vi "UNITEST MAIN v01.3.vi"() -> ()   [LabVIEW 2025]
uses:
  controls/LAB-IQ UI Data.ctl
  HEAVE vi's/Heave Write enum.ctl
  487e97dd-ad82-4ea8-9260-f35915b83a37.vi
  fdf22e40-24ec-4bd6-b058-052306f15f2c.vi
  02c5850b-52e8-4ed5-91f8-6f0ad62f4994.vi
  1223eb78-e4c4-4b69-bf80-185c82055158.vi
  e5651a45-6a49-4a3f-b503-ff1eaf449b4a.vi
  support/Message Queue/Enqueue Message (Single).vi
  <vilib>/Utility/error.llb/Error Cluster From Error Code.vi
  <vilib>/ErrorRing/Error Ring.xnode
  support/Message Queue/LAB-IQ Message Queue.lvlib
  support/User Event - Stop/LAB-IQ User Event - Stop.lvlib
  d081153b-36ca-4bc4-8478-749476f82ba4.vi
  HEAVE vi's/Heave Right enum.ctl
panel:
  in  "Checkbox":bool
  in  "seconds to wait":dbl=0.0001 format="%#_6p"
  out "error out":errorcluster
  in  "error in (no error)":errorcluster
  out "Heave and Surge Read":string
  in  "min_finetune_floor":dbl=0.15
  in  "min_deadband_floor":dbl=0.05
  in  "fine_tune_pct":dbl=100.0
  out "Start Test Temp":bool
  in  "STOP":bool
  in  "AppLoadSeq scratch":bool
  out "Pulse delta":dbl
  in  "Fine Tune Zone":dbl=10.0
  in  "PID Delay (sec)":dbl=1.0 format="%#_6p"
  in  "Max_pos_limit":dbl=50000000.0
  in  "Min_pos_limit":dbl
  in  "i_limit":dbl=10.0
  in  "Max Step Linit":dbl=10.0
  in  "Init Step":dbl=10.0
  in  "pct_scale":dbl=100.0
  in  "Deadband":dbl=0.1
  in  "Kd":dbl
  in  "Ki":dbl
  in  "Kp":dbl=1.0
  out "Current Position":dbl
  in  "Set Load":dbl
  in  "Current Load":dbl
  in  "Manual Write Heave & Surge":bool
  out "Heave and Surge Write":string
  in  "Heave Loop Delay":dbl
  in  "Heave PID Speed":dbl=15.0
  in  "Surge Jog Speed":dbl=1.0 format="%.4f"
  in  "Heave Jog Speed":dbl=15.0
  in  "SPARE 4":u8
  in  "SPARE 3":u8
  in  "SPARE 2":u8
  in  "SPARE 1":u8
  out "Spare 15":u8
  out "Spare 14":u8
  out "Spare 13":u8
  out "Spare 12":u8
  out "Spare 11":u8
  out "Spare 10":u8
  out "Spare 9":u8
  out "Spare 8":u8
  out "Spare 7":u8
  out "Spare 6":u8
  out "Spare 5":u8
  out "Spare 4":u8
  out "Spare 3":u8
  out "Spare 2":u8
  out "Spare 1":u8
  out "Node Id":u8
  out "Read Heave Temp":bool
  out "fwMinor":u8
  out "fwMajor":u8
  out "faultCode":u16
  out "SURGE POSE":sgl format="%#.6f"
  out "HEAVE POSE":sgl format="%#.6f"
  out "Homed":u8
  out "State":u8
  out "Ack ID":u16
  in  "SPEED":sgl=10000.0
  in  "Distance":sgl=10000.0
  in  "Mode Command":u8=2
  out "Sequence ID":u16
  out "error out Read":errorcluster
  out "error out Write":errorcluster
  out "Heave and Surge Read":string
  out "Load Cell Temp":bool
  in  "Stop Scratch":bool
  in  "Enter Fixed SRR 2":dbl min=0.0 max=0.0 format="%.3f"
  in  "E.Velocity 2":bool=TRUE caption="SRR"
  out "Message":string="Load Entered is out of range!!!"
  in  "Tab Control 3":T1(tab)
  in  "Tab Control 5":enum32{""}(tab)
  in  "Tab Control 14":T2(tab)=enum."Motor Load"
  in  "Ramp MulFac":dbl=2.0
  in  "pulses LoadDiffRamp(2..10)":dbl=9.0
  in  "PulseControlRamp(diff<=3N)":dbl=5.0 min=1.0 max=1000.0 step=1.0 format="%#.1f"
  in  "SetLoadDeadband(%) Load(0-10N)":dbl=0.1 min=0.0001 max=100.0 step=0.0001 format="%#.6f"
  in  "PID gains out delay (microForce)":T3={"proportional gain (Kc)"=300.0, "integral time (Ti, min)"=0.00011, "derivative time (Td, min)"=0.0} {"derivative time (Td, min)" format="%.3f"; "integral time (Ti, min)" min=1e-05 max=100.0 step=1e-06 format="%.6f"; "proportional gain (Kc)" format="%.3f"}
  in  "Ramp":bool
  in  "Gain 2":dbl=0.016
  in  "pulses LoadDiff(2..10)":dbl=10.0
  in  "pulses LoadDiff(11..50)":dbl=40.0
  in  "PulseControl(diff<=3N)":dbl=1.0 min=1.0 max=1000.0 step=1.0 format="%#.1f"
  out "SetLoadDeadband(%)  2":dbl=1.0 min=0.001 max=100.0 step=0.001 format="%#.6f"
  in  "Dummy Run":bool
  out "Vertical load (N)":dbl format="%#.3f"
  in  "AutoTune":bool
  in  "Offset  3":dbl=1.5
  in  "apply load":bool
  in  "Enter ByPass Load":dbl
  in  "reinit 3":bool=TRUE
  in  "output range delay":cluster{"output high":dbl, "output low":dbl}={"output high"=100.0, "output low"=-100.0} {"output low" format="%.2f"; "output high" format="%.2f"}
  in  "PID gains out delay":T3={"proportional gain (Kc)"=30.0, "integral time (Ti, min)"=0.00101, "derivative time (Td, min)"=0.0} {"derivative time (Td, min)" format="%.3f"; "integral time (Ti, min)" min=1e-05 max=100.0 step=0.0001 format="%.4f"; "proportional gain (Kc)" format="%.3f"}
  in  "Bypass Load":bool
  in  "pulsesSent":dbl=200.0
  out "pulses":dbl
  out "actpid":dbl
  out "gFF Rot 7":cluster{dbl, dbl, dbl}(graph)
  in  "pulses LoadDiff(21..1000)":dbl=40.0
  in  "Delay":dbl=1.5 min=0.001 max=5.0 step=0.001 format="%#.6f"
  in  "deadband":dbl=0.2
  in  "Tab Control 26":enum32{"Page 1", "Page 2"}(tab)
  in  "ClearAll":bool
  out "Mz(Nm)":dbl[](array[numeric])
  out "My(Nm)":dbl[](array[numeric])
  out "Mx(Nm)":dbl[](array[numeric])
  in  "Save Dwell":dbl=0.015 caption="Save Dwell (sec)" min=0.0 max=5.0 step=0.001 format="%.3f"
  out "Mx":dbl[](graph)
  out "My":dbl[](graph)
  out "Mz":dbl[](graph)
  out "Fx(N)":dbl[](graph)
  out "Fy(N)":dbl[](graph)
  out "Fz(N)":dbl[](graph)
  in  "ZeroAll":bool
  in  "Acq Delay (ms)":dbl=10.0
  in  "Burst Delay (ms)":dbl=10.0
  out "model":string
  out "SN":i32
  out "FFx(N)":dbl[](array[numeric])
  in  "Sensor IP":string="192.168.1.100"
  in  "Port":i32=8080
  out "FFy(N)":dbl[](array[numeric])
  out "Load(N)":dbl[](array[numeric])
  out "AE":bool
  in  "delete Handle":bool
  in  "Create Handle":bool=TRUE
  out "ft_data":dbl[](array[numeric])=[1.0, 1.0, 1.0, 1.0, 1.0, 1.0]
  out "ft_range":dbl[](array[numeric])=[1.0, 1.0, 1.0, 1.0, 1.0, 1.0]
  in  "stop 6":bool
  out "running_flag":bool
  out "ft_udp_handle":i32
  out "get-data-return":i32
  out "get-range-return":i32
  out "zero-return":i32
  out "filter-return":i32
  out "initial-return":i32
  out "deleteHandle-result":i32
  in  "Tab Control 19":enum32{"Platform COM", "Config ", "DevInfo"}(tab)=enum."Config "
  in  "SAMPLES":dbl=100.0
  in  "Re-initilaize":bool
  in  "Filter ON/OFF":bool=TRUE
  in  "TracHomeSurgeOffsetCounts 10MM":dbl=505100.0
  in  "TracHomeSwayOffsetCounts 10MM":dbl=1432.0
  in  "Acoustic Emission:":dbl=1.0 min=0.0001 max=200.0 step=0.0001 format="%.4f"
  in  "Apply Filter (FF)":bool
  in  "Filter% 2":dbl=50.0 min=50.0 max=100.0 step=0.1 format="%.1f"
  in  "Apply Filter (Load)":bool=TRUE
  in  "Filter%":dbl=80.0 min=50.0 max=100.0 step=0.1 format="%.1f"
  in  "Sway distance (mm)":dbl=245.0
  in  "Surge distance (mm)":dbl=370.0
  in  "DataSavingLoopDelay(ms)":dbl=15.0
  in  "SAVE  2":bool
  in  "Enter Distance":bool caption="Enter Counts"
  in  "Sway Counts:":dbl=100.0 min=0.0 max=100000000.0 step=1.0 format="%.2f"
  in  "Distance (mm): 3":dbl=100.0 caption="Distance (mm):" min=0.0 max=1500.0 step=0.001 format="%.5f"
  in  "Surge Counts:":dbl=100.0 min=0.0 max=100000000.0 step=1.0 format="%.1f"
  in  "Distance (mm): 2":dbl=100.0 caption="Distance (mm):" min=0.0 max=1500.0 step=0.0001 format="%.3f"
  in  "Distance (mm):":dbl=100.0 min=0.0 max=1500.0 step=0.001 format="%.5f"
  in  "Heave Counts:":dbl=100.0 min=0.0 max=100000000.0 step=1.0
  in  "LRMHomeSurgeOffsetCounts":dbl=307197.0
  in  "LRMHomeSwayOffsetCounts":dbl=26880.0
  in  "TracHomeSurgeOffsetCounts 20MM":dbl=505100.0
  in  "TracHomeSwayOffsetCounts 20MM":dbl=1432.0
  in  "RotHomeSwayOffsetCounts":dbl=14656.0
  in  "RotHomeSurgeOffsetCounts":dbl=311465.0
  in  "Heave distance":dbl=340.0
  out "Zmm":dbl=1600.0
  out "Heave Pulses/mm":dbl=1600.0
  out "Surge Pulses/mm":dbl=1600.0
  out "Sway Pulses/mm":dbl=320.0
  in  "Heave Pitch":dbl=4.0
  in  "Surge Pitch":dbl=3.0
  in  "Sway Pitch":dbl=2.0
  in  "Heave PPR":dbl=6400.0
  in  "Surge PPR":dbl=6400.0
  in  "Sway PPR":dbl=6400.0
  in  "GUI":T4(tab)
  in  "Platform Settings":bool caption="Password"
  in  "Configure":bool caption="Password"
  in  "Home":bool caption="Password"
  in  "EXIT":bool
  in  "Analysis":bool caption="Password"
  in  "service 2":bool caption="Password"
  in  "MainPage":T5(tab)=enum."HOME"
  in  "Select Load Head":bool
  in  "Notes :":string
  in  "FILE":string
  in  "Sample ID :":string
  in  "Operator ID :":string
  in  "Operator Name :":string
  in  "Auto":bool caption="Power Status"
  out "mm/s  Surge":dbl=7.0 caption="Jog" min=0.001 max=50.0 step=0.0001 format="%.2f"
  in  "Update Surge Speed":bool
  out "Drive Error":string
  in  "Disable Axis Jog Soft Limits":bool
  out "mm/s  Sway":dbl=7.0 caption="Jog" min=0.001 max=50.0 step=0.0001 format="%.2f"
  out "Sway and Surge COM Status":bool=TRUE caption="Load COM Status"
  out "Heave COM Status":bool=TRUE caption="Load COM Status"
  in  "Enable Platform":bool
  in  "Surge Forward Main":bool
  in  "Surge Backward Main":bool
  in  "Sway Right Main":bool
  in  "Sway Left Main":bool
  in  "Heave Down Main":bool
  in  "Heave Up main":bool
  in  "Update Sway Speed":bool
  in  "Update Heave Speed":bool
  out "mm/s Heave":dbl=7.0 caption="Jog" min=0.001 max=30.0 step=0.0001 format="%.2f"
  in  "mm/sec":dbl=1.0 caption="Jog" min=0.001 max=50.0 step=0.001 format="%.2f"
  in  "mm":dbl=0.001 caption="Jog" min=0.001 max=200.0 step=0.0001 format="%#.3f"
  in  "Surface Analysis":bool
  in  "Imaging":bool
  in  "Image Analysis":bool
  in  "Post Analysis":bool
  in  "SSP 0.75":bool
  in  "SSP 0.5":bool
  in  "SSP 0.3":bool
  in  "Warning":enum32{"Page 2"}(tab)
  in  "gui GIF":enum32{"Check", "Deca", "kilo", "Micro"}(tab)
  out "Communication is established":bool=TRUE caption="Load COM Status"
  in  "Reference Sample":u16(ring) items=["None", "Brass", "Aluminium", "Mild Steel"]
  out "Load Cell Communication Slide":u8(slide)=1 min=1 max=10 step=1 scale=0.0..10.0
  in  "com 3":bool
  out "com":bool
  out "DecaForce COM Status":bool caption="Load COM Status"
  in  "Loading Mode":u16(ring) items=["Constant", "Ramp", "Steps", "Indentation"]
  in  "Enter the CoF Trip":dbl=1.0
  in  "Enter the Friction Force Trip":dbl=520.0 min=500.0 max=500.0 step=1.0 format="%#.1f"
  in  "Enter the Normal load Trip":dbl=520.0 min=500.0 max=500.0 step=0.001 format="%.3f"
  in  "KiloForce":bool
  in  "DecaForce":bool
  in  "MicroForce":bool
  in  "LHBack":bool
  in  "LHNext":bool
  in  "Load Selection":T6(tab)
  in  "Enter the Load  (N)":dbl=2.0 min=2.0 max=50.0 step=0.1 format="%#.4f"
  in  "Enter the Final Load (N)":dbl=1.0 min=0.0 max=500.0 step=1.0 format="%#.0f"
  in  "Update":bool
  in  "Enter the Loading Rate (N/min)":dbl=60.0 min=60.0 max=1200.0 step=0.1 format="%.2f"
  out "Warning 2":bool
  in  "Stribeck Table  For loading":string[][](table)=[["", "", ""], ["", "", ""], ["", "", ""], ["", "", ""]]
  in  "Stribeck table":bool
  in  "seq":bool=TRUE
  in  "Clear 3":bool
  in  "Indentation":string[][](table)=[["Detection", "5", "2"], ["Unload", "0", "5"], ["Load", "10", "2"], ["Unload", "0", "5"], ["Detection", "5", "2"], ["Unload", "0", "5"]]
  in  "Multipoint":bool caption="Singlepoint"
  in  "AppLoad 4":bool
  in  "zNL":bool
  out "NL disp":dbl caption="Normal Load ( N )" min=-2000.0 max=2000.0 step=0.0001 format="%.1f"
  in  "Traction":bool
  in  "Surge Forward MM":bool
  in  "Surge Backward MM":bool
  in  "M3 Image":enum32{"Page 1", "Page 2"}(tab)
  in  "String 39":string="Jog heave to bring the upper sample closer to the lower sample within 1mm."
  in  "Sway Left MM":bool
  in  "Sway Right MM":bool
  in  "Disable Axis Jog Soft Limits":bool
  in  "mm":dbl=0.001 caption="Jog" min=0.001 max=5.0 step=0.0001 format="%#.3f"
  in  "Heave Down MM":bool
  in  "Heave Up MM":bool
  in  "Wear Track Diameter (mm)":dbl=5.0 caption="Wear Track Diameter (mm):" min=1.0 max=30.0 step=1.0 format="%.2f"
  in  "Set WTD":bool
  in  "HomeScratch":bool
  in  "HomeRot":bool
  in  "PlaceModule":bool
  in  "Motion Mode:":u16(ring) items=["Uniform Rotation", "Angular Oscillation", "Stribeck ", "Steps"]
  in  "LR Sway":bool
  in  "Rot Hor":bool
  in  "Rot Ver":bool
  in  "Scratch":bool
  in  "LR Cam":bool
  in  "MMBack":bool
  in  "MMNext":bool
  in  "Rotary Module Selection":T7(tab)
  in  "SPEED SELECTION :":enum32{"Speed in RPM", "Speed in m/sec"}(radio)=enum."Speed in m/sec"
  in  "TEST SELECTION":enum32{"Time", "Cycle"}(radio)
  in  "Enter the Speed(mm/sec)":dbl=1.0 min=0.1 max=10.0 step=0.1 format="%.1f"
  in  "Enter the Speed(RPM)":dbl=45.0 min=5.0 max=300.0 step=1.0
  in  "Enter the Frequency (Hz)":dbl=1.0 min=0.1 max=10.0 step=0.1 format="%.1f"
  in  "Enter the Angle (Deg)":dbl=45.0 min=5.0 max=300.0 step=1.0
  in  "Angular Oscillation Set":bool
  in  "Rotary Tab":enum32{"Page 1", "Page 2"}(tab)
  out "e.v/ssr 2":enum32{"E.V", "SSR"}(tab)
  in  "Enter the Final E.Velocity (m/s) 2":dbl=1.0 min=0.001 max=4.0 step=0.001 format="%.3f"
  in  "Enter initial E.Velocity (m/s) 2":dbl=2.0 min=0.001 max=4.0 step=0.001 format="%.3f"
  in  "Enter Fixed E.Velocity 2":dbl=1.0 min=0.001 max=2.0 step=0.001 format="%.3f"
  in  "Enter Final SRR 2":dbl=1.0 min=0.001 max=1.0 step=0.001 format="%.2f"
  in  "Enter initial SRR 2":dbl=1.0 min=0.001 max=1.0 step=0.001 format="%.2f"
  out "Final Speed (RPM) 3":dbl=1.0 min=0.1 max=3000.0 step=0.1 format="%.1f"
  out "Initial Speed (RPM) 2":dbl=100.0 min=0.1 max=3000.0 step=0.1 format="%.1f"
  in  "Enter the Final Velocity (m/s) 3":dbl=1.0 min=0.001 max=2.0 step=0.001 format="%.3f"
  in  "Enter initial Velocity (m/s)  3":dbl=2.0 min=0.001 max=2.0 step=0.001 format="%.3f"
  out "Ramp Up 2":bool caption="Ramp Down"
  in  "File Path :  2":path
  in  "Import 2":bool
  in  "Save 2":bool
  in  "SPEED SELECTION : rotary":enum32{"Speed in Rpm", "Speed in m/sec"}(radio)=enum."Speed in m/sec"
  in  "calculate rotary":bool
  in  "String 45":string="File Path Location : C:-->LAB-IQ 150 --> User Defined\n                                       Protocol-->File.txt"
  in  "Step Speed":enum32{"Step Speed", "Step (load-Speed)"}(tab)
  in  "StepTable For Speed":string[][](table)=[["", "", ""], ["", "", ""], ["", "", ""], ["", "", ""]]
  in  "StepTable For Load-Speed":string[][](table)=[["", "", ""], ["", "", ""], ["", "", ""], ["", "", ""]]
  in  "StepTable For Speed 3":string[][](table)=[["", "", ""], ["", "", ""], ["", "", ""], ["", "", ""]]
  in  "Motion Direction:  3":u16(ring) items=["Clockwise", "Counter Clockwise"]
  out "Humidity  Status  3":bool caption="Communication Status"
  out "Low Temp  Status  2":bool caption="Communication Status"
  out "TK4 status 2":bool caption="Communication Status"
  in  "String 40":string="Before selecting Acoustic make sure the sensor output pin is connected to A4."
  in  "Stage Temperature":dbl[](array[numeric])=[150.0, 230.0, 300.0, 350.0, 400.0, 450.0, 500.0]
  in  "Sample Temperature":dbl[](array[numeric])=[100.0, 150.0, 200.0, 250.0, 300.0, 350.0, 400.0]
  in  "Humidity (Amb)":bool
  in  "Clear List":bool
  out "Sensors Picked":string
  in  "Add to list":bool
  in  "Wear":bool
  in  "Vibration":bool
  in  "Humidity (Chamber)":bool
  in  "Temperature (Chamber)":bool
  in  "ECR":bool
  in  "Temperature (Amb)":bool
  in  "Microphone":bool
  in  "Acoustic Emission 3":bool
  in  "SNext":bool
  in  "APBack":bool
  in  "Enter the Temperature (°C):":dbl
  in  "Enter the Stage \nTemperature (°C):":dbl=20.0 min=20.0 max=150.0 step=1.0 format="%#.0f"
  in  "Enter the Humidity (%Rh):":dbl=30.0 min=30.0 max=85.0 step=1.0
  in  "Low Temp":bool
  in  "High Temp":bool
  in  "Humidity":bool
  in  "Main Screen Tab":T8(tab)
  in  "ClrLog":bool
  out "Trip Log":string
  in  "Start Test":bool
  out "Test status":bool caption="Test Status"
  out "AR Led":bool caption="AR"
  out "Data":bool=TRUE
  out "Health":bool=TRUE
  out "Sway COM Status":bool=TRUE caption="Load COM Status"
  out "Heave COM Status":bool=TRUE caption="Load COM Status"
  in  "Grp Tab":enum32{"Rot/LRM", "FBT"}(tab)
  in  "Sub Graph":T9(tab)
  in  "Speed Reset Graph":bool
  in  "Speed Tab":enum32{" Rotary Disc", "MTM Ball", "MTM Disc"}(tab)
  out "speed mm/sec":dbl(graph)=0.13298760003255525
  out "MTM BALL SPEED":dbl(graph)=0.13298760003255525
  out "MTM DISC  SPEED":dbl(graph)=0.13298760003255525
  in  "Temperature Reset":bool
  out "Temperature (deg c)":dbl(graph)=0.13298760003255525
  in  "ECR RESET":bool
  out "ECR":dbl(graph)=0.13298760003255525
  out "Acoustic Emission (mV)":dbl min=0.0 max=5000.0 step=0.1
  in  "Aqucostic Reset Graph":bool
  out "gACQUOS":dbl(graph)=0.13298760003255525
  in  "Humidity Reset Graph":bool
  out "HumrGp":dbl(graph)=0.13298760003255525
  out "SD (mm)":dbl caption="Sliding Distance ( mm )" min=-200.0 max=200.0 step=0.1 format="%.4f"
  in  "Siliding distance Reset Graph":bool
  out "SDGp":dbl(graph)=0.13298760003255525
  out "Hymidity":bool
  in  "Humidity Disable trip":bool=TRUE
  in  "CoF Trip  2":dbl=540.0 min=100.0 max=540.0 step=1.0
  out "Depth Trip":dbl=600.0
  in  "Depth Trip":bool=TRUE
  out "Weart Deapth":bool
  in  "Depth Reset Graph":bool
  out "Weart":bool
  in  "Depthz":bool
  out "Depth (µm)":dbl min=-200.0 max=200.0 step=0.1 format="%.1f"
  out "WearGp":dbl(graph)=0.13298760003255525
  out "NL Trip 2":dbl=600.0
  out "Load pid":bool
  in  "Load Disable Trip":bool=TRUE
  in  "Load Reset Graph":bool
  out "NL Display 4":dbl caption="Normal Load ( N )" min=-2000.0 max=2000.0 step=0.0001 format="%.1f"
  out "Main Chart 3":cluster{dbl, "NL disp":dbl, dbl}(graph)
  in  "FF Tab":T10(tab)
  in  "COF Reset Graph":bool
  in  "COF Disable Trip":bool=TRUE
  out "COF TRIP":dbl=600.0
  out "COF MAIN CHART":cluster{dbl, "NL disp":dbl, dbl}(graph)
  out "Friction Force (N)":dbl min=-2000.0 max=2000.0 step=0.0001 format="%.1f"
  in  "FF Reset Graph":bool
  in  "FF Disable Trip":bool=TRUE
  out "FF TRIP":dbl=600.0
  out "FF MAIN CHART":cluster{dbl, "NL disp":dbl, dbl}(graph)
  in  "BACK":bool
  out "Ambient \nTemperature":dbl min=0.0 max=5000.0 step=0.1 format="%.1f"
  out "Ambient\n Humidity":dbl min=0.0 max=5000.0 step=0.1 format="%.2f"
  out "NL disp 2":dbl caption="Normal Load ( N )" min=-2000.0 max=2000.0 step=0.0001 format="%.1f"
  out "Set Humidity":dbl caption="Set Humidity  (% Rh)" min=-2000.0 max=2000.0 step=1.0 format="%.1f"
  out "humidity disp":dbl caption="Humidity (% Rh)" min=-2000.0 max=2000.0 step=1.0 format="%.1f"
  in  "Humidity On":bool
  in  "zNL 2":bool
  out "NLt":bool
  in  "Load En":bool
  out "Freq (Hz)":dbl min=0.0 max=5000.0 step=0.1 format="%.4f"
  out "HumCOMStatus":bool caption="Communication Status"
  out "Load Communication":bool
  in  "Temp Tabs":enum32{"Low Temp", "High Temp"}(tab)=enum."High Temp"
  out "Controller  Status":bool
  out "ChamberTemp":dbl format="%#.1f"
  in  "SetTmp":dbl=-190.0 caption="Set Temperature (Deg C)" min=-190.0 max=100.0 step=1.0 format="%.1f"
  in  "Cooling":bool
  in  "Heater":bool
  out "TK4 status":bool caption="Controller  Status"
  out "ChamberTemp":dbl format="%#.1f"
  in  "SetTmp":dbl caption="Set Temperature (Deg C)" min=0.0 max=1000.0 step=1.0 format="%.1f"
  in  "Set Load (N)":dbl=100.0 min=0.01 max=1500.0 step=0.01 format="%.1f"
  in  "Time Tab":enum32{"cycles", "duration"}(tab)=enum."duration"
  out "Test Duration 4":dbl=600.0 caption="Test Duration\n(HH:MM:SS)" min=0.0083 max=180000.0 step=0.0001 format="%<%H:%M:%S>t"
  out "TEST CYCLE":dbl min=0.0 max=5000.0 step=0.01 format="%.2f"
  in  "TOTAL CYCLES":dbl min=0.0 max=5000.0 step=0.1 format="%.4f"
  out "Time ( HH:MM:SS ) 2":dbl min=0.0 max=144000.0 step=1.0 format="%<%H:%M:%S>t"
  in  "Test Duration":dbl=600.0 caption="Test Duration\n(HH:MM:SS)" min=0.0083 max=180000.0 step=0.0001 format="%<%H:%M:%S>t"
  in  "Main Speed Tab":enum32{"ROTARY", "TRACTION"}(tab)
  in  "SPEED TAB":enum32{"RPM", "m/sec"}(tab)
  out "Speed (RPM)":dbl min=0.0 max=5000.0 step=0.1 format="%.1f"
  out "Set Speed":dbl caption="Set Speed (RPM)" min=0.0 max=1500.0 step=0.1 format="%.1f"
  out "Speed (m/sec)":dbl min=0.0 max=5000.0 step=0.001 format="%.4f"
  out "Set Speed (m/sec)":dbl min=0.0 max=1500.0 step=0.001 format="%.4f"
  in  "MTM MOTOR DISPLAY":enum32{"MTM RPM", "MTM m/sec"}(tab)
  out "Disc Speed (RPM)":dbl min=0.0 max=1500.0 step=0.1 format="%.1f"
  out "Ball Speed (RPM)":dbl min=0.0 max=1500.0 step=0.1 format="%.1f"
  out "Disc Speed (m/sec)":dbl min=0.0 max=1500.0 step=0.1 format="%.1f"
  out "Ball Speed (m/sec)":dbl min=0.0 max=1500.0 step=0.1 format="%.1f"
  in  "Angle and Frequency":enum32{"angular", "lrm"}(tab)
  out "Angle (Deg)":dbl min=0.0 max=5000.0 step=0.01 format="%.2f"
  out "Stroke (mm)":dbl min=0.0 max=5000.0 step=0.01 format="%.2f"
  in  "Analysis Home":bool
  in  "Password":string
  in  "Home Service":bool
  in  "Advanced Setting":bool
  in  "About Tab":enum32{"Primary"}(tab)
  in  "ECR Port:":refnum<visa-resource-name>="COM10"
  in  "Ramp Port:":refnum<visa-resource-name>="COM10"
  in  "Installation/Replacement completed":bool
  in  "Loahead":bool
  in  "Heave and Surge COM Port:":refnum<visa-resource-name>="COM9"
  in  "Sway COM Port:":refnum<visa-resource-name>="COM10"
  in  "Temp Modbus:":refnum<visa-resource-name>="COM14"
  in  "Humidity Port:":refnum<visa-resource-name>="COM10"
  in  "Edit Gain Constants":bool
  in  "Save Gain Constants":bool
  in  "Service About":bool
  # "load Aquisition off"
  # "load Aquisition On"
  # "Configuration"
  # "Limits for Heave Surge and Sway"
  # "Modules Offset Parameters"
  # "Counts-Distance Calculator"
  # "File Name :"
  # "Ensure the traction module is aligned\n horizontally with the stage before ENABLE."
  # "SET JOG SPEED"
  # "JOG MODE"
  # "Module Selection"
  # "Positioning Control"
  # "Connect the controller\ncable to M3"
  # "Environment"
  # "Sensors"
  # "Data Points"
  # "Data Points"
  # "Data Points"
  # "Data Points"
  # "ohms"
  # "Data Points"
  # "Data Points"
  # "Data Points"
  # "LAB-IQ 150 / UNITEST / WO2456 / UT150  v05 / AUGUST 2025"
  # "NOTE: This operation needs to be done only when the machine is ON."
types:
  T1 = enum32{"Advanced", "Motor", "Depth_graph", "UIO Communicator", "Add to list parametrs", "Instrument Functions", "BURST FILE SAVE"}
  T2 = enum32{"LRM heating", "FBT_Heating", "Motor Load", "Loadcell Response", "Voice Load", "Step loading and speed ", "Depth"}
  T3 = cluster{"proportional gain (Kc)":dbl, "integral time (Ti, min)":dbl, "derivative time (Td, min)":dbl}
  T4 = enum32{"Setup", "Load Head", "Motion Module", "Environment", "Begin"}
  T5 = enum32{"Details", "PlatformSetting", "Analysis", "HOME"}
  T6 = enum32{"Constant", "Ramp", "Step", "Indentation"}
  T7 = enum32{"Uniform Rotation", "Angular Oscillation", "Speed Ramp", "Speed Step"}
  T8 = enum32{"  Acquire  ", "Compare Files Rot", "About", "Service"}
  T9 = enum32{"Speed", "Temperature", "ECR", "Acoustic Emission", "Humidity", "Sliding Distance"}
  T10 = enum32{"Coefficient of Friction ", "Friction Force (N)"}
  T11 = typedef "Heave Write enum.ctl" = enum16{"INIT", "WRITE", "CLOSE", "REINIT"}
  T12 = typedef "LAB-IQ UI Data.ctl" = cluster{"Main Home Screen":cluster{"GUI":refnum<vi>, "Platform Settings":refnum<vi>, "Configure":refnum<vi>, "Home":refnum<vi>, "EXIT":refnum<vi>, "service 2":refnum<vi>, "MainPage":refnum<vi>, "Analysis":refnum<vi>}, "Platform Settings":cluster{"mm/s  Surge":refnum<vi>, "Update Surge Speed":refnum<vi>, "Drive Error":refnum<vi>, "Disable Axis Jog Soft Limits":refnum<vi>, "mm/s  Sway":refnum<vi>, "Sway and Surge COM Status":refnum<vi>, "Heave COM Status":refnum<vi>, "Enable Platform":refnum<vi>, "Surge Forward Main":refnum<vi>, "Sway Right Main":refnum<vi>, "Sway Left Main":refnum<vi>, "Heave Down Main":refnum<vi>, "Heave Up main":refnum<vi>, "Update Sway Speed":refnum<vi>, "Update Heave Speed":refnum<vi>, "mm/s Heave":refnum<vi>, "mm/sec":refnum<vi>, "mm":refnum<vi>, "Surge Backward Main":refnum<vi>}, "Analysis Screen":cluster{"Analysis Home":refnum<vi>, "Surface Analysis":refnum<vi>, "Imaging":refnum<vi>, "Image Analysis":refnum<vi>, "Post Analysis":refnum<vi>}, "Config Screen":cluster{"Select Load Head":refnum<vi>, "Notes :":refnum<vi>, "FILE":refnum<vi>, "Sample ID :":refnum<vi>, "Operator ID :":refnum<vi>, "Operator Name :":refnum<vi>, "Auto":refnum<vi>}, "Motion Module":cluster{"zNL":refnum<vi>, "NL disp":refnum<vi>, "Rotary Tab":refnum<vi>, "Motion Direction:  3":refnum<vi>, "E.Velocity 2":refnum<vi>, "e.v/ssr 2":refnum<vi>, "Enter Fixed E.Velocity 2":refnum<vi>, "Enter Final SRR 2":refnum<vi>, "Enter initial SRR 2":refnum<vi>, "Enter Fixed SRR 2":refnum<vi>, "Enter the Final E.Velocity (m/s) 2":refnum<vi>, "Enter initial E.Velocity (m/s) 2":refnum<vi>, "Final Speed (RPM) 3":refnum<vi>, "Initial Speed (RPM) 2":refnum<vi>, "Enter the Final Velocity (m/s) 3":refnum<vi>, "Enter initial Velocity (m/s)  3":refnum<vi>, "Ramp Up 2":refnum<vi>, "TEST SELECTION":refnum<vi>, "SPEED SELECTION : ":refnum<vi>, "Angular Oscillation Set":refnum<vi>, "Traction":refnum<vi>, "Step Speed":refnum<vi>, "StepTable For Load-Speed":refnum<vi>, "StepTable For Speed":refnum<vi>, "Surge Forward MM":refnum<vi>, "Surge Backward MM":refnum<vi>, "M3 Image":refnum<vi>, "String 39":refnum<vi>, "Sway Left MM":refnum<vi>, "Sway Right MM":refnum<vi>, "Disable Axis Jog Soft Limits":refnum<vi>, "mm":refnum<vi>, "Heave Down MM":refnum<vi>, "Heave Up MM":refnum<vi>, "Wear Track Diameter (mm)":refnum<vi>, "Set WTD":refnum<vi>, "HomeScratch":refnum<vi>, "HomeRot":refnum<vi>, "PlaceModule":refnum<vi>, "Enter the Angle (Deg)":refnum<vi>, "Enter the Frequency (Hz)":refnum<vi>, "Motion Mode:":refnum<vi>, "LR Sway":refnum<vi>, "Rot Hor":refnum<vi>, "Scratch":refnum<vi>, "LR Cam":refnum<vi>, "MMBack":refnum<vi>, "MMNext":refnum<vi>, "Rot Ver":refnum<vi>, "Rotary Module Selection":refnum<vi>, "calculate rotary":refnum<vi>, "SPEED SELECTION : rotary":refnum<vi>, "Import 2":refnum<vi>, "Save 2":refnum<vi>, "File Path :  2":refnum<vi>, "String 45":refnum<vi>, "StepTable For Speed 3":refnum<vi>, "Enter the Speed(mm/sec)":refnum<vi>, "Enter the Speed(RPM)":refnum<vi>}, "Environmental control":cluster{"Humidity  Status  3":refnum<vi>, "Low Temp  Status  2":refnum<vi>, "TK4 status 2":refnum<vi>, "Stage Temperature":refnum<vi>, "Sample Temperature":refnum<vi>, "Humidity (Amb)":refnum<vi>, "Clear List":refnum<vi>, "Add to list":refnum<vi>, "Wear":refnum<vi>, "Vibration":refnum<vi>, "Humidity (Chamber)":refnum<vi>, "Temperature (Chamber)":refnum<vi>, "ECR ":refnum<vi>, "Temperature (Amb)":refnum<vi>, "Microphone":refnum<vi>, "Acoustic Emission 3":refnum<vi>, "SNext":refnum<vi>, "APBack":refnum<vi>, "Enter the Temperature (°C):":refnum<vi>, "Enter the Stage \nTemperature (°C):":refnum<vi>, "Enter the Humidity (%Rh):":refnum<vi>, "Low Temp":refnum<vi>, "High Temp":refnum<vi>, "Humidity":refnum<vi>, "Sensors Picked":refnum<vi>}, "About Screen":cluster{"Password":refnum<vi>, "Home Service":refnum<vi>, "Advanced Setting":refnum<vi>, "About Tab":refnum<vi>, "ECR Port:":refnum<vi>, "Ramp Port:":refnum<vi>, "Installation/Replacement completed":refnum<vi>, "Loahead":refnum<vi>, "Heave and Surge COM Port:":refnum<vi>, "Sway COM Port:":refnum<vi>, "Temp Modbus:":refnum<vi>, "Humidity Port:":refnum<vi>, "Edit Gain Constants":refnum<vi>, "Save Gain Constants":refnum<vi>}, "Main Screen":cluster{"Main Screen Tab":refnum<vi>, "Angle and Frequency":refnum<vi>, "Stroke (mm)":refnum<vi>, "Angle (Deg)":refnum<vi>, "Main Speed Tab":refnum<vi>, "MTM MOTOR DISPLAY":refnum<vi>, "Disc Speed (m/sec)":refnum<vi>, "Ball Speed (m/sec)":refnum<vi>, "Disc Speed (RPM)":refnum<vi>, "Ball Speed (RPM)":refnum<vi>, "SPEED TAB":refnum<vi>, "Speed (m/sec)":refnum<vi>, "Set Speed (m/sec)":refnum<vi>, "Speed (RPM)":refnum<vi>, "Set Speed":refnum<vi>, "Time Tab":refnum<vi>, "Time ( HH:MM:SS ) 2":refnum<vi>, "Test Duration":refnum<vi>, "Test Duration 4":refnum<vi>, "TEST CYCLE":refnum<vi>, "TOTAL CYCLES":refnum<vi>, "Set Load (N)":refnum<vi>, "Temp Tabs":refnum<vi>, "Heater":refnum<vi>, "TK4 status":refnum<vi>, "ChamberTemp":refnum<vi>, "SetTmp":refnum<vi>, "Controller  Status":refnum<vi>, "ChamberTemp 2":refnum<vi>, "SetTmp 2":refnum<vi>, "Controller  Status 2":refnum<vi>, "ChamberTemp 3":refnum<vi>, "SetTmp 3":refnum<vi>, "Cooling":refnum<vi>, "Load Communication":refnum<vi>, "Ambient \nTemperature":refnum<vi>, "HumCOMStatus":refnum<vi>, "Ambient\n Humidity":refnum<vi>, "Freq (Hz)":refnum<vi>, "Load En":refnum<vi>, "NLt":refnum<vi>, "zNL 2":refnum<vi>, "Humidity On":refnum<vi>, "humidity disp":refnum<vi>, "Set Humidity":refnum<vi>, "NL disp 2":refnum<vi>, "Humidity On 2":refnum<vi>, "humidity disp 2":refnum<vi>, "Set Humidity 2":refnum<vi>, "NL disp 3":refnum<vi>, "AppLoadSeq scratch":refnum<vi>, "Stop Scratch":refnum<vi>, "ClrLog":refnum<vi>, "Trip Log":refnum<vi>, "STOP":refnum<vi>, "Start Test":refnum<vi>, "Test status":refnum<vi>, "AR Led":refnum<vi>, "Data":refnum<vi>, "Health":refnum<vi>, "Sway COM Status":refnum<vi>, "Heave COM Status":refnum<vi>, "Grp Tab":refnum<vi>, "Sub Graph":refnum<vi>, "SD (mm)":refnum<vi>, "Siliding distance Reset Graph":refnum<vi>, "SDGp":refnum<vi>, "Humidity Reset Graph":refnum<vi>, "HumrGp":refnum<vi>, "Acoustic Emission (mV)":refnum<vi>, "Aqucostic Reset Graph":refnum<vi>, "gACQUOS":refnum<vi>, "ECR RESET":refnum<vi>, "ECR":refnum<vi>, "Temperature Reset":refnum<vi>, "Acoustic Emission (mV) 2":refnum<vi>, "Aqucostic Reset Graph 2":refnum<vi>, "gACQUOS 2":refnum<vi>, "ECR RESET 2":refnum<vi>, "ECR 2":refnum<vi>, "Temperature Reset 2":refnum<vi>, "Temperature (deg c)":refnum<vi>, "Speed Reset Graph":refnum<vi>, "Speed Tab":refnum<vi>, "MTM DISC  SPEED":refnum<vi>, "MTM BALL SPEED":refnum<vi>, "speed mm/sec":refnum<vi>, "Hymidity":refnum<vi>, "Humidity Disable trip":refnum<vi>, "CoF Trip  2":refnum<vi>, "Depth Trip":refnum<vi>, "Weart Deapth":refnum<vi>, "Depth Reset Graph":refnum<vi>, "Weart":refnum<vi>, "Depthz":refnum<vi>, "Depth (µm)":refnum<vi>, "WearGp":refnum<vi>, "NL Trip 2":refnum<vi>, "Load pid":refnum<vi>, "Load Disable Trip":refnum<vi>, "Load Reset Graph":refnum<vi>, "NL Display 4":refnum<vi>, "Main Chart 3":refnum<vi>, "BACK":refnum<vi>, "Depth Trip 2":refnum<vi>, "COF TRIP ":refnum<vi>, "Friction Force (N)":refnum<vi>, "FF Reset Graph":refnum<vi>, "FF Disable Trip":refnum<vi>, "FF TRIP":refnum<vi>, "FF MAIN CHART":refnum<vi>, "COF Disable Trip":refnum<vi>, "COF Reset Graph":refnum<vi>, "COF MAIN CHART":refnum<vi>, "FF Tab":refnum<vi>, "Start Test Temp":refnum<vi>}, "Loading":cluster{"Indentation":refnum<vi>, "Reference Sample":refnum<vi>, "Load Cell Communication Slide":refnum<vi>, "com 3":refnum<vi>, "com":refnum<vi>, "DecaForce COM Status":refnum<vi>, "Update":refnum<vi>, "Clear 3":refnum<vi>, "seq":refnum<vi>, "Stribeck table":refnum<vi>, "Stribeck Table  For loading":refnum<vi>, "Loading Mode":refnum<vi>, "Enter the Final Load (N)":refnum<vi>, "Enter the CoF Trip":refnum<vi>, "Enter the Friction Force Trip":refnum<vi>, "Enter the Normal load Trip":refnum<vi>, "Enter the Load  (N)":refnum<vi>, "KiloForce":refnum<vi>, "DecaForce ":refnum<vi>, "MicroForce":refnum<vi>, "LHBack":refnum<vi>, "LHNext":refnum<vi>, "Enter the Loading Rate (N/min)":refnum<vi>, "Message":refnum<vi>, "Warning 2":refnum<vi>, "SSP 0.75":refnum<vi>, "SSP 0.5":refnum<vi>, "SSP 0.3":refnum<vi>, "Warning":refnum<vi>, "gui GIF":refnum<vi>, "Communication is established":refnum<vi>, "AppLoad 4":refnum<vi>, "Multipoint":refnum<vi>, "Load Selection":refnum<vi>}, "PID":cluster{"Ramp MulFac":refnum<vi>, "pulses LoadDiffRamp(2..10)":refnum<vi>, "PulseControlRamp(diff<=3N)":refnum<vi>, "SetLoadDeadband(%) Load(0-10N)":refnum<vi>, "PID gains out delay (microForce)":refnum<vi>, "Ramp":refnum<vi>, "Gain 2":refnum<vi>, "pulses LoadDiff(2..10)":refnum<vi>, "pulses LoadDiff(11..50)":refnum<vi>, "PulseControl(diff<=3N)":refnum<vi>, "SetLoadDeadband(%)  2":refnum<vi>, "Dummy Run":refnum<vi>, "Vertical load (N)":refnum<vi>, "AutoTune":refnum<vi>, "Offset 3 ":refnum<vi>, "apply load":refnum<vi>, "Offset  3":refnum<vi>, "apply load 2":refnum<vi>, "Enter ByPass Load":refnum<vi>, "reinit 3":refnum<vi>, "output range delay":refnum<vi>, "PID gains out delay":refnum<vi>, "Bypass Load":refnum<vi>, "pulsesSent":refnum<vi>, "pulses ":refnum<vi>, "actpid":refnum<vi>, "gFF Rot":refnum<vi>, "pulses LoadDiff(21..1000)":refnum<vi>, "Delay":refnum<vi>, "deadband":refnum<vi>}, "Config Parameters":cluster{"Tab Control 3":refnum<vi>, "Tab Control 19":refnum<vi>, "SAMPLES":refnum<vi>, "Re-initilaize":refnum<vi>, "Filter ON/OFF":refnum<vi>, "TracHomeSurgeOffsetCounts 10MM":refnum<vi>, "TracHomeSwayOffsetCounts 10MM":refnum<vi>, "Acoustic Emission:":refnum<vi>, "Apply Filter (FF)":refnum<vi>, "Filter% 2":refnum<vi>, "Apply Filter (Load)":refnum<vi>, "Filter% ":refnum<vi>, "Sway distance (mm)":refnum<vi>, "Surge distance (mm)":refnum<vi>, "DataSavingLoopDelay(ms)":refnum<vi>, "SAVE 2":refnum<vi>, "Enter Distance":refnum<vi>, "Sway Counts:":refnum<vi>, "Distance (mm): 3":refnum<vi>, "Surge Counts:":refnum<vi>, "Distance (mm): 2":refnum<vi>, "Distance (mm):":refnum<vi>, "Heave Counts:":refnum<vi>, "LRMHomeSurgeOffsetCounts":refnum<vi>, "LRMHomeSwayOffsetCounts":refnum<vi>, "TracHomeSurgeOffsetCounts 20MM":refnum<vi>, "TracHomeSwayOffsetCounts 20MM":refnum<vi>, "RotHomeSwayOffsetCounts":refnum<vi>, "RotHomeSurgeOffsetCounts":refnum<vi>, "Heave distance":refnum<vi>, "Zmm":refnum<vi>, "Heave Pulses/mm":refnum<vi>, "Surge Pulses/mm":refnum<vi>, "Sway Pulses/mm":refnum<vi>, "Heave Pitch":refnum<vi>, "Surge Pitch":refnum<vi>, "Sway Pitch":refnum<vi>, "Heave PPR":refnum<vi>, "Surge PPR":refnum<vi>, "Sway PPR":refnum<vi>, "Tab Control 5":refnum<vi>, "Tab Control 14":refnum<vi>, "Tab Control 26":refnum<vi>, "AE":refnum<vi>, "Heave Loop Delay":refnum<vi>, "Heave PID Speed":refnum<vi>, "Surge Jog Speed":refnum<vi>, "Heave Jog Speed":refnum<vi>}, "Loading Com Port":cluster{"ClearAll":refnum<vi>, "Mz(Nm)":refnum<vi>, "My(Nm)":refnum<vi>, "Mx(Nm)":refnum<vi>, "Save Dwell":refnum<vi>, "Mx ":refnum<vi>, "My ":refnum<vi>, "Mz":refnum<vi>, "Fx(N)":refnum<vi>, "Fy(N)":refnum<vi>, "Fz(N)":refnum<vi>, "ZeroAll":refnum<vi>, "Acq Delay (ms)":refnum<vi>, "Burst Delay (ms)":refnum<vi>, "model":refnum<vi>, "SN":refnum<vi>, "FFx(N)":refnum<vi>, "Sensor IP":refnum<vi>, "Port":refnum<vi>, "FFy(N)":refnum<vi>, "Load(N)":refnum<vi>, "delete Handle":refnum<vi>, "Create Handle":refnum<vi>, "ft_data":refnum<vi>, "ft_range":refnum<vi>, "ft_data 2":refnum<vi>, "stop 6":refnum<vi>, "running_flag":refnum<vi>, "ft_udp_handle":refnum<vi>, "get-data-return":refnum<vi>, "get-range-return":refnum<vi>, "zero-return":refnum<vi>, "filter-return":refnum<vi>, "initial-return":refnum<vi>, "deleteHandle-result":refnum<vi>, "Load Cell Temp":refnum<vi>}, "Heave AND Surge":cluster{"SURGE POSE":refnum<vi>, "error out Read":refnum<vi>, "HEAVE POSE":refnum<vi>, "State":refnum<vi>, "Homed":refnum<vi>, "Sequence ID":refnum<vi>, "error out Write":refnum<vi>, "faultCode":refnum<vi>, "Ack ID":refnum<vi>, "SPEED":refnum<vi>, "Distance":refnum<vi>, "Mode Command":refnum<vi>, "Heave and Surge Read":refnum<vi>, "Read Heave Temp":refnum<vi>, "Spare 15":refnum<vi>, "Spare 14":refnum<vi>, "Spare 13":refnum<vi>, "Spare 12":refnum<vi>, "Spare 11":refnum<vi>, "Spare 10":refnum<vi>, "Spare 9":refnum<vi>, "Spare 8":refnum<vi>, "Spare 7":refnum<vi>, "Spare 6":refnum<vi>, "Spare 5":refnum<vi>, "Spare 4":refnum<vi>, "Spare 2":refnum<vi>, "Spare 1":refnum<vi>, "Node Id":refnum<vi>, "Spare 3":refnum<vi>, "SPARE 4":refnum<vi>, "SPARE 3":refnum<vi>, "SPARE 2":refnum<vi>, "SPARE 1":refnum<vi>, "fwMajor":refnum<vi>, "fwMinor":refnum<vi>, "Manual Write":refnum<vi>, "Heave and Surge Write":refnum<vi>}, "New PID LOGIC":cluster{"Fine Tune Zone":refnum<vi>, "PID SDelay":refnum<vi>, "Max_pos_limit":refnum<vi>, "Min_pos_limit":refnum<vi>, "i_limit":refnum<vi>, "pct_scale":refnum<vi>, "Deadband":refnum<vi>, "Kd":refnum<vi>, "Ki":refnum<vi>, "Kp":refnum<vi>, "Current Position":refnum<vi>, "Set Load":refnum<vi>, "Current Load":refnum<vi>, "Pulse delta":refnum<vi>, "Init Step":refnum<vi>, "Max Step Linit":refnum<vi>}}
  T13 = typedef "init queue out loop.ctl" = cluster{"UI Loop":refnum<queue>, "LOAD COM LOOP ":refnum<queue>, "SWAY MOTOR COM LOOP":refnum<queue>, "HEAVE MOTOR COM LOOP":refnum<queue>, "TEMPERATURE COM LOOP":refnum<queue>, "RAMP MOTOR COM LOOP":refnum<queue>, "ECR PORT":refnum<queue>, "HUMIDITY COM PORT":refnum<queue>, "PROGRAM LOOP":refnum<queue>, "MONITOR LOOP":refnum<queue>, "REPORT":refnum<queue>, "LOAD PID":refnum<queue>}
  T14 = typedef "Heave Right enum.ctl" = enum16{"INIT", "READ", "CLOSE", "REINIT", ""}
  T15 = enum8{"Enabled", "Disabled", "Disabled and Grayed Out"}
  T16 = enum16{"INIT", "SETLOWPASSFILTER", "SETZERO", "GETSENSORINFO", "GETRANGE", "ZEROALL", "READDATA", "UNINITIAL", "DELETEHANDLE"}
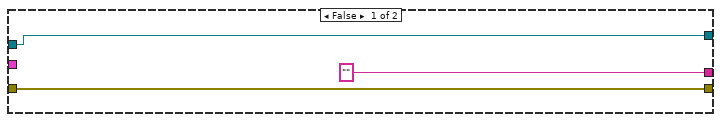
[diagram p2: hidden frame]
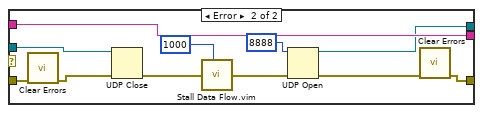
[diagram p3: hidden frame]
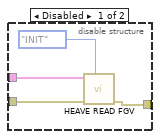
[diagram p4: hidden frame]
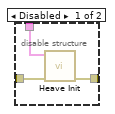
[diagram p5: hidden frame]
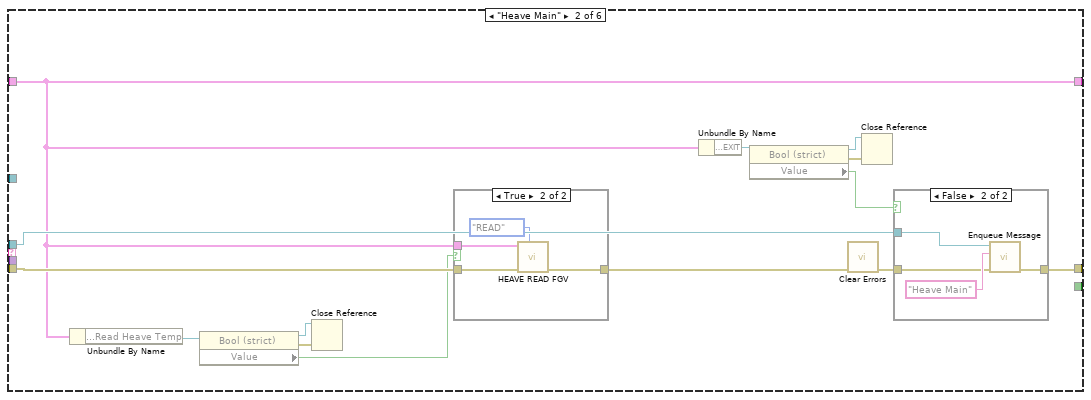
[diagram p6: hidden frame]
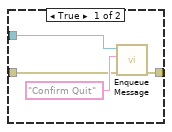
[diagram p8: hidden frame]
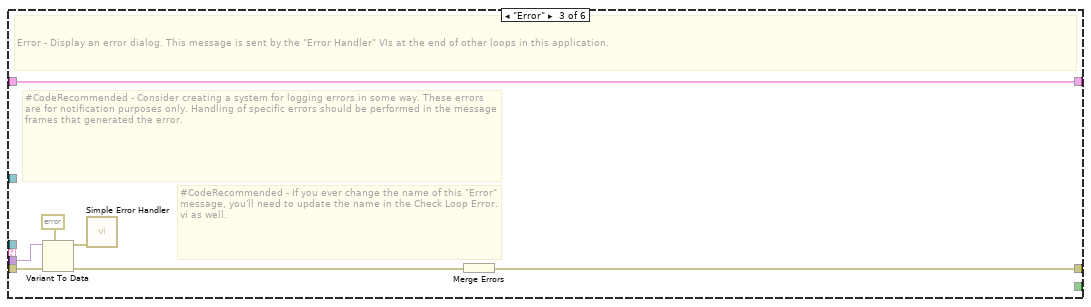
[diagram p9: hidden frame]
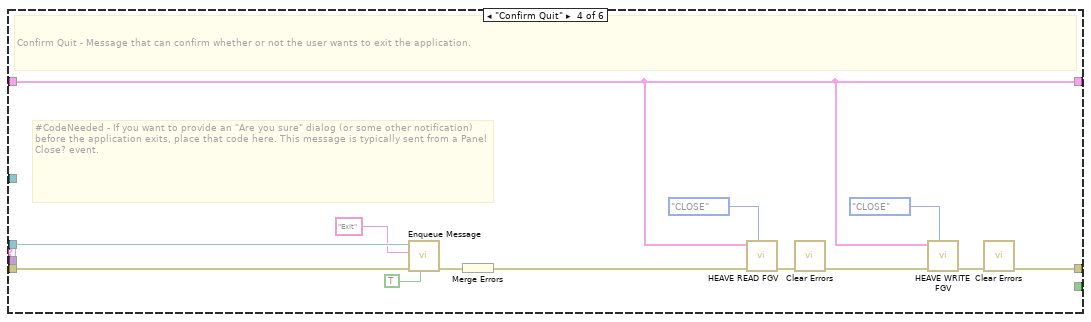
[diagram p10: hidden frame]
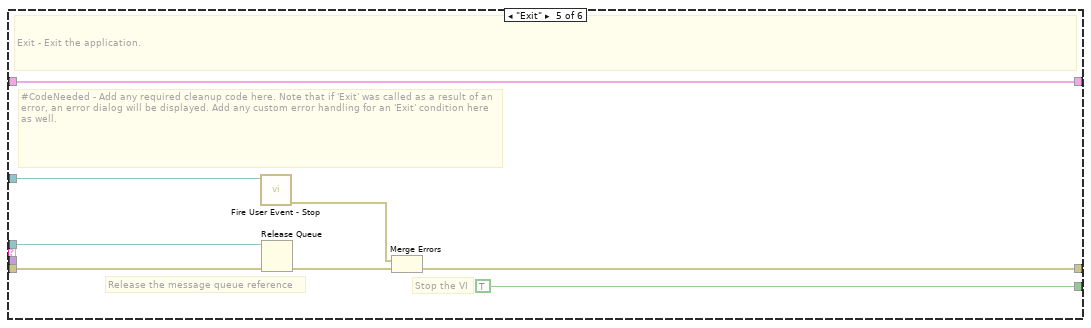
[diagram p11: hidden frame]
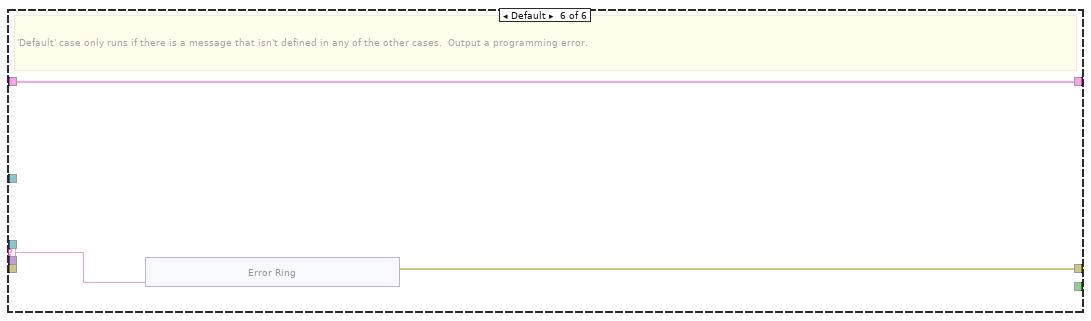
[diagram p12: hidden frame]
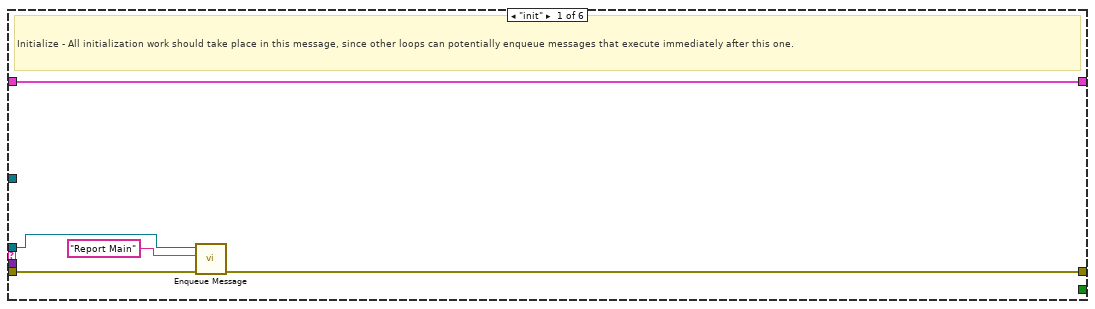
[diagram p14: hidden frame]
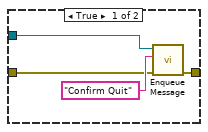
[diagram p15: hidden frame]
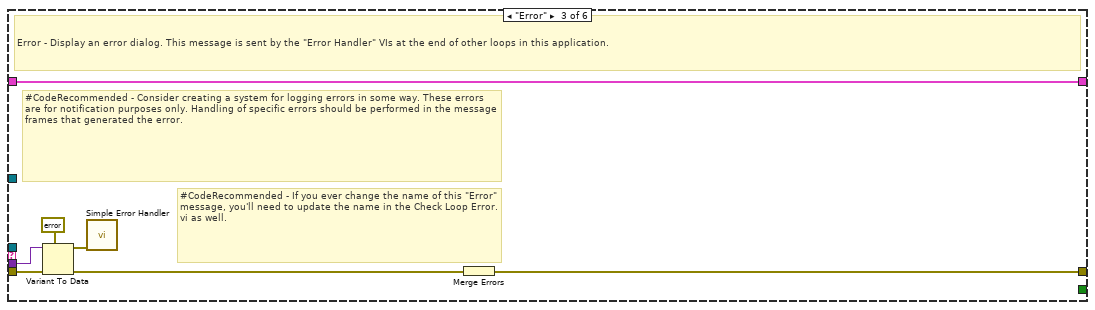
[diagram p16: hidden frame]
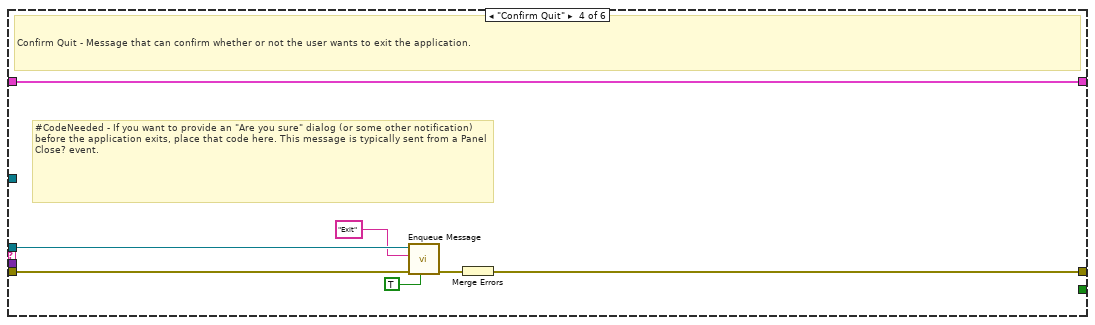
[diagram p17: hidden frame]
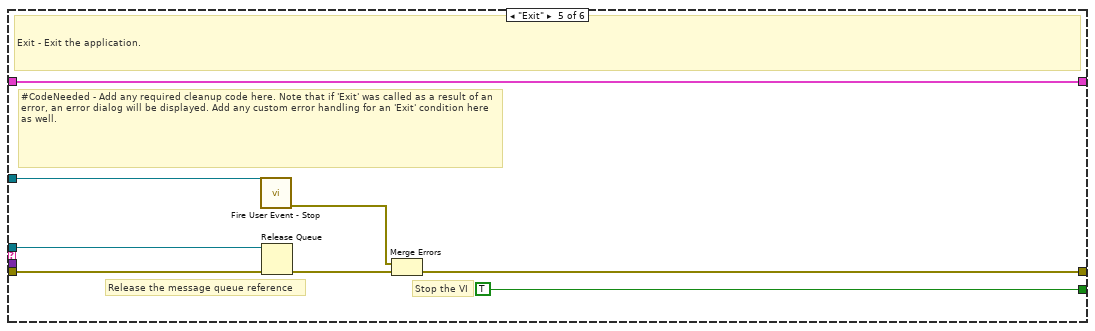
[diagram p18: hidden frame]
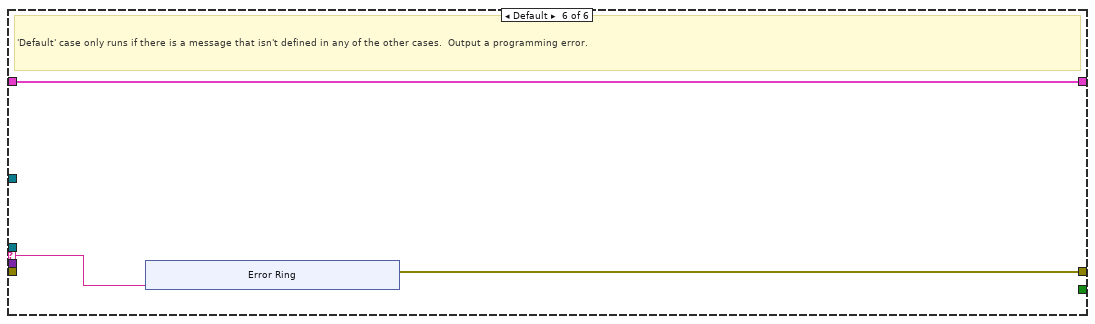
[diagram p19: hidden frame]
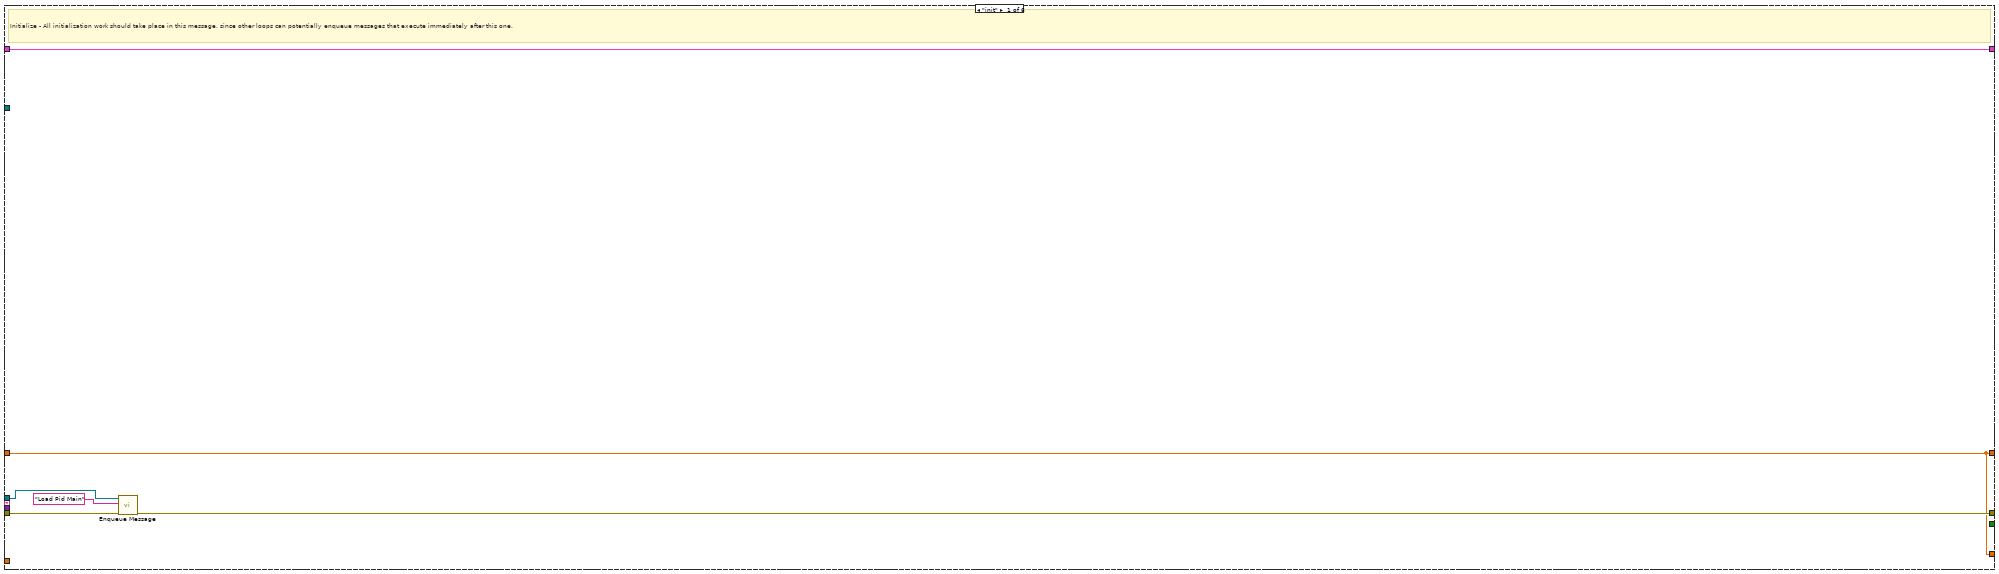
[diagram p20: hidden frame]
diagram:
  w1 = 0.0
  w8 = "" ("HEAVE OUT")
  w15 = -1  # max queue size
  (unwired) string[] ["PID DELAY (sec)", "Kp", "Ki", "Kd", "Deaadband", "pct_scale", "Init_step", "i_limit", "Max Step Limit", "i_limit", "Min_pos_limit", "Max_pos_limit", "Fine_tune_zone"]
  # "Start Test"
  n1 = flat-sequence {
    tunnel: [w68] -> w55
    tunnel: T12 {"Main Home Screen"={"GUI"=refnum, "Platform Settings"=refnum, "Configure"=refnum, "Home"=refnum, "EXIT"=refnum, "service 2"=refnum, "MainPage"=refnum, "Analysis"=refnum}, "Platform Settings"={"mm/s  Surge"=refnum, "Update Surge Speed"=refnum, "Drive Error"=refnum, "Disable Axis Jog Soft Limits"=refnum, "mm/s  Sway"=refnum, "Sway and Surge COM Status"=refnum, "Heave COM Status"=refnum, "Enable Platform"=refnum, "Surge Forward Main"=refnum, "Sway Right Main"=refnum, "Sway Left Main"=refnum, "Heave Down Main"=refnum, "Heave Up main"=refnum, "Update Sway Speed"=refnum, "Update Heave Speed"=refnum, "mm/s Heave"=refnum, "mm/sec"=refnum, "mm"=refnum, "Surge Backward Main"=refnum}, "Analysis Screen"={"Analysis Home"=refnum, "Surface Analysis"=refnum, "Imaging"=refnum, "Image Analysis"=refnum, "Post Analysis"=refnum}, "Config Screen"={"Select Load Head"=refnum, "Notes :"=refnum, "FILE"=refnum, "Sample ID :"=refnum, "Operator ID :"=refnum, "Operator Name :"=refnum, "Auto"=refnum}, "Motion Module"={"zNL"=refnum, "NL disp"=refnum, "Rotary Tab"=refnum, "Motion Direction:  3"=refnum, "E.Velocity 2"=refnum, "e.v/ssr 2"=refnum, "Enter Fixed E.Velocity 2"=refnum, "Enter Final SRR 2"=refnum, "Enter initial SRR 2"=refnum, "Enter Fixed SRR 2"=refnum, "Enter the Final E.Velocity (m/s) 2"=refnum, "Enter initial E.Velocity (m/s) 2"=refnum, "Final Speed (RPM) 3"=refnum, "Initial Speed (RPM) 2"=refnum, "Enter the Final Velocity (m/s) 3"=refnum, "Enter initial Velocity (m/s)  3"=refnum, "Ramp Up 2"=refnum, "TEST SELECTION"=refnum, "SPEED SELECTION : "=refnum, "Angular Oscillation Set"=refnum, "Traction"=refnum, "Step Speed"=refnum, "StepTable For Load-Speed"=refnum, "StepTable For Speed"=refnum, "Surge Forward MM"=refnum, "Surge Backward MM"=refnum, "M3 Image"=refnum, "String 39"=refnum, "Sway Left MM"=refnum, "Sway Right MM"=refnum, "Disable Axis Jog Soft Limits"=refnum, "mm"=refnum, "Heave Down MM"=refnum, "Heave Up MM"=refnum, "Wear Track Diameter (mm)"=refnum, "Set WTD"=refnum, "HomeScratch"=refnum, "HomeRot"=refnum, "PlaceModule"=refnum, "Enter the Angle (Deg)"=refnum, "Enter the Frequency (Hz)"=refnum, "Motion Mode:"=refnum, "LR Sway"=refnum, "Rot Hor"=refnum, "Scratch"=refnum, "LR Cam"=refnum, "MMBack"=refnum, "MMNext"=refnum, "Rot Ver"=refnum, "Rotary Module Selection"=refnum, "calculate rotary"=refnum, "SPEED SELECTION : rotary"=refnum, "Import 2"=refnum, "Save 2"=refnum, "File Path :  2"=refnum, "String 45"=refnum, "StepTable For Speed 3"=refnum, "Enter the Speed(mm/sec)"=refnum, "Enter the Speed(RPM)"=refnum}, "Environmental control"={"Humidity  Status  3"=refnum, "Low Temp  Status  2"=refnum, "TK4 status 2"=refnum, "Stage Temperature"=refnum, "Sample Temperature"=refnum, "Humidity (Amb)"=refnum, "Clear List"=refnum, "Add to list"=refnum, "Wear"=refnum, "Vibration"=refnum, "Humidity (Chamber)"=refnum, "Temperature (Chamber)"=refnum, "ECR "=refnum, "Temperature (Amb)"=refnum, "Microphone"=refnum, "Acoustic Emission 3"=refnum, "SNext"=refnum, "APBack"=refnum, "Enter the Temperature (°C):"=refnum, "Enter the Stage \nTemperature (°C):"=refnum, "Enter the Humidity (%Rh):"=refnum, "Low Temp"=refnum, "High Temp"=refnum, "Humidity"=refnum, "Sensors Picked"=refnum}, "About Screen"={"Password"=refnum, "Home Service"=refnum, "Advanced Setting"=refnum, "About Tab"=refnum, "ECR Port:"=refnum, "Ramp Port:"=refnum, "Installation/Replacement completed"=refnum, "Loahead"=refnum, "Heave and Surge COM Port:"=refnum, "Sway COM Port:"=refnum, "Temp Modbus:"=refnum, "Humidity Port:"=refnum, "Edit Gain Constants"=refnum, "Save Gain Constants"=refnum}, "Main Screen"={"Main Screen Tab"=refnum, "Angle and Frequency"=refnum, "Stroke (mm)"=refnum, "Angle (Deg)"=refnum, "Main Speed Tab"=refnum, "MTM MOTOR DISPLAY"=refnum, "Disc Speed (m/sec)"=refnum, "Ball Speed (m/sec)"=refnum, "Disc Speed (RPM)"=refnum, "Ball Speed (RPM)"=refnum, "SPEED TAB"=refnum, "Speed (m/sec)"=refnum, "Set Speed (m/sec)"=refnum, "Speed (RPM)"=refnum, "Set Speed"=refnum, "Time Tab"=refnum, "Time ( HH:MM:SS ) 2"=refnum, "Test Duration"=refnum, "Test Duration 4"=refnum, "TEST CYCLE"=refnum, "TOTAL CYCLES"=refnum, "Set Load (N)"=refnum, "Temp Tabs"=refnum, "Heater"=refnum, "TK4 status"=refnum, "ChamberTemp"=refnum, "SetTmp"=refnum, "Controller  Status"=refnum, "ChamberTemp 2"=refnum, "SetTmp 2"=refnum, "Controller  Status 2"=refnum, "ChamberTemp 3"=refnum, "SetTmp 3"=refnum, "Cooling"=refnum, "Load Communication"=refnum, "Ambient \nTemperature"=refnum, "HumCOMStatus"=refnum, "Ambient\n Humidity"=refnum, "Freq (Hz)"=refnum, "Load En"=refnum, "NLt"=refnum, "zNL 2"=refnum, "Humidity On"=refnum, "humidity disp"=refnum, "Set Humidity"=refnum, "NL disp 2"=refnum, "Humidity On 2"=refnum, "humidity disp 2"=refnum, "Set Humidity 2"=refnum, "NL disp 3"=refnum, "AppLoadSeq scratch"=refnum, "Stop Scratch"=refnum, "ClrLog"=refnum, "Trip Log"=refnum, "STOP"=refnum, "Start Test"=refnum, "Test status"=refnum, "AR Led"=refnum, "Data"=refnum, "Health"=refnum, "Sway COM Status"=refnum, "Heave COM Status"=refnum, "Grp Tab"=refnum, "Sub Graph"=refnum, "SD (mm)"=refnum, "Siliding distance Reset Graph"=refnum, "SDGp"=refnum, "Humidity Reset Graph"=refnum, "HumrGp"=refnum, "Acoustic Emission (mV)"=refnum, "Aqucostic Reset Graph"=refnum, "gACQUOS"=refnum, "ECR RESET"=refnum, "ECR"=refnum, "Temperature Reset"=refnum, "Acoustic Emission (mV) 2"=refnum, "Aqucostic Reset Graph 2"=refnum, "gACQUOS 2"=refnum, "ECR RESET 2"=refnum, "ECR 2"=refnum, "Temperature Reset 2"=refnum, "Temperature (deg c)"=refnum, "Speed Reset Graph"=refnum, "Speed Tab"=refnum, "MTM DISC  SPEED"=refnum, "MTM BALL SPEED"=refnum, "speed mm/sec"=refnum, "Hymidity"=refnum, "Humidity Disable trip"=refnum, "CoF Trip  2"=refnum, "Depth Trip"=refnum, "Weart Deapth"=refnum, "Depth Reset Graph"=refnum, "Weart"=refnum, "Depthz"=refnum, "Depth (µm)"=refnum, "WearGp"=refnum, "NL Trip 2"=refnum, "Load pid"=refnum, "Load Disable Trip"=refnum, "Load Reset Graph"=refnum, "NL Display 4"=refnum, "Main Chart 3"=refnum, "BACK"=refnum, "Depth Trip 2"=refnum, "COF TRIP "=refnum, "Friction Force (N)"=refnum, "FF Reset Graph"=refnum, "FF Disable Trip"=refnum, "FF TRIP"=refnum, "FF MAIN CHART"=refnum, "COF Disable Trip"=refnum, "COF Reset Graph"=refnum, "COF MAIN CHART"=refnum, "FF Tab"=refnum, "Start Test Temp"=refnum}, "Loading"={"Indentation"=refnum, "Reference Sample"=refnum, "Load Cell Communication Slide"=refnum, "com 3"=refnum, "com"=refnum, "DecaForce COM Status"=refnum, "Update"=refnum, "Clear 3"=refnum, "seq"=refnum, "Stribeck table"=refnum, "Stribeck Table  For loading"=refnum, "Loading Mode"=refnum, "Enter the Final Load (N)"=refnum, "Enter the CoF Trip"=refnum, "Enter the Friction Force Trip"=refnum, "Enter the Normal load Trip"=refnum, "Enter the Load  (N)"=refnum, "KiloForce"=refnum, "DecaForce "=refnum, "MicroForce"=refnum, "LHBack"=refnum, "LHNext"=refnum, "Enter the Loading Rate (N/min)"=refnum, "Message"=refnum, "Warning 2"=refnum, "SSP 0.75"=refnum, "SSP 0.5"=refnum, "SSP 0.3"=refnum, "Warning"=refnum, "gui GIF"=refnum, "Communication is established"=refnum, "AppLoad 4"=refnum, "Multipoint"=refnum, "Load Selection"=refnum}, "PID"={"Ramp MulFac"=refnum, "pulses LoadDiffRamp(2..10)"=refnum, "PulseControlRamp(diff<=3N)"=refnum, "SetLoadDeadband(%) Load(0-10N)"=refnum, "PID gains out delay (microForce)"=refnum, "Ramp"=refnum, "Gain 2"=refnum, "pulses LoadDiff(2..10)"=refnum, "pulses LoadDiff(11..50)"=refnum, "PulseControl(diff<=3N)"=refnum, "SetLoadDeadband(%)  2"=refnum, "Dummy Run"=refnum, "Vertical load (N)"=refnum, "AutoTune"=refnum, "Offset 3 "=refnum, "apply load"=refnum, "Offset  3"=refnum, "apply load 2"=refnum, "Enter ByPass Load"=refnum, "reinit 3"=refnum, "output range delay"=refnum, "PID gains out delay"=refnum, "Bypass Load"=refnum, "pulsesSent"=refnum, "pulses "=refnum, "actpid"=refnum, "gFF Rot"=refnum, "pulses LoadDiff(21..1000)"=refnum, "Delay"=refnum, "deadband"=refnum}, "Config Parameters"={"Tab Control 3"=refnum, "Tab Control 19"=refnum, "SAMPLES"=refnum, "Re-initilaize"=refnum, "Filter ON/OFF"=refnum, "TracHomeSurgeOffsetCounts 10MM"=refnum, "TracHomeSwayOffsetCounts 10MM"=refnum, "Acoustic Emission:"=refnum, "Apply Filter (FF)"=refnum, "Filter% 2"=refnum, "Apply Filter (Load)"=refnum, "Filter% "=refnum, "Sway distance (mm)"=refnum, "Surge distance (mm)"=refnum, "DataSavingLoopDelay(ms)"=refnum, "SAVE 2"=refnum, "Enter Distance"=refnum, "Sway Counts:"=refnum, "Distance (mm): 3"=refnum, "Surge Counts:"=refnum, "Distance (mm): 2"=refnum, "Distance (mm):"=refnum, "Heave Counts:"=refnum, "LRMHomeSurgeOffsetCounts"=refnum, "LRMHomeSwayOffsetCounts"=refnum, "TracHomeSurgeOffsetCounts 20MM"=refnum, "TracHomeSwayOffsetCounts 20MM"=refnum, "RotHomeSwayOffsetCounts"=refnum, "RotHomeSurgeOffsetCounts"=refnum, "Heave distance"=refnum, "Zmm"=refnum, "Heave Pulses/mm"=refnum, "Surge Pulses/mm"=refnum, "Sway Pulses/mm"=refnum, "Heave Pitch"=refnum, "Surge Pitch"=refnum, "Sway Pitch"=refnum, "Heave PPR"=refnum, "Surge PPR"=refnum, "Sway PPR"=refnum, "Tab Control 5"=refnum, "Tab Control 14"=refnum, "Tab Control 26"=refnum, "AE"=refnum, "Heave Loop Delay"=refnum, "Heave PID Speed"=refnum, "Surge Jog Speed"=refnum, "Heave Jog Speed"=refnum}, "Loading Com Port"={"ClearAll"=refnum, "Mz(Nm)"=refnum, "My(Nm)"=refnum, "Mx(Nm)"=refnum, "Save Dwell"=refnum, "Mx "=refnum, "My "=refnum, "Mz"=refnum, "Fx(N)"=refnum, "Fy(N)"=refnum, "Fz(N)"=refnum, "ZeroAll"=refnum, "Acq Delay (ms)"=refnum, "Burst Delay (ms)"=refnum, "model"=refnum, "SN"=refnum, "FFx(N)"=refnum, "Sensor IP"=refnum, "Port"=refnum, "FFy(N)"=refnum, "Load(N)"=refnum, "delete Handle"=refnum, "Create Handle"=refnum, "ft_data"=refnum, "ft_range"=refnum, "ft_data 2"=refnum, "stop 6"=refnum, "running_flag"=refnum, "ft_udp_handle"=refnum, "get-data-return"=refnum, "get-range-return"=refnum, "zero-return"=refnum, "filter-return"=refnum, "initial-return"=refnum, "deleteHandle-result"=refnum, "Load Cell Temp"=refnum}, "Heave AND Surge"={"SURGE POSE"=refnum, "error out Read"=refnum, "HEAVE POSE"=refnum, "State"=refnum, "Homed"=refnum, "Sequence ID"=refnum, "error out Write"=refnum, "faultCode"=refnum, "Ack ID"=refnum, "SPEED"=refnum, "Distance"=refnum, "Mode Command"=refnum, "Heave and Surge Read"=refnum, "Read Heave Temp"=refnum, "Spare 15"=refnum, "Spare 14"=refnum, "Spare 13"=refnum, "Spare 12"=refnum, "Spare 11"=refnum, "Spare 10"=refnum, "Spare 9"=refnum, "Spare 8"=refnum, "Spare 7"=refnum, "Spare 6"=refnum, "Spare 5"=refnum, "Spare 4"=refnum, "Spare 2"=refnum, "Spare 1"=refnum, "Node Id"=refnum, "Spare 3"=refnum, "SPARE 4"=refnum, "SPARE 3"=refnum, "SPARE 2"=refnum, "SPARE 1"=refnum, "fwMajor"=refnum, "fwMinor"=refnum, "Manual Write"=refnum, "Heave and Surge Write"=refnum}, "New PID LOGIC"={"Fine Tune Zone"=refnum, "PID SDelay"=refnum, "Max_pos_limit"=refnum, "Min_pos_limit"=refnum, "i_limit"=refnum, "pct_scale"=refnum, "Deadband"=refnum, "Kd"=refnum, "Ki"=refnum, "Kp"=refnum, "Current Position"=refnum, "Set Load"=refnum, "Current Load"=refnum, "Pulse delta"=refnum, "Init Step"=refnum, "Max Step Linit"=refnum}} ("Data Cluster") -> [w67]
    tunnel: w55 -> [w97]
    tunnel: [w77] -> w54
    tunnel: w54 -> [w104]
    tunnel: [w98] -> w53
    tunnel: w53 -> [w113]
    tunnel: [w112] -> w52
    tunnel: w52 -> [w149]
    tunnel: [w148] -> w50
    tunnel: w50 -> [w210]
    tunnel: [w209] -> w49
    tunnel: w49 -> [w237]
    tunnel: [w236] -> w48
    tunnel: w48 -> [w253]
    tunnel: [w252] -> w47
    tunnel: w47 -> [w358]
    tunnel: [w357] -> w22
    tunnel: w22 -> [w388]
    tunnel: [w387] -> w21
    tunnel: w21 -> [w438]
    tunnel: [w437] -> w20
    tunnel: w20 -> [w475]
    tunnel: [w474] -> w19
    tunnel: w19 -> [w515]
    tunnel: [w514] -> w17
    tunnel: [w532] -> w7
    tunnel: w17 -> [w533]
    frame #0 {
      n2 = control-ref of="GUI"() -> (w76:refnum<vi>)
      n3 = control-ref of="MainPage"() -> (w70:refnum<vi>)
      n4 = control-ref of="Platform Settings"() -> (w75:refnum<vi>)
      n5 = control-ref of="Configure"() -> (w74:refnum<vi>)
      n6 = control-ref of="Home"() -> (w73:refnum<vi>)
      n7 = control-ref of="EXIT"() -> (w72:refnum<vi>)
      n8 = control-ref of="service 2"() -> (w71:refnum<vi>)
      n9 = control-ref of="Analysis"() -> (w69:refnum<vi>)
      n10 = Bundle By Name(cluster=w67, "Main Home Screen.GUI"=w76, "Main Home Screen.Platform Settings"=w75, "Main Home Screen.Configure"=w74, "Main Home Screen.Home"=w73, "Main Home Screen.EXIT"=w72, "Main Home Screen.service 2"=w71, "Main Home Screen.MainPage"=w70, "Main Home Screen.Analysis"=w69) -> (w68:T12)
    }
    frame #1 {
      n11 = control-ref of="Sway Right Main"() -> (w87:refnum<vi>)
      n12 = control-ref of="Sway Left Main"() -> (w86:refnum<vi>)
      n13 = control-ref of="Heave Down Main"() -> (w85:refnum<vi>)
      n14 = control-ref of="Heave Up main"() -> (w84:refnum<vi>)
      n15 = control-ref of="Update Sway Speed"() -> (w83:refnum<vi>)
      n16 = control-ref of="Update Heave Speed"() -> (w82:refnum<vi>)
      n17 = control-ref of="Surge Backward Main"() -> (w78:refnum<vi>)
      n18 = control-ref of="Update Surge Speed"() -> (w95:refnum<vi>)
      n19 = control-ref of="Disable Axis Jog Soft Limits"() -> (w93:refnum<vi>)
      n20 = control-ref of="Sway and Surge COM Status"() -> (w91:refnum<vi>)
      n21 = control-ref of="Heave COM Status"() -> (w90:refnum<vi>)
      n22 = control-ref of="Enable Platform"() -> (w89:refnum<vi>)
      n23 = control-ref of="Surge Forward Main"() -> (w88:refnum<vi>)
      n24 = control-ref of="mm/s Heave"() -> (w81:refnum<vi>)
      n25 = control-ref of="mm/sec"() -> (w80:refnum<vi>)
      n26 = control-ref of="mm"() -> (w79:refnum<vi>)
      n27 = control-ref of="mm/s  Surge"() -> (w96:refnum<vi>)
      n28 = control-ref of="mm/s  Sway"() -> (w92:refnum<vi>)
      n29 = control-ref of="Drive Error"() -> (w94:refnum<vi>)
      n30 = Bundle By Name(cluster=w97, "Platform Settings.mm/s  Surge"=w96, "Platform Settings.Update Surge Speed"=w95, "Platform Settings.Drive Error"=w94, "Platform Settings.Disable Axis Jog Soft Limits"=w93, "Platform Settings.mm/s  Sway"=w92, "Platform Settings.Sway and Surge COM Status"=w91, "Platform Settings.Heave COM Status"=w90, "Platform Settings.Enable Platform"=w89, "Platform Settings.Surge Forward Main"=w88, "Platform Settings.Sway Right Main"=w87, "Platform Settings.Sway Left Main"=w86, "Platform Settings.Heave Down Main"=w85, "Platform Settings.Heave Up main"=w84, "Platform Settings.Update Sway Speed"=w83, "Platform Settings.Update Heave Speed"=w82, "Platform Settings.mm/s Heave"=w81, "Platform Settings.mm/sec"=w80, "Platform Settings.mm"=w79, "Platform Settings.Surge Backward Main"=w78) -> (w77:T12)
    }
    frame #2 {
      n31 = control-ref of="Analysis Home"() -> (w103:refnum<vi>)
      n32 = control-ref of="Surface Analysis"() -> (w102:refnum<vi>)
      n33 = control-ref of="Imaging"() -> (w101:refnum<vi>)
      n34 = control-ref of="Image Analysis"() -> (w100:refnum<vi>)
      n35 = control-ref of="Post Analysis"() -> (w99:refnum<vi>)
      n36 = Bundle By Name(cluster=w104, "Analysis Screen.Analysis Home"=w103, "Analysis Screen.Surface Analysis"=w102, "Analysis Screen.Imaging"=w101, "Analysis Screen.Image Analysis"=w100, "Analysis Screen.Post Analysis"=w99) -> (w98:T12)
    }
    frame #3 {
      n37 = control-ref of="Select Load Head"() -> (w111:refnum<vi>)
      n38 = control-ref of="Auto"() -> (w105:refnum<vi>)
      n39 = control-ref of="Notes :"() -> (w110:refnum<vi>)
      n40 = control-ref of="FILE"() -> (w109:refnum<vi>)
      n41 = control-ref of="Sample ID :"() -> (w108:refnum<vi>)
      n42 = control-ref of="Operator ID :"() -> (w107:refnum<vi>)
      n43 = control-ref of="Operator Name :"() -> (w106:refnum<vi>)
      n44 = Bundle By Name(cluster=w113, "Config Screen.Select Load Head"=w111, "Config Screen.Notes :"=w110, "Config Screen.FILE"=w109, "Config Screen.Sample ID :"=w108, "Config Screen.Operator ID :"=w107, "Config Screen.Operator Name :"=w106, "Config Screen.Auto"=w105) -> (w112:T12)
    }
    frame #4 {
      n45 = control-ref of="Warning"() -> (w141:refnum<vi>)
      n46 = control-ref of="gui GIF"() -> (w140:refnum<vi>)
      n47 = control-ref of="Load Selection"() -> (w114:refnum<vi>)
      n48 = control-ref of="Warning 2"() -> (w145:refnum<vi>)
      n49 = control-ref of="SSP 0.75"() -> (w144:refnum<vi>)
      n50 = control-ref of="SSP 0.5"() -> (w143:refnum<vi>)
      n51 = control-ref of="SSP 0.3"() -> (w142:refnum<vi>)
      n52 = control-ref of="Communication is established"() -> (w139:refnum<vi>)
      n53 = control-ref of="AppLoad 4"() -> (w138:refnum<vi>)
      n54 = control-ref of="Multipoint"() -> (w137:refnum<vi>)
      n55 = control-ref of="com 3"() -> (w133:refnum<vi>)
      n56 = control-ref of="com"() -> (w132:refnum<vi>)
      n57 = control-ref of="DecaForce COM Status"() -> (w131:refnum<vi>)
      n58 = control-ref of="Update"() -> (w130:refnum<vi>)
      n59 = control-ref of="Clear 3"() -> (w129:refnum<vi>)
      n60 = control-ref of="seq"() -> (w128:refnum<vi>)
      n61 = control-ref of="Stribeck table"() -> (w127:refnum<vi>)
      n62 = control-ref of="KiloForce"() -> (w119:refnum<vi>)
      n63 = control-ref of="DecaForce"() -> (w118:refnum<vi>)
      n64 = control-ref of="MicroForce"() -> (w117:refnum<vi>)
      n65 = control-ref of="LHBack"() -> (w116:refnum<vi>)
      n66 = control-ref of="LHNext"() -> (w115:refnum<vi>)
      n67 = control-ref of="Enter the Loading Rate (N/min)"() -> (w147:refnum<vi>)
      n68 = control-ref of="Enter the Final Load (N)"() -> (w124:refnum<vi>)
      n69 = control-ref of="Enter the CoF Trip"() -> (w123:refnum<vi>)
      n70 = control-ref of="Enter the Friction Force Trip"() -> (w122:refnum<vi>)
      n71 = control-ref of="Enter the Normal load Trip"() -> (w121:refnum<vi>)
      n72 = control-ref of="Enter the Load  (N)"() -> (w120:refnum<vi>)
      n73 = control-ref of="Message"() -> (w146:refnum<vi>)
      n74 = control-ref of="Indentation"() -> (w136:refnum<vi>)
      n75 = control-ref of="Stribeck Table  For loading"() -> (w126:refnum<vi>)
      n76 = control-ref of="Reference Sample"() -> (w135:refnum<vi>)
      n77 = control-ref of="Load Cell Communication Slide"() -> (w134:refnum<vi>)
      n78 = control-ref of="Loading Mode"() -> (w125:refnum<vi>)
      n79 = Bundle By Name(cluster=w149, "Loading.Enter the Loading Rate (N/min)"=w147, "Loading.Message"=w146, "Loading.Warning 2"=w145, "Loading.SSP 0.75"=w144, "Loading.SSP 0.5"=w143, "Loading.SSP 0.3"=w142, "Loading.Warning"=w141, "Loading.gui GIF"=w140, "Loading.Communication is established"=w139, "Loading.AppLoad 4"=w138, "Loading.Multipoint"=w137, "Loading.Indentation"=w136, "Loading.Reference Sample"=w135, "Loading.Load Cell Communication Slide"=w134, "Loading.com 3"=w133, "Loading.com"=w132, "Loading.DecaForce COM Status"=w131, "Loading.Update"=w130, "Loading.Clear 3"=w129, "Loading.seq"=w128, "Loading.Stribeck table"=w127, "Loading.Stribeck Table  For loading"=w126, "Loading.Loading Mode"=w125, "Loading.Enter the Final Load (N)"=w124, "Loading.Enter the CoF Trip"=w123, "Loading.Enter the Friction Force Trip"=w122, "Loading.Enter the Normal load Trip"=w121, "Loading.Enter the Load  (N)"=w120, "Loading.KiloForce"=w119, "Loading.DecaForce"=w118, "Loading.MicroForce"=w117, "Loading.LHBack"=w116, "Loading.LHNext"=w115, "Loading.Load Selection"=w114) -> (w148:T12)
    }
    frame #5 {
      n80 = control-ref of="TEST SELECTION"() -> (w191:refnum<vi>)
      n81 = control-ref of="SPEED SELECTION :"() -> (w190:refnum<vi>)
      n82 = control-ref of="SPEED SELECTION : rotary"() -> (w157:refnum<vi>)
      n83 = control-ref of="Rotary Tab"() -> (w206:refnum<vi>)
      n84 = control-ref of="e.v/ssr 2"() -> (w203:refnum<vi>)
      n85 = control-ref of="Step Speed"() -> (w187:refnum<vi>)
      n86 = control-ref of="M3 Image"() -> (w182:refnum<vi>)
      n87 = control-ref of="Rotary Module Selection"() -> (w159:refnum<vi>)
      n88 = control-ref of="zNL"() -> (w208:refnum<vi>)
      n89 = control-ref of="E.Velocity 2"() -> (w204:refnum<vi>)
      n90 = control-ref of="Ramp Up 2"() -> (w192:refnum<vi>)
      n91 = control-ref of="Angular Oscillation Set"() -> (w189:refnum<vi>)
      n92 = control-ref of="Traction"() -> (w188:refnum<vi>)
      n93 = control-ref of="Surge Forward MM"() -> (w184:refnum<vi>)
      n94 = control-ref of="Surge Backward MM"() -> (w183:refnum<vi>)
      n95 = control-ref of="Sway Left MM"() -> (w180:refnum<vi>)
      n96 = control-ref of="Sway Right MM"() -> (w179:refnum<vi>)
      n97 = control-ref of="Disable Axis Jog Soft Limits"() -> (w178:refnum<vi>)
      n98 = control-ref of="Heave Down MM"() -> (w176:refnum<vi>)
      n99 = control-ref of="Heave Up MM"() -> (w175:refnum<vi>)
      n100 = control-ref of="Set WTD"() -> (w173:refnum<vi>)
      n101 = control-ref of="HomeScratch"() -> (w172:refnum<vi>)
      n102 = control-ref of="HomeRot"() -> (w171:refnum<vi>)
      n103 = control-ref of="PlaceModule"() -> (w170:refnum<vi>)
      n104 = control-ref of="LR Sway"() -> (w166:refnum<vi>)
      n105 = control-ref of="Rot Hor"() -> (w165:refnum<vi>)
      n106 = control-ref of="Scratch"() -> (w164:refnum<vi>)
      n107 = control-ref of="LR Cam"() -> (w163:refnum<vi>)
      n108 = control-ref of="MMBack"() -> (w162:refnum<vi>)
      n109 = control-ref of="MMNext"() -> (w161:refnum<vi>)
      n110 = control-ref of="Rot Ver"() -> (w160:refnum<vi>)
      n111 = control-ref of="calculate rotary"() -> (w158:refnum<vi>)
      n112 = control-ref of="Import 2"() -> (w156:refnum<vi>)
      n113 = control-ref of="Save 2"() -> (w155:refnum<vi>)
      n114 = control-ref of="NL disp"() -> (w207:refnum<vi>)
      n115 = control-ref of="Enter Fixed E.Velocity 2"() -> (w202:refnum<vi>)
      n116 = control-ref of="Enter Final SRR 2"() -> (w201:refnum<vi>)
      n117 = control-ref of="Enter initial SRR 2"() -> (w200:refnum<vi>)
      n118 = control-ref of="Enter Fixed SRR 2"() -> (w199:refnum<vi>)
      n119 = control-ref of="Enter the Final E.Velocity (m/s) 2"() -> (w198:refnum<vi>)
      n120 = control-ref of="Enter initial E.Velocity (m/s) 2"() -> (w197:refnum<vi>)
      n121 = control-ref of="Final Speed (RPM) 3"() -> (w196:refnum<vi>)
      n122 = control-ref of="Initial Speed (RPM) 2"() -> (w195:refnum<vi>)
      n123 = control-ref of="Enter the Final Velocity (m/s) 3"() -> (w194:refnum<vi>)
      n124 = control-ref of="Enter initial Velocity (m/s)  3"() -> (w193:refnum<vi>)
      n125 = control-ref of="mm"() -> (w177:refnum<vi>)
      n126 = control-ref of="Wear Track Diameter (mm)"() -> (w174:refnum<vi>)
      n127 = control-ref of="Enter the Angle (Deg)"() -> (w169:refnum<vi>)
      n128 = control-ref of="Enter the Frequency (Hz)"() -> (w168:refnum<vi>)
      n129 = control-ref of="Enter the Speed(mm/sec)"() -> (w151:refnum<vi>)
      n130 = control-ref of="Enter the Speed(RPM)"() -> (w150:refnum<vi>)
      n131 = control-ref of="String 39"() -> (w181:refnum<vi>)
      n132 = control-ref of="String 45"() -> (w153:refnum<vi>)
      n133 = control-ref of="StepTable For Load-Speed"() -> (w186:refnum<vi>)
      n134 = control-ref of="StepTable For Speed"() -> (w185:refnum<vi>)
      n135 = control-ref of="Motion Direction:  3"() -> (w205:refnum<vi>)
      n136 = control-ref of="Motion Mode:"() -> (w167:refnum<vi>)
      n137 = control-ref of="StepTable For Speed 3"() -> (w152:refnum<vi>)
      n138 = control-ref of="File Path :  2"() -> (w154:refnum<vi>)
      n139 = Bundle By Name(cluster=w210, "Motion Module.zNL"=w208, "Motion Module.NL disp"=w207, "Motion Module.Rotary Tab"=w206, "Motion Module.Motion Direction:  3"=w205, "Motion Module.E.Velocity 2"=w204, "Motion Module.e.v/ssr 2"=w203, "Motion Module.Enter Fixed E.Velocity 2"=w202, "Motion Module.Enter Final SRR 2"=w201, "Motion Module.Enter initial SRR 2"=w200, "Motion Module.Enter Fixed SRR 2"=w199, "Motion Module.Enter the Final E.Velocity (m/s) 2"=w198, "Motion Module.Enter initial E.Velocity (m/s) 2"=w197, "Motion Module.Final Speed (RPM) 3"=w196, "Motion Module.Initial Speed (RPM) 2"=w195, "Motion Module.Enter the Final Velocity (m/s) 3"=w194, "Motion Module.Enter initial Velocity (m/s)  3"=w193, "Motion Module.Ramp Up 2"=w192, "Motion Module.TEST SELECTION"=w191, "Motion Module.SPEED SELECTION :"=w190, "Motion Module.Angular Oscillation Set"=w189, "Motion Module.Traction"=w188, "Motion Module.Step Speed"=w187, "Motion Module.StepTable For Load-Speed"=w186, "Motion Module.StepTable For Speed"=w185, "Motion Module.Surge Forward MM"=w184, "Motion Module.Surge Backward MM"=w183, "Motion Module.M3 Image"=w182, "Motion Module.String 39"=w181, "Motion Module.Sway Left MM"=w180, "Motion Module.Sway Right MM"=w179, "Motion Module.Disable Axis Jog Soft Limits"=w178, "Motion Module.mm"=w177, "Motion Module.Heave Down MM"=w176, "Motion Module.Heave Up MM"=w175, "Motion Module.Wear Track Diameter (mm)"=w174, "Motion Module.Set WTD"=w173, "Motion Module.HomeScratch"=w172, "Motion Module.HomeRot"=w171, "Motion Module.PlaceModule"=w170, "Motion Module.Enter the Angle (Deg)"=w169, "Motion Module.Enter the Frequency (Hz)"=w168, "Motion Module.Motion Mode:"=w167, "Motion Module.LR Sway"=w166, "Motion Module.Rot Hor"=w165, "Motion Module.Scratch"=w164, "Motion Module.LR Cam"=w163, "Motion Module.MMBack"=w162, "Motion Module.MMNext"=w161, "Motion Module.Rot Ver"=w160, "Motion Module.Rotary Module Selection"=w159, "Motion Module.calculate rotary"=w158, "Motion Module.SPEED SELECTION : rotary"=w157, "Motion Module.Import 2"=w156, "Motion Module.Save 2"=w155, "Motion Module.File Path :  2"=w154, "Motion Module.String 45"=w153, "Motion Module.StepTable For Speed 3"=w152, "Motion Module.Enter the Speed(mm/sec)"=w151, "Motion Module.Enter the Speed(RPM)"=w150) -> (w209:T12)
    }
    frame #6 {
      n140 = control-ref of="Add to list"() -> (w228:refnum<vi>)
      n141 = control-ref of="Wear"() -> (w227:refnum<vi>)
      n142 = control-ref of="Vibration"() -> (w226:refnum<vi>)
      n143 = control-ref of="Humidity (Chamber)"() -> (w225:refnum<vi>)
      n144 = control-ref of="Temperature (Chamber)"() -> (w224:refnum<vi>)
      n145 = control-ref of="ECR"() -> (w223:refnum<vi>)
      n146 = control-ref of="Temperature (Amb)"() -> (w222:refnum<vi>)
      n147 = control-ref of="Microphone"() -> (w221:refnum<vi>)
      n148 = control-ref of="Acoustic Emission 3"() -> (w220:refnum<vi>)
      n149 = control-ref of="SNext"() -> (w219:refnum<vi>)
      n150 = control-ref of="APBack"() -> (w218:refnum<vi>)
      n151 = control-ref of="Low Temp"() -> (w214:refnum<vi>)
      n152 = control-ref of="High Temp"() -> (w213:refnum<vi>)
      n153 = control-ref of="Humidity"() -> (w212:refnum<vi>)
      n154 = control-ref of="Humidity  Status  3"() -> (w235:refnum<vi>)
      n155 = control-ref of="Low Temp  Status  2"() -> (w234:refnum<vi>)
      n156 = control-ref of="TK4 status 2"() -> (w233:refnum<vi>)
      n157 = control-ref of="Humidity (Amb)"() -> (w230:refnum<vi>)
      n158 = control-ref of="Clear List"() -> (w229:refnum<vi>)
      n159 = control-ref of="Enter the Temperature (°C):"() -> (w217:refnum<vi>)
      n160 = control-ref of="Enter the Stage \nTemperature (°C):"() -> (w216:refnum<vi>)
      n161 = control-ref of="Enter the Humidity (%Rh):"() -> (w215:refnum<vi>)
      n162 = control-ref of="Sensors Picked"() -> (w211:refnum<vi>)
      n163 = control-ref of="Stage Temperature"() -> (w232:refnum<vi>)
      n164 = control-ref of="Sample Temperature"() -> (w231:refnum<vi>)
      n165 = Bundle By Name(cluster=w237, "Environmental control.Humidity  Status  3"=w235, "Environmental control.Low Temp  Status  2"=w234, "Environmental control.TK4 status 2"=w233, "Environmental control.Stage Temperature"=w232, "Environmental control.Sample Temperature"=w231, "Environmental control.Humidity (Amb)"=w230, "Environmental control.Clear List"=w229, "Environmental control.Add to list"=w228, "Environmental control.Wear"=w227, "Environmental control.Vibration"=w226, "Environmental control.Humidity (Chamber)"=w225, "Environmental control.Temperature (Chamber)"=w224, "Environmental control.ECR"=w223, "Environmental control.Temperature (Amb)"=w222, "Environmental control.Microphone"=w221, "Environmental control.Acoustic Emission 3"=w220, "Environmental control.SNext"=w219, "Environmental control.APBack"=w218, "Environmental control.Enter the Temperature (°C):"=w217, "Environmental control.Enter the Stage \nTemperature (°C):"=w216, "Environmental control.Enter the Humidity (%Rh):"=w215, "Environmental control.Low Temp"=w214, "Environmental control.High Temp"=w213, "Environmental control.Humidity"=w212, "Environmental control.Sensors Picked"=w211) -> (w236:T12)
    }
    frame #7 {
      n166 = control-ref of="ECR Port:"() -> (w247:refnum<vi>)
      n167 = control-ref of="Ramp Port:"() -> (w246:refnum<vi>)
      n168 = control-ref of="Heave and Surge COM Port:"() -> (w243:refnum<vi>)
      n169 = control-ref of="Sway COM Port:"() -> (w242:refnum<vi>)
      n170 = control-ref of="Temp Modbus:"() -> (w241:refnum<vi>)
      n171 = control-ref of="Humidity Port:"() -> (w240:refnum<vi>)
      n172 = control-ref of="About Tab"() -> (w248:refnum<vi>)
      n173 = control-ref of="Home Service"() -> (w250:refnum<vi>)
      n174 = control-ref of="Advanced Setting"() -> (w249:refnum<vi>)
      n175 = control-ref of="Installation/Replacement completed"() -> (w245:refnum<vi>)
      n176 = control-ref of="Loahead"() -> (w244:refnum<vi>)
      n177 = control-ref of="Edit Gain Constants"() -> (w239:refnum<vi>)
      n178 = control-ref of="Save Gain Constants"() -> (w238:refnum<vi>)
      n179 = control-ref of="Password"() -> (w251:refnum<vi>)
      n180 = Bundle By Name(cluster=w253, "About Screen.Password"=w251, "About Screen.Home Service"=w250, "About Screen.Advanced Setting"=w249, "About Screen.About Tab"=w248, "About Screen.ECR Port:"=w247, "About Screen.Ramp Port:"=w246, "About Screen.Installation/Replacement completed"=w245, "About Screen.Loahead"=w244, "About Screen.Heave and Surge COM Port:"=w243, "About Screen.Sway COM Port:"=w242, "About Screen.Temp Modbus:"=w241, "About Screen.Humidity Port:"=w240, "About Screen.Edit Gain Constants"=w239, "About Screen.Save Gain Constants"=w238) -> (w252:T12)
    }
    frame #8 {
      n181 = control-ref of="SDGp"() -> (w297:refnum<vi>)
      n182 = control-ref of="HumrGp"() -> (w295:refnum<vi>)
      n183 = control-ref of="gACQUOS"() -> (w292:refnum<vi>)
      n184 = control-ref of="ECR"() -> (w290:refnum<vi>)
      n185 = control-ref of="Temperature (deg c)"() -> (w288:refnum<vi>)
      n186 = control-ref of="MTM DISC  SPEED"() -> (w285:refnum<vi>)
      n187 = control-ref of="MTM BALL SPEED"() -> (w284:refnum<vi>)
      n188 = control-ref of="speed mm/sec"() -> (w283:refnum<vi>)
      n189 = control-ref of="WearGp"() -> (w273:refnum<vi>)
      n190 = control-ref of="Main Chart 3"() -> (w267:refnum<vi>)
      n191 = control-ref of="FF MAIN CHART"() -> (w259:refnum<vi>)
      n192 = control-ref of="COF MAIN CHART"() -> (w256:refnum<vi>)
      n193 = control-ref of="Main Screen Tab"() -> (w356:refnum<vi>)
      n194 = control-ref of="Angle and Frequency"() -> (w355:refnum<vi>)
      n195 = control-ref of="Main Speed Tab"() -> (w352:refnum<vi>)
      n196 = control-ref of="MTM MOTOR DISPLAY"() -> (w351:refnum<vi>)
      n197 = control-ref of="SPEED TAB"() -> (w346:refnum<vi>)
      n198 = control-ref of="Time Tab"() -> (w341:refnum<vi>)
      n199 = control-ref of="Temp Tabs"() -> (w334:refnum<vi>)
      n200 = control-ref of="Grp Tab"() -> (w301:refnum<vi>)
      n201 = control-ref of="Sub Graph"() -> (w300:refnum<vi>)
      n202 = control-ref of="Speed Tab"() -> (w286:refnum<vi>)
      n203 = control-ref of="FF Tab"() -> (w255:refnum<vi>)
      n204 = control-ref of="Heater"() -> (w333:refnum<vi>)
      n205 = control-ref of="TK4 status"() -> (w332:refnum<vi>)
      n206 = control-ref of="Controller  Status"() -> (w329:refnum<vi>)
      n207 = control-ref of="Cooling"() -> (w326:refnum<vi>)
      n208 = control-ref of="Load Communication"() -> (w325:refnum<vi>)
      n209 = control-ref of="HumCOMStatus"() -> (w323:refnum<vi>)
      n210 = control-ref of="Load En"() -> (w320:refnum<vi>)
      n211 = control-ref of="NLt"() -> (w319:refnum<vi>)
      n212 = control-ref of="zNL 2"() -> (w318:refnum<vi>)
      n213 = control-ref of="Humidity On"() -> (w317:refnum<vi>)
      n214 = control-ref of="AppLoadSeq scratch"() -> (w313:refnum<vi>)
      n215 = control-ref of="Stop Scratch"() -> (w312:refnum<vi>)
      n216 = control-ref of="ClrLog"() -> (w311:refnum<vi>)
      n217 = control-ref of="STOP"() -> (w309:refnum<vi>)
      n218 = control-ref of="Start Test"() -> (w308:refnum<vi>)
      n219 = control-ref of="Test status"() -> (w307:refnum<vi>)
      n220 = control-ref of="AR Led"() -> (w306:refnum<vi>)
      n221 = control-ref of="Data"() -> (w305:refnum<vi>)
      n222 = control-ref of="Health"() -> (w304:refnum<vi>)
      n223 = control-ref of="Sway COM Status"() -> (w303:refnum<vi>)
      n224 = control-ref of="Heave COM Status"() -> (w302:refnum<vi>)
      n225 = control-ref of="Siliding distance Reset Graph"() -> (w298:refnum<vi>)
      n226 = control-ref of="Humidity Reset Graph"() -> (w296:refnum<vi>)
      n227 = control-ref of="Aqucostic Reset Graph"() -> (w293:refnum<vi>)
      n228 = control-ref of="ECR RESET"() -> (w291:refnum<vi>)
      n229 = control-ref of="Temperature Reset"() -> (w289:refnum<vi>)
      n230 = control-ref of="Speed Reset Graph"() -> (w287:refnum<vi>)
      n231 = control-ref of="Hymidity"() -> (w282:refnum<vi>)
      n232 = control-ref of="Humidity Disable trip"() -> (w281:refnum<vi>)
      n233 = control-ref of="Weart Deapth"() -> (w278:refnum<vi>)
      n234 = control-ref of="Depth Reset Graph"() -> (w277:refnum<vi>)
      n235 = control-ref of="Weart"() -> (w276:refnum<vi>)
      n236 = control-ref of="Depthz"() -> (w275:refnum<vi>)
      n237 = control-ref of="Load pid"() -> (w271:refnum<vi>)
      n238 = control-ref of="Load Disable Trip"() -> (w270:refnum<vi>)
      n239 = control-ref of="Load Reset Graph"() -> (w269:refnum<vi>)
      n240 = control-ref of="BACK"() -> (w266:refnum<vi>)
      n241 = control-ref of="FF Reset Graph"() -> (w262:refnum<vi>)
      n242 = control-ref of="FF Disable Trip"() -> (w261:refnum<vi>)
      n243 = control-ref of="COF Disable Trip"() -> (w258:refnum<vi>)
      n244 = control-ref of="COF Reset Graph"() -> (w257:refnum<vi>)
      n245 = control-ref of="Start Test Temp"() -> (w254:refnum<vi>)
      n246 = control-ref of="Depth Trip"() -> (w265:refnum<vi>)
      n247 = control-ref of="Stroke (mm)"() -> (w354:refnum<vi>)
      n248 = control-ref of="Angle (Deg)"() -> (w353:refnum<vi>)
      n249 = control-ref of="Disc Speed (m/sec)"() -> (w350:refnum<vi>)
      n250 = control-ref of="Ball Speed (m/sec)"() -> (w349:refnum<vi>)
      n251 = control-ref of="Disc Speed (RPM)"() -> (w348:refnum<vi>)
      n252 = control-ref of="Ball Speed (RPM)"() -> (w347:refnum<vi>)
      n253 = control-ref of="Speed (m/sec)"() -> (w345:refnum<vi>)
      n254 = control-ref of="Set Speed (m/sec)"() -> (w344:refnum<vi>)
      n255 = control-ref of="Speed (RPM)"() -> (w343:refnum<vi>)
      n256 = control-ref of="Set Speed"() -> (w342:refnum<vi>)
      n257 = control-ref of="Time ( HH:MM:SS ) 2"() -> (w340:refnum<vi>)
      n258 = control-ref of="Test Duration"() -> (w339:refnum<vi>)
      n259 = control-ref of="Test Duration 4"() -> (w338:refnum<vi>)
      n260 = control-ref of="TEST CYCLE"() -> (w337:refnum<vi>)
      n261 = control-ref of="TOTAL CYCLES"() -> (w336:refnum<vi>)
      n262 = control-ref of="Set Load (N)"() -> (w335:refnum<vi>)
      n263 = control-ref of="ChamberTemp"() -> (w331:refnum<vi>)
      n264 = control-ref of="SetTmp"() -> (w330:refnum<vi>)
      n265 = control-ref of="ChamberTemp"() -> (w328:refnum<vi>)
      n266 = control-ref of="SetTmp"() -> (w327:refnum<vi>)
      n267 = control-ref of="Ambient \nTemperature"() -> (w324:refnum<vi>)
      n268 = control-ref of="Ambient\n Humidity"() -> (w322:refnum<vi>)
      n269 = control-ref of="Freq (Hz)"() -> (w321:refnum<vi>)
      n270 = control-ref of="humidity disp"() -> (w316:refnum<vi>)
      n271 = control-ref of="Set Humidity"() -> (w315:refnum<vi>)
      n272 = control-ref of="NL disp 2"() -> (w314:refnum<vi>)
      n273 = control-ref of="SD (mm)"() -> (w299:refnum<vi>)
      n274 = control-ref of="Acoustic Emission (mV)"() -> (w294:refnum<vi>)
      n275 = control-ref of="CoF Trip  2"() -> (w280:refnum<vi>)
      n276 = control-ref of="Depth Trip"() -> (w279:refnum<vi>)
      n277 = control-ref of="Depth (µm)"() -> (w274:refnum<vi>)
      n278 = control-ref of="NL Trip 2"() -> (w272:refnum<vi>)
      n279 = control-ref of="NL Display 4"() -> (w268:refnum<vi>)
      n280 = control-ref of="COF TRIP"() -> (w264:refnum<vi>)
      n281 = control-ref of="Friction Force (N)"() -> (w263:refnum<vi>)
      n282 = control-ref of="FF TRIP"() -> (w260:refnum<vi>)
      n283 = control-ref of="Trip Log"() -> (w310:refnum<vi>)
      n284 = Bundle By Name(cluster=w358, "Main Screen.Main Screen Tab"=w356, "Main Screen.Angle and Frequency"=w355, "Main Screen.Stroke (mm)"=w354, "Main Screen.Angle (Deg)"=w353, "Main Screen.Main Speed Tab"=w352, "Main Screen.MTM MOTOR DISPLAY"=w351, "Main Screen.Disc Speed (m/sec)"=w350, "Main Screen.Ball Speed (m/sec)"=w349, "Main Screen.Disc Speed (RPM)"=w348, "Main Screen.Ball Speed (RPM)"=w347, "Main Screen.SPEED TAB"=w346, "Main Screen.Speed (m/sec)"=w345, "Main Screen.Set Speed (m/sec)"=w344, "Main Screen.Speed (RPM)"=w343, "Main Screen.Set Speed"=w342, "Main Screen.Time Tab"=w341, "Main Screen.Time ( HH:MM:SS ) 2"=w340, "Main Screen.Test Duration"=w339, "Main Screen.Test Duration 4"=w338, "Main Screen.TEST CYCLE"=w337, "Main Screen.TOTAL CYCLES"=w336, "Main Screen.Set Load (N)"=w335, "Main Screen.Temp Tabs"=w334, "Main Screen.Heater"=w333, "Main Screen.TK4 status"=w332, "Main Screen.ChamberTemp"=w331, "Main Screen.SetTmp"=w330, "Main Screen.Controller  Status"=w329, "Main Screen.ChamberTemp 2"=w328, "Main Screen.SetTmp 2"=w327, "Main Screen.Cooling"=w326, "Main Screen.Load Communication"=w325, "Main Screen.Ambient \nTemperature"=w324, "Main Screen.HumCOMStatus"=w323, "Main Screen.Ambient\n Humidity"=w322, "Main Screen.Freq (Hz)"=w321, "Main Screen.Load En"=w320, "Main Screen.NLt"=w319, "Main Screen.zNL 2"=w318, "Main Screen.Humidity On"=w317, "Main Screen.humidity disp"=w316, "Main Screen.Set Humidity"=w315, "Main Screen.NL disp 2"=w314, "Main Screen.AppLoadSeq scratch"=w313, "Main Screen.Stop Scratch"=w312, "Main Screen.ClrLog"=w311, "Main Screen.Trip Log"=w310, "Main Screen.STOP"=w309, "Main Screen.Start Test"=w308, "Main Screen.Test status"=w307, "Main Screen.AR Led"=w306, "Main Screen.Data"=w305, "Main Screen.Health"=w304, "Main Screen.Sway COM Status"=w303, "Main Screen.Heave COM Status"=w302, "Main Screen.Grp Tab"=w301, "Main Screen.Sub Graph"=w300, "Main Screen.SD (mm)"=w299, "Main Screen.Siliding distance Reset Graph"=w298, "Main Screen.SDGp"=w297, "Main Screen.Humidity Reset Graph"=w296, "Main Screen.HumrGp"=w295, "Main Screen.Acoustic Emission (mV)"=w294, "Main Screen.Aqucostic Reset Graph"=w293, "Main Screen.gACQUOS"=w292, "Main Screen.ECR RESET"=w291, "Main Screen.ECR"=w290, "Main Screen.Temperature Reset"=w289, "Main Screen.Temperature (deg c)"=w288, "Main Screen.Speed Reset Graph"=w287, "Main Screen.Speed Tab"=w286, "Main Screen.MTM DISC  SPEED"=w285, "Main Screen.MTM BALL SPEED"=w284, "Main Screen.speed mm/sec"=w283, "Main Screen.Hymidity"=w282, "Main Screen.Humidity Disable trip"=w281, "Main Screen.CoF Trip  2"=w280, "Main Screen.Depth Trip"=w279, "Main Screen.Weart Deapth"=w278, "Main Screen.Depth Reset Graph"=w277, "Main Screen.Weart"=w276, "Main Screen.Depthz"=w275, "Main Screen.Depth (µm)"=w274, "Main Screen.WearGp"=w273, "Main Screen.NL Trip 2"=w272, "Main Screen.Load pid"=w271, "Main Screen.Load Disable Trip"=w270, "Main Screen.Load Reset Graph"=w269, "Main Screen.NL Display 4"=w268, "Main Screen.Main Chart 3"=w267, "Main Screen.BACK"=w266, "Main Screen.Depth Trip 2"=w265, "Main Screen.COF TRIP"=w264, "Main Screen.Friction Force (N)"=w263, "Main Screen.FF Reset Graph"=w262, "Main Screen.FF Disable Trip"=w261, "Main Screen.FF TRIP"=w260, "Main Screen.FF MAIN CHART"=w259, "Main Screen.COF Disable Trip"=w258, "Main Screen.COF Reset Graph"=w257, "Main Screen.COF MAIN CHART"=w256, "Main Screen.FF Tab"=w255, "Main Screen.Start Test Temp"=w254) -> (w357:T12)
    }
    frame #9 {
      n285 = control-ref of="gFF Rot 7"() -> (w362:refnum<vi>)
      n286 = control-ref of="Ramp"() -> (w381:refnum<vi>)
      n287 = control-ref of="Dummy Run"() -> (w375:refnum<vi>)
      n288 = control-ref of="AutoTune"() -> (w373:refnum<vi>)
      n289 = control-ref of="apply load"() -> (w371:refnum<vi>)
      n290 = control-ref of="reinit 3"() -> (w369:refnum<vi>)
      n291 = control-ref of="Bypass Load"() -> (w366:refnum<vi>)
      n292 = control-ref of="PID gains out delay (microForce)"() -> (w382:refnum<vi>)
      n293 = control-ref of="output range delay"() -> (w368:refnum<vi>)
      n294 = control-ref of="PID gains out delay"() -> (w367:refnum<vi>)
      n295 = control-ref of="Ramp MulFac"() -> (w386:refnum<vi>)
      n296 = control-ref of="pulses LoadDiffRamp(2..10)"() -> (w385:refnum<vi>)
      n297 = control-ref of="PulseControlRamp(diff<=3N)"() -> (w384:refnum<vi>)
      n298 = control-ref of="SetLoadDeadband(%) Load(0-10N)"() -> (w383:refnum<vi>)
      n299 = control-ref of="Gain 2"() -> (w380:refnum<vi>)
      n300 = control-ref of="pulses LoadDiff(2..10)"() -> (w379:refnum<vi>)
      n301 = control-ref of="pulses LoadDiff(11..50)"() -> (w378:refnum<vi>)
      n302 = control-ref of="PulseControl(diff<=3N)"() -> (w377:refnum<vi>)
      n303 = control-ref of="SetLoadDeadband(%)  2"() -> (w376:refnum<vi>)
      n304 = control-ref of="Vertical load (N)"() -> (w374:refnum<vi>)
      n305 = control-ref of="Offset  3"() -> (w372:refnum<vi>)
      n306 = control-ref of="Enter ByPass Load"() -> (w370:refnum<vi>)
      n307 = control-ref of="pulsesSent"() -> (w365:refnum<vi>)
      n308 = control-ref of="pulses"() -> (w364:refnum<vi>)
      n309 = control-ref of="actpid"() -> (w363:refnum<vi>)
      n310 = control-ref of="pulses LoadDiff(21..1000)"() -> (w361:refnum<vi>)
      n311 = control-ref of="Delay"() -> (w360:refnum<vi>)
      n312 = control-ref of="deadband"() -> (w359:refnum<vi>)
      n313 = Bundle By Name(cluster=w388, "PID.Ramp MulFac"=w386, "PID.pulses LoadDiffRamp(2..10)"=w385, "PID.PulseControlRamp(diff<=3N)"=w384, "PID.SetLoadDeadband(%) Load(0-10N)"=w383, "PID.PID gains out delay (microForce)"=w382, "PID.Ramp"=w381, "PID.Gain 2"=w380, "PID.pulses LoadDiff(2..10)"=w379, "PID.pulses LoadDiff(11..50)"=w378, "PID.PulseControl(diff<=3N)"=w377, "PID.SetLoadDeadband(%)  2"=w376, "PID.Dummy Run"=w375, "PID.Vertical load (N)"=w374, "PID.AutoTune"=w373, "PID.Offset 3"=w372, "PID.apply load"=w371, "PID.Enter ByPass Load"=w370, "PID.reinit 3"=w369, "PID.output range delay"=w368, "PID.PID gains out delay"=w367, "PID.Bypass Load"=w366, "PID.pulsesSent"=w365, "PID.pulses"=w364, "PID.actpid"=w363, "PID.gFF Rot"=w362, "PID.pulses LoadDiff(21..1000)"=w361, "PID.Delay"=w360, "PID.deadband"=w359) -> (w387:T12)
    }
    frame #10 {
      n314 = control-ref of="Tab Control 3"() -> (w436:refnum<vi>)
      n315 = control-ref of="Tab Control 19"() -> (w435:refnum<vi>)
      n316 = control-ref of="Tab Control 5"() -> (w396:refnum<vi>)
      n317 = control-ref of="Tab Control 14"() -> (w395:refnum<vi>)
      n318 = control-ref of="Tab Control 26"() -> (w394:refnum<vi>)
      n319 = control-ref of="Re-initilaize"() -> (w433:refnum<vi>)
      n320 = control-ref of="Filter ON/OFF"() -> (w432:refnum<vi>)
      n321 = control-ref of="Apply Filter (FF)"() -> (w428:refnum<vi>)
      n322 = control-ref of="Apply Filter (Load)"() -> (w426:refnum<vi>)
      n323 = control-ref of="SAVE  2"() -> (w421:refnum<vi>)
      n324 = control-ref of="Enter Distance"() -> (w420:refnum<vi>)
      n325 = control-ref of="AE"() -> (w393:refnum<vi>)
      n326 = control-ref of="Heave Loop Delay"() -> (w392:refnum<vi>)
      n327 = control-ref of="Heave PID Speed"() -> (w391:refnum<vi>)
      n328 = control-ref of="Surge Jog Speed"() -> (w390:refnum<vi>)
      n329 = control-ref of="Heave Jog Speed"() -> (w389:refnum<vi>)
      n330 = control-ref of="SAMPLES"() -> (w434:refnum<vi>)
      n331 = control-ref of="TracHomeSurgeOffsetCounts 10MM"() -> (w431:refnum<vi>)
      n332 = control-ref of="TracHomeSwayOffsetCounts 10MM"() -> (w430:refnum<vi>)
      n333 = control-ref of="Acoustic Emission:"() -> (w429:refnum<vi>)
      n334 = control-ref of="Filter% 2"() -> (w427:refnum<vi>)
      n335 = control-ref of="Filter%"() -> (w425:refnum<vi>)
      n336 = control-ref of="Sway distance (mm)"() -> (w424:refnum<vi>)
      n337 = control-ref of="Surge distance (mm)"() -> (w423:refnum<vi>)
      n338 = control-ref of="DataSavingLoopDelay(ms)"() -> (w422:refnum<vi>)
      n339 = control-ref of="Sway Counts:"() -> (w419:refnum<vi>)
      n340 = control-ref of="Distance (mm): 3"() -> (w418:refnum<vi>)
      n341 = control-ref of="Surge Counts:"() -> (w417:refnum<vi>)
      n342 = control-ref of="Distance (mm): 2"() -> (w416:refnum<vi>)
      n343 = control-ref of="Distance (mm):"() -> (w415:refnum<vi>)
      n344 = control-ref of="Heave Counts:"() -> (w414:refnum<vi>)
      n345 = control-ref of="LRMHomeSurgeOffsetCounts"() -> (w413:refnum<vi>)
      n346 = control-ref of="LRMHomeSwayOffsetCounts"() -> (w412:refnum<vi>)
      n347 = control-ref of="TracHomeSurgeOffsetCounts 20MM"() -> (w411:refnum<vi>)
      n348 = control-ref of="TracHomeSwayOffsetCounts 20MM"() -> (w410:refnum<vi>)
      n349 = control-ref of="RotHomeSwayOffsetCounts"() -> (w409:refnum<vi>)
      n350 = control-ref of="RotHomeSurgeOffsetCounts"() -> (w408:refnum<vi>)
      n351 = control-ref of="Heave distance"() -> (w407:refnum<vi>)
      n352 = control-ref of="Zmm"() -> (w406:refnum<vi>)
      n353 = control-ref of="Heave Pulses/mm"() -> (w405:refnum<vi>)
      n354 = control-ref of="Surge Pulses/mm"() -> (w404:refnum<vi>)
      n355 = control-ref of="Sway Pulses/mm"() -> (w403:refnum<vi>)
      n356 = control-ref of="Heave Pitch"() -> (w402:refnum<vi>)
      n357 = control-ref of="Surge Pitch"() -> (w401:refnum<vi>)
      n358 = control-ref of="Sway Pitch"() -> (w400:refnum<vi>)
      n359 = control-ref of="Heave PPR"() -> (w399:refnum<vi>)
      n360 = control-ref of="Surge PPR"() -> (w398:refnum<vi>)
      n361 = control-ref of="Sway PPR"() -> (w397:refnum<vi>)
      n362 = Bundle By Name(cluster=w438, "Config Parameters.Tab Control 3"=w436, "Config Parameters.Tab Control 19"=w435, "Config Parameters.SAMPLES"=w434, "Config Parameters.Re-initilaize"=w433, "Config Parameters.Filter ON/OFF"=w432, "Config Parameters.TracHomeSurgeOffsetCounts 10MM"=w431, "Config Parameters.TracHomeSwayOffsetCounts 10MM"=w430, "Config Parameters.Acoustic Emission:"=w429, "Config Parameters.Apply Filter (FF)"=w428, "Config Parameters.Filter% 2"=w427, "Config Parameters.Apply Filter (Load)"=w426, "Config Parameters.Filter%"=w425, "Config Parameters.Sway distance (mm)"=w424, "Config Parameters.Surge distance (mm)"=w423, "Config Parameters.DataSavingLoopDelay(ms)"=w422, "Config Parameters.SAVE 2"=w421, "Config Parameters.Enter Distance"=w420, "Config Parameters.Sway Counts:"=w419, "Config Parameters.Distance (mm): 3"=w418, "Config Parameters.Surge Counts:"=w417, "Config Parameters.Distance (mm): 2"=w416, "Config Parameters.Distance (mm):"=w415, "Config Parameters.Heave Counts:"=w414, "Config Parameters.LRMHomeSurgeOffsetCounts"=w413, "Config Parameters.LRMHomeSwayOffsetCounts"=w412, "Config Parameters.TracHomeSurgeOffsetCounts 20MM"=w411, "Config Parameters.TracHomeSwayOffsetCounts 20MM"=w410, "Config Parameters.RotHomeSwayOffsetCounts"=w409, "Config Parameters.RotHomeSurgeOffsetCounts"=w408, "Config Parameters.Heave distance"=w407, "Config Parameters.Zmm"=w406, "Config Parameters.Heave Pulses/mm"=w405, "Config Parameters.Surge Pulses/mm"=w404, "Config Parameters.Sway Pulses/mm"=w403, "Config Parameters.Heave Pitch"=w402, "Config Parameters.Surge Pitch"=w401, "Config Parameters.Sway Pitch"=w400, "Config Parameters.Heave PPR"=w399, "Config Parameters.Surge PPR"=w398, "Config Parameters.Sway PPR"=w397, "Config Parameters.Tab Control 5"=w396, "Config Parameters.Tab Control 14"=w395, "Config Parameters.Tab Control 26"=w394, "Config Parameters.AE"=w393, "Config Parameters.Heave Loop Delay"=w392, "Config Parameters.Heave PID Speed"=w391, "Config Parameters.Surge Jog Speed"=w390, "Config Parameters.Heave Jog Speed"=w389) -> (w437:T12)
    }
    frame #11 {
      n363 = control-ref of="Mx"() -> (w468:refnum<vi>)
      n364 = control-ref of="My"() -> (w467:refnum<vi>)
      n365 = control-ref of="Mz"() -> (w466:refnum<vi>)
      n366 = control-ref of="Fx(N)"() -> (w465:refnum<vi>)
      n367 = control-ref of="Fy(N)"() -> (w464:refnum<vi>)
      n368 = control-ref of="Fz(N)"() -> (w463:refnum<vi>)
      n369 = control-ref of="Load Cell Temp"() -> (w439:refnum<vi>)
      n370 = control-ref of="ClearAll"() -> (w473:refnum<vi>)
      n371 = control-ref of="ZeroAll"() -> (w462:refnum<vi>)
      n372 = control-ref of="delete Handle"() -> (w452:refnum<vi>)
      n373 = control-ref of="Create Handle"() -> (w451:refnum<vi>)
      n374 = control-ref of="stop 6"() -> (w448:refnum<vi>)
      n375 = control-ref of="running_flag"() -> (w447:refnum<vi>)
      n376 = control-ref of="Save Dwell"() -> (w469:refnum<vi>)
      n377 = control-ref of="Acq Delay (ms)"() -> (w461:refnum<vi>)
      n378 = control-ref of="Burst Delay (ms)"() -> (w460:refnum<vi>)
      n379 = control-ref of="SN"() -> (w458:refnum<vi>)
      n380 = control-ref of="Port"() -> (w455:refnum<vi>)
      n381 = control-ref of="ft_udp_handle"() -> (w446:refnum<vi>)
      n382 = control-ref of="get-data-return"() -> (w445:refnum<vi>)
      n383 = control-ref of="get-range-return"() -> (w444:refnum<vi>)
      n384 = control-ref of="zero-return"() -> (w443:refnum<vi>)
      n385 = control-ref of="filter-return"() -> (w442:refnum<vi>)
      n386 = control-ref of="initial-return"() -> (w441:refnum<vi>)
      n387 = control-ref of="deleteHandle-result"() -> (w440:refnum<vi>)
      n388 = control-ref of="model"() -> (w459:refnum<vi>)
      n389 = control-ref of="Sensor IP"() -> (w456:refnum<vi>)
      n390 = control-ref of="Mz(Nm)"() -> (w472:refnum<vi>)
      n391 = control-ref of="My(Nm)"() -> (w471:refnum<vi>)
      n392 = control-ref of="Mx(Nm)"() -> (w470:refnum<vi>)
      n393 = control-ref of="FFx(N)"() -> (w457:refnum<vi>)
      n394 = control-ref of="FFy(N)"() -> (w454:refnum<vi>)
      n395 = control-ref of="Load(N)"() -> (w453:refnum<vi>)
      n396 = control-ref of="ft_data"() -> (w450:refnum<vi>)
      n397 = control-ref of="ft_range"() -> (w449:refnum<vi>)
      n398 = Bundle By Name(cluster=w475, "Loading Com Port.ClearAll"=w473, "Loading Com Port.Mz(Nm)"=w472, "Loading Com Port.My(Nm)"=w471, "Loading Com Port.Mx(Nm)"=w470, "Loading Com Port.Save Dwell"=w469, "Loading Com Port.Mx"=w468, "Loading Com Port.My"=w467, "Loading Com Port.Mz"=w466, "Loading Com Port.Fx(N)"=w465, "Loading Com Port.Fy(N)"=w464, "Loading Com Port.Fz(N)"=w463, "Loading Com Port.ZeroAll"=w462, "Loading Com Port.Acq Delay (ms)"=w461, "Loading Com Port.Burst Delay (ms)"=w460, "Loading Com Port.model"=w459, "Loading Com Port.SN"=w458, "Loading Com Port.FFx(N)"=w457, "Loading Com Port.Sensor IP"=w456, "Loading Com Port.Port"=w455, "Loading Com Port.FFy(N)"=w454, "Loading Com Port.Load(N)"=w453, "Loading Com Port.delete Handle"=w452, "Loading Com Port.Create Handle"=w451, "Loading Com Port.ft_data"=w450, "Loading Com Port.ft_range"=w449, "Loading Com Port.stop 6"=w448, "Loading Com Port.running_flag"=w447, "Loading Com Port.ft_udp_handle"=w446, "Loading Com Port.get-data-return"=w445, "Loading Com Port.get-range-return"=w444, "Loading Com Port.zero-return"=w443, "Loading Com Port.filter-return"=w442, "Loading Com Port.initial-return"=w441, "Loading Com Port.deleteHandle-result"=w440, "Loading Com Port.Load Cell Temp"=w439) -> (w474:T12)
    }
    frame #12 {
      n399 = control-ref of="Manual Write Heave & Surge"() -> (w477:refnum<vi>)
      n400 = control-ref of="Read Heave Temp"() -> (w500:refnum<vi>)
      n401 = control-ref of="error out Read"() -> (w512:refnum<vi>)
      n402 = control-ref of="error out Write"() -> (w507:refnum<vi>)
      n403 = control-ref of="SURGE POSE"() -> (w513:refnum<vi>)
      n404 = control-ref of="HEAVE POSE"() -> (w511:refnum<vi>)
      n405 = control-ref of="State"() -> (w510:refnum<vi>)
      n406 = control-ref of="Homed"() -> (w509:refnum<vi>)
      n407 = control-ref of="Sequence ID"() -> (w508:refnum<vi>)
      n408 = control-ref of="faultCode"() -> (w506:refnum<vi>)
      n409 = control-ref of="Ack ID"() -> (w505:refnum<vi>)
      n410 = control-ref of="SPEED"() -> (w504:refnum<vi>)
      n411 = control-ref of="Distance"() -> (w503:refnum<vi>)
      n412 = control-ref of="Mode Command"() -> (w502:refnum<vi>)
      n413 = control-ref of="SPARE 2"() -> (w499:refnum<vi>)
      n414 = control-ref of="SPARE 1"() -> (w498:refnum<vi>)
      n415 = control-ref of="Spare 15"() -> (w497:refnum<vi>)
      n416 = control-ref of="Spare 14"() -> (w496:refnum<vi>)
      n417 = control-ref of="Spare 13"() -> (w495:refnum<vi>)
      n418 = control-ref of="Spare 12"() -> (w494:refnum<vi>)
      n419 = control-ref of="Spare 11"() -> (w493:refnum<vi>)
      n420 = control-ref of="Spare 10"() -> (w492:refnum<vi>)
      n421 = control-ref of="Spare 9"() -> (w491:refnum<vi>)
      n422 = control-ref of="Spare 8"() -> (w490:refnum<vi>)
      n423 = control-ref of="Spare 7"() -> (w489:refnum<vi>)
      n424 = control-ref of="Spare 6"() -> (w488:refnum<vi>)
      n425 = control-ref of="Spare 5"() -> (w487:refnum<vi>)
      n426 = control-ref of="Spare 4"() -> (w486:refnum<vi>)
      n427 = control-ref of="Spare 3"() -> (w485:refnum<vi>)
      n428 = control-ref of="Spare 2"() -> (w484:refnum<vi>)
      n429 = control-ref of="Spare 1"() -> (w483:refnum<vi>)
      n430 = control-ref of="Node Id"() -> (w482:refnum<vi>)
      n431 = control-ref of="SPARE 3"() -> (w481:refnum<vi>)
      n432 = control-ref of="SPARE 4"() -> (w480:refnum<vi>)
      n433 = control-ref of="fwMajor"() -> (w479:refnum<vi>)
      n434 = control-ref of="fwMinor"() -> (w478:refnum<vi>)
      n435 = control-ref of="Heave and Surge Write"() -> (w476:refnum<vi>)
      n436 = control-ref of="Heave and Surge Read"() -> (w501:refnum<vi>)
      n437 = Bundle By Name(cluster=w515, "Heave AND Surge.SURGE POSE"=w513, "Heave AND Surge.error out Read"=w512, "Heave AND Surge.HEAVE POSE"=w511, "Heave AND Surge.State"=w510, "Heave AND Surge.Homed"=w509, "Heave AND Surge.Sequence ID"=w508, "Heave AND Surge.error out Write"=w507, "Heave AND Surge.faultCode"=w506, "Heave AND Surge.Ack ID"=w505, "Heave AND Surge.SPEED"=w504, "Heave AND Surge.Distance"=w503, "Heave AND Surge.Mode Command"=w502, "Heave AND Surge.Heave and Surge Read"=w501, "Heave AND Surge.Read Heave Temp"=w500, "Heave AND Surge.SPARE 2"=w499, "Heave AND Surge.SPARE 1"=w498, "Heave AND Surge.Spare 15"=w497, "Heave AND Surge.Spare 14"=w496, "Heave AND Surge.Spare 13"=w495, "Heave AND Surge.Spare 12"=w494, "Heave AND Surge.Spare 11"=w493, "Heave AND Surge.Spare 10"=w492, "Heave AND Surge.Spare 9"=w491, "Heave AND Surge.Spare 8"=w490, "Heave AND Surge.Spare 7"=w489, "Heave AND Surge.Spare 6"=w488, "Heave AND Surge.Spare 5"=w487, "Heave AND Surge.Spare 4"=w486, "Heave AND Surge.Spare 3"=w485, "Heave AND Surge.Spare 2"=w484, "Heave AND Surge.Spare 1"=w483, "Heave AND Surge.Node Id"=w482, "Heave AND Surge.SPARE 3"=w481, "Heave AND Surge.SPARE 4"=w480, "Heave AND Surge.fwMajor"=w479, "Heave AND Surge.fwMinor"=w478, "Heave AND Surge.Manual Write"=w477, "Heave AND Surge.Heave and Surge Write"=w476) -> (w514:T12)
    }
    frame #13 {
      n438 = control-ref of="Fine Tune Zone"() -> (w531:refnum<vi>)
      n439 = control-ref of="PID Delay (sec)"() -> (w530:refnum<vi>)
      n440 = control-ref of="Max_pos_limit"() -> (w529:refnum<vi>)
      n441 = control-ref of="Min_pos_limit"() -> (w528:refnum<vi>)
      n442 = control-ref of="i_limit"() -> (w527:refnum<vi>)
      n443 = control-ref of="pct_scale"() -> (w518:refnum<vi>)
      n444 = control-ref of="Deadband"() -> (w526:refnum<vi>)
      n445 = control-ref of="Kd"() -> (w525:refnum<vi>)
      n446 = control-ref of="Ki"() -> (w524:refnum<vi>)
      n447 = control-ref of="Kp"() -> (w523:refnum<vi>)
      n448 = control-ref of="Current Position"() -> (w522:refnum<vi>)
      n449 = control-ref of="Set Load"() -> (w521:refnum<vi>)
      n450 = control-ref of="Current Load"() -> (w520:refnum<vi>)
      n451 = control-ref of="Pulse delta"() -> (w519:refnum<vi>)
      n452 = control-ref of="Init Step"() -> (w517:refnum<vi>)
      n453 = control-ref of="Max Step Linit"() -> (w516:refnum<vi>)
      n454 = Bundle By Name(cluster=w533, "New PID LOGIC.Fine Tune Zone"=w531, "New PID LOGIC.PID SDelay"=w530, "New PID LOGIC.Max_pos_limit"=w529, "New PID LOGIC.Min_pos_limit"=w528, "New PID LOGIC.i_limit"=w527, "New PID LOGIC.pct_scale"=w518, "New PID LOGIC.Deadband"=w526, "New PID LOGIC.Kd"=w525, "New PID LOGIC.Ki"=w524, "New PID LOGIC.Kp"=w523, "New PID LOGIC.Current Position"=w522, "New PID LOGIC.Set Load"=w521, "New PID LOGIC.Current Load"=w520, "New PID LOGIC.Pulse delta"=w519, "New PID LOGIC.Init Step"=w517, "New PID LOGIC.Max Step Linit"=w516) -> (w532:T12)
    }
  }
  n455 = call <userlib>:"Fit VI window to Largest Dec.vi"() -> ("error out"=w43:errorcluster, "dup VI Ref"=w40:refnum<vi>)  [unwired: 6 in]
  n456 = invoke on="Invoke Node" class="VI" method="FP.Run-Time Position.Maximized"(reference=w40, error in=w43) -> (error out=w42:errorcluster)  [unwired: 2 in, 3 out]
  n457 = call <vilib>:"Clear Errors.vi"("error in (no error)"=w42) -> ("error out"=w41:errorcluster)  [unwired: 5 in, 1 out]
  n458 = control-ref of="This VI"() -> (w46:refnum<vi>)
  n459 = invoke on="Invoke Node" class="VI" method="Default Vals.Reinit All"(reference=w46, error in=w41) -> (reference out=w44:refnum<vi>, error out=w45:errorcluster)  [unwired: 1 in, 1 out]
  n460 = Close Reference(reference=w44, error in (no error)=w45) -> (error out=w39:errorcluster)
  n461 = call "Create User Event - Stop.vi"("error in (no error)"=w39) -> ("error out"=w14:errorcluster, "User Event - Stop"=w26:refnum<user-event>)  [unwired: 9 in]
  n462 = call "main screen queue out Unitest.vi"("error in (no error)"=w14) -> ("error out"=w66:errorcluster, "output Queue"=w38:T13)  [unwired: 9 in]
  n463 = Unbundle By Name(w38) -> ("UI Loop"=w64:refnum<queue>)
  n464 = Unbundle By Name(w38) -> ("LOAD COM LOOP"=w36:refnum<queue>)
  n465 = Unbundle By Name(w38) -> ("SWAY MOTOR COM LOOP"=w35:refnum<queue>)
  n466 = Unbundle By Name(w38) -> ("HEAVE MOTOR COM LOOP"=w18:refnum<queue>)
  n467 = Unbundle By Name(w38) -> ("TEMPERATURE COM LOOP"=w33:refnum<queue>)
  n468 = Unbundle By Name(w38) -> ("RAMP MOTOR COM LOOP"=w30:refnum<queue>)
  n469 = Unbundle By Name(w38) -> ("ECR PORT"=w29:refnum<queue>)
  n470 = Unbundle By Name(w38) -> ("HUMIDITY COM PORT"=w28:refnum<queue>)
  n471 = Unbundle By Name(w38) -> ("PROGRAM LOOP"=w27:refnum<queue>)
  n472 = Unbundle By Name(w38) -> ("MONITOR LOOP"=w25:refnum<queue>)
  n473 = Unbundle By Name(w38) -> ("LOAD PID"=w24:refnum<queue>)
  n474 = Unbundle By Name(w38) -> ("REPORT"=w23:refnum<queue>)
  n475 = register-events(w26) -> (reference out=w58:refnum<event-registration>, error out=w56:errorcluster)  [unwired: 2 in]
  n476 = Merge Errors(w56, w66) -> (w57:errorcluster)
  n477 = while {
    tunnel: w64 -> [w541]
    shift-right: [w539] -> w61
    shift-left: w58 -> [w540]
    tunnel: [w535] -> w59
    stop <- w537 stop-if-true
    # "Event Handling Loop"
    n478 = event shown="[35] \"STOP\": Value Change" {
      selector: w540 -> [_ _ _ _ _ _ _ _ _ _ _ _ _ _ _ _ _ _ _ _ _ _ _ _ _ _ _ _ _ _ _ _ _ _ _ _ _ _ _]
      dyn-events: [_ _ _ _ _ _ _ _ _ _ _ _ _ _ _ _ _ _ _ _ _ _ _ _ _ _ _ _ _ _ _ _ _ _ _ _ _ _ _] -> w539
      timeout: 100 -> [_ _ _ _ _ _ _ _ _ _ _ _ _ _ _ _ _ _ _ _ _ _ _ _ _ _ _ _ _ _ _ _ _ _ _ _ _ _ _]
      tunnel: [_ _ _ _ _ _ _ _ _ _ _ _ _ _ _ _ _ _ _ _ _ _ _ _ _ _ _ _ _ _ _ _ _ _ _ _ _ _ TRUE ("Discard?")] -> w537
      tunnel: w541 -> [w546 w550 w555 w560 w565 w570 w575 w580 w585 w590 w595 w600 w605 w610 w615 w620 w625 w630 w635 w640 w645 w650 w655 w660 w665 w670 w675 w680 w685 w690 w695 w700 w705 w710 w715 w720 w723 w728 w730]
      tunnel: [w545 w548 w553 w558 w563 w568 w573 w578 w583 w588 w593 w598 w603 w608 w613 w618 w623 w628 w633 w638 w643 w648 w653 w658 w663 w668 w673 w678 w683 w688 w693 w698 w703 w708 w713 w718 _ w727 _] -> w538
      tunnel: [w544 w549 w554 w559 w564 w569 w574 w579 w584 w589 w594 w599 w604 w609 w614 w619 w624 w629 w634 w639 w644 w649 w654 w659 w664 w669 w674 w679 w684 w689 w694 w699 w704 w709 w714 w719 w723 w726 w730] -> w536
      event Panel Close? {
        n479 = event-data() -> ()  [unwired: 1 in, 1 out]
        n480 = call-poly "Enqueue Message.vi"("Priority Message? (F)"=TRUE, "Message"="Confirm Quit", "Message Queue"=w546) -> ("error out"=w545:errorcluster, "dup Message Queue"=w544:refnum<queue>)  [unwired: 7 in]
        n481 = event-data("Discard?"=TRUE) -> ()  [unwired: 1 in, 1 out]
      }
      event Timeout {
        n482 = event-data() -> ()  [unwired: 1 in, 1 out]
        n483 = call-poly "Enqueue Message.vi"("Priority Message? (F)"=TRUE, "Message"="Time Out", "Message Queue"=w550) -> ("error out"=w548:errorcluster, "dup Message Queue"=w549:refnum<queue>)  [unwired: 7 in]
      }
      event "SAVE  2": Value Change {
        n484 = event-data() -> ()  [unwired: 1 in, 1 out]
        n485 = call-poly "Enqueue Message.vi"("Priority Message? (F)"=TRUE, "Message"="Service Save", "Message Queue"=w555) -> ("error out"=w553:errorcluster, "dup Message Queue"=w554:refnum<queue>)  [unwired: 7 in]
      }
      event "Home": Value Change {
        n486 = event-data() -> ()  [unwired: 1 in, 1 out]
        n487 = call-poly "Enqueue Message.vi"("Priority Message? (F)"=TRUE, "Message"="HOME", "Message Queue"=w560) -> ("error out"=w558:errorcluster, "dup Message Queue"=w559:refnum<queue>)  [unwired: 7 in]
      }
      event "Platform Settings": Value Change {
        n488 = event-data() -> ()  [unwired: 1 in, 1 out]
        n489 = call-poly "Enqueue Message.vi"("Priority Message? (F)"=TRUE, "Message"="Platform Setting", "Message Queue"=w565) -> ("error out"=w563:errorcluster, "dup Message Queue"=w564:refnum<queue>)  [unwired: 7 in]
      }
      event "Configure": Value Change {
        n490 = event-data() -> ()  [unwired: 1 in, 1 out]
        n491 = call-poly "Enqueue Message.vi"("Priority Message? (F)"=TRUE, "Message"="Configure", "Message Queue"=w570) -> ("error out"=w568:errorcluster, "dup Message Queue"=w569:refnum<queue>)  [unwired: 7 in]
      }
      event "Analysis": Value Change {
        n492 = event-data() -> ()  [unwired: 1 in, 1 out]
        n493 = call-poly "Enqueue Message.vi"("Priority Message? (F)"=TRUE, "Message"="Analysis", "Message Queue"=w575) -> ("error out"=w573:errorcluster, "dup Message Queue"=w574:refnum<queue>)  [unwired: 7 in]
      }
      event "service 2": Value Change {
        n494 = event-data() -> ()  [unwired: 1 in, 1 out]
        n495 = call-poly "Enqueue Message.vi"("Priority Message? (F)"=TRUE, "Message"="service 2", "Message Queue"=w580) -> ("error out"=w578:errorcluster, "dup Message Queue"=w579:refnum<queue>)  [unwired: 7 in]
      }
      event "Auto": Value Change {
        n496 = event-data() -> ()  [unwired: 1 in, 1 out]
        n497 = call-poly "Enqueue Message.vi"("Priority Message? (F)"=TRUE, "Message"="Auto", "Message Queue"=w585) -> ("error out"=w583:errorcluster, "dup Message Queue"=w584:refnum<queue>)  [unwired: 7 in]
      }
      event "Select Load Head": Value Change {
        n498 = event-data() -> ()  [unwired: 1 in, 1 out]
        n499 = call-poly "Enqueue Message.vi"("Priority Message? (F)"=TRUE, "Message"="Select Load Head", "Message Queue"=w590) -> ("error out"=w588:errorcluster, "dup Message Queue"=w589:refnum<queue>)  [unwired: 7 in]
      }
      event "com 3": Value Change {
        n500 = event-data() -> ()  [unwired: 1 in, 1 out]
        n501 = call-poly "Enqueue Message.vi"("Priority Message? (F)"=TRUE, "Message"="com 3", "Message Queue"=w595) -> ("error out"=w593:errorcluster, "dup Message Queue"=w594:refnum<queue>)  [unwired: 7 in]
      }
      event "Loading Mode": Value Change {
        n502 = event-data() -> ()  [unwired: 1 in, 1 out]
        n503 = call-poly "Enqueue Message.vi"("Priority Message? (F)"=TRUE, "Message"="Loading Mode", "Message Queue"=w600) -> ("error out"=w598:errorcluster, "dup Message Queue"=w599:refnum<queue>)  [unwired: 7 in]
      }
      event "SSP 0.3": Value Change {
        n504 = event-data() -> ()  [unwired: 1 in, 1 out]
        n505 = call-poly "Enqueue Message.vi"("Priority Message? (F)"=TRUE, "Message"="SSP 0.3", "Message Queue"=w605) -> ("error out"=w603:errorcluster, "dup Message Queue"=w604:refnum<queue>)  [unwired: 7 in]
      }
      event "SSP 0.5": Value Change {
        n506 = event-data() -> ()  [unwired: 1 in, 1 out]
        n507 = call-poly "Enqueue Message.vi"("Priority Message? (F)"=TRUE, "Message"="SSP 0.5", "Message Queue"=w610) -> ("error out"=w608:errorcluster, "dup Message Queue"=w609:refnum<queue>)  [unwired: 7 in]
      }
      event "SSP 0.75": Value Change {
        n508 = event-data() -> ()  [unwired: 1 in, 1 out]
        n509 = call-poly "Enqueue Message.vi"("Priority Message? (F)"=TRUE, "Message"="SSP 0.75", "Message Queue"=w615) -> ("error out"=w613:errorcluster, "dup Message Queue"=w614:refnum<queue>)  [unwired: 7 in]
      }
      event "LHBack": Value Change {
        n510 = event-data() -> ()  [unwired: 1 in, 1 out]
        n511 = call-poly "Enqueue Message.vi"("Priority Message? (F)"=TRUE, "Message"="LHBack", "Message Queue"=w620) -> ("error out"=w618:errorcluster, "dup Message Queue"=w619:refnum<queue>)  [unwired: 7 in]
      }
      event "LHNext": Value Change {
        n512 = event-data() -> ()  [unwired: 1 in, 1 out]
        n513 = call-poly "Enqueue Message.vi"("Priority Message? (F)"=TRUE, "Message"="LHNext", "Message Queue"=w625) -> ("error out"=w623:errorcluster, "dup Message Queue"=w624:refnum<queue>)  [unwired: 7 in]
      }
      event "Rot Ver": Value Change {
        n514 = event-data() -> ()  [unwired: 1 in, 1 out]
        n515 = call-poly "Enqueue Message.vi"("Priority Message? (F)"=TRUE, "Message"="Rot Ver", "Message Queue"=w630) -> ("error out"=w628:errorcluster, "dup Message Queue"=w629:refnum<queue>)  [unwired: 7 in]
      }
      event "Scratch": Value Change {
        n516 = event-data() -> ()  [unwired: 1 in, 1 out]
        n517 = call-poly "Enqueue Message.vi"("Priority Message? (F)"=TRUE, "Message"="Scratch", "Message Queue"=w635) -> ("error out"=w633:errorcluster, "dup Message Queue"=w634:refnum<queue>)  [unwired: 7 in]
      }
      event "Motion Mode:": Value Change {
        n518 = event-data() -> ()  [unwired: 1 in, 1 out]
        n519 = call-poly "Enqueue Message.vi"("Priority Message? (F)"=TRUE, "Message"="Motion Mode:", "Message Queue"=w640) -> ("error out"=w638:errorcluster, "dup Message Queue"=w639:refnum<queue>)  [unwired: 7 in]
      }
      event "MMBack": Value Change {
        n520 = event-data() -> ()  [unwired: 1 in, 1 out]
        n521 = call-poly "Enqueue Message.vi"("Priority Message? (F)"=TRUE, "Message"="MMBack", "Message Queue"=w645) -> ("error out"=w643:errorcluster, "dup Message Queue"=w644:refnum<queue>)  [unwired: 7 in]
      }
      event "MMNext": Value Change {
        n522 = event-data() -> ()  [unwired: 1 in, 1 out]
        n523 = call-poly "Enqueue Message.vi"("Priority Message? (F)"=TRUE, "Message"="MMNext", "Message Queue"=w650) -> ("error out"=w648:errorcluster, "dup Message Queue"=w649:refnum<queue>)  [unwired: 7 in]
      }
      event "APBack": Value Change {
        n524 = event-data() -> ()  [unwired: 1 in, 1 out]
        n525 = call-poly "Enqueue Message.vi"("Priority Message? (F)"=TRUE, "Message"="APBack", "Message Queue"=w655) -> ("error out"=w653:errorcluster, "dup Message Queue"=w654:refnum<queue>)  [unwired: 7 in]
      }
      event "SNext": Value Change {
        n526 = event-data() -> ()  [unwired: 1 in, 1 out]
        n527 = call-poly "Enqueue Message.vi"("Priority Message? (F)"=TRUE, "Message"="SNext", "Message Queue"=w660) -> ("error out"=w658:errorcluster, "dup Message Queue"=w659:refnum<queue>)  [unwired: 7 in]
      }
      event "ZeroAll": Value Change {
        n528 = event-data() -> ()  [unwired: 1 in, 1 out]
        n529 = call-poly "Enqueue Message.vi"("Priority Message? (F)"=TRUE, "Message"="ZeroAll", "Message Queue"=w665) -> ("error out"=w663:errorcluster, "dup Message Queue"=w664:refnum<queue>)  [unwired: 7 in]
      }
      event "Enable Platform": Value Change {
        n530 = event-data() -> ()  [unwired: 1 in, 1 out]
        n531 = call-poly "Enqueue Message.vi"("Priority Message? (F)"=TRUE, "Message"="Enable Platform", "Message Queue"=w670) -> ("error out"=w668:errorcluster, "dup Message Queue"=w669:refnum<queue>)  [unwired: 7 in]
      }
      event "Heave Up main": Value Change {
        n532 = event-data() -> ()  [unwired: 1 in, 1 out]
        n533 = call-poly "Enqueue Message.vi"("Priority Message? (F)"=TRUE, "Message"="Heave Up main", "Message Queue"=w675) -> ("error out"=w673:errorcluster, "dup Message Queue"=w674:refnum<queue>)  [unwired: 7 in]
      }
      event "Heave Down Main": Value Change {
        n534 = event-data() -> ()  [unwired: 1 in, 1 out]
        n535 = call-poly "Enqueue Message.vi"("Priority Message? (F)"=TRUE, "Message"="Heave Down Main", "Message Queue"=w680) -> ("error out"=w678:errorcluster, "dup Message Queue"=w679:refnum<queue>)  [unwired: 7 in]
      }
      event "Manual Write Heave & Surge": Value Change {
        n536 = event-data() -> ()  [unwired: 1 in, 1 out]
        n537 = call-poly "Enqueue Message.vi"("Priority Message? (F)"=TRUE, "Message"="Manual Write Heave & Surge", "Message Queue"=w685) -> ("error out"=w683:errorcluster, "dup Message Queue"=w684:refnum<queue>)  [unwired: 7 in]
      }
      event "Surge Backward Main": Value Change {
        n538 = event-data() -> ()  [unwired: 1 in, 1 out]
        n539 = call-poly "Enqueue Message.vi"("Priority Message? (F)"=TRUE, "Message"="Surge Backward Main", "Message Queue"=w690) -> ("error out"=w688:errorcluster, "dup Message Queue"=w689:refnum<queue>)  [unwired: 7 in]
      }
      event "Surge Forward Main": Value Change {
        n540 = event-data() -> ()  [unwired: 1 in, 1 out]
        n541 = call-poly "Enqueue Message.vi"("Priority Message? (F)"=TRUE, "Message"="Surge Forward Main", "Message Queue"=w695) -> ("error out"=w693:errorcluster, "dup Message Queue"=w694:refnum<queue>)  [unwired: 7 in]
      }
      event "Load En": Value Change {
        n542 = event-data() -> ()  [unwired: 1 in, 1 out]
        n543 = call-poly "Enqueue Message.vi"("Priority Message? (F)"=TRUE, "Message"="Load En", "Message Queue"=w700) -> ("error out"=w698:errorcluster, "dup Message Queue"=w699:refnum<queue>)  [unwired: 7 in]
      }
      event "apply load": Value Change {
        n544 = event-data() -> ()  [unwired: 1 in, 1 out]
        n545 = call-poly "Enqueue Message.vi"("Priority Message? (F)"=TRUE, "Message"="apply load", "Message Queue"=w705) -> ("error out"=w703:errorcluster, "dup Message Queue"=w704:refnum<queue>)  [unwired: 7 in]
      }
      event "BACK": Value Change {
        n546 = event-data() -> ()  [unwired: 1 in, 1 out]
        n547 = call-poly "Enqueue Message.vi"("Priority Message? (F)"=TRUE, "Message"="BACK", "Message Queue"=w710) -> ("error out"=w708:errorcluster, "dup Message Queue"=w709:refnum<queue>)  [unwired: 7 in]
      }
      event "Start Test": Value Change {
        n548 = event-data() -> ()  [unwired: 1 in, 1 out]
        n549 = call-poly "Enqueue Message.vi"("Priority Message? (F)"=TRUE, "Message"="Start Test", "Message Queue"=w715) -> ("error out"=w713:errorcluster, "dup Message Queue"=w714:refnum<queue>)  [unwired: 7 in]
      }
      event "STOP": Value Change {
        n550 = event-data() -> ()  [unwired: 1 in, 1 out]
        n551 = call-poly "Enqueue Message.vi"("Priority Message? (F)"=TRUE, "Message"="STOP", "Message Queue"=w720) -> ("error out"=w718:errorcluster, "dup Message Queue"=w719:refnum<queue>)  [unwired: 7 in]
      }
      event Application Instance Close {
        # "#CodeRecommended - When a project closes, all VIs within that project are aborted and leave memory. However, any code placed in this event frame is guaranteed to run to completion, so add any cleanup code that absolutely must happen here."
        n552 = event-data() -> ()  [unwired: 1 in, 1 out]
      }
      event "EXIT": Value Change {
        n553 = event-data() -> ()  [unwired: 1 in, 1 out]
        n554 = call-poly "Enqueue Message.vi"("Priority Message? (F)"=TRUE, "Message"="Exit", "Message Queue"=w728) -> ("error out"=w727:errorcluster, "dup Message Queue"=w726:refnum<queue>)  [unwired: 7 in]
      }
      event User Event {
        # "The Message Handling Loop processed an \"Exit\" message, which fired this event to stop the Event Handling Loop."
        n555 = event-data() -> ()  [unwired: 1 in, 1 out]
      }
    }
    n556 = call "LAB-IQ Error Handler - Event Handling Loop.vi"("error in (no error)"=w538, "Message Queue"=w536) -> ("dup error in"=w535:errorcluster)  [unwired: 8 in, 1 out]
  }
  n557 = while {
    shift-right: [w745] -> _
    shift-left: w7 -> [w746]
    tunnel: [w739] -> _
    tunnel: w24 -> [w737]
    tunnel: w14 -> [w736]
    tunnel: w26 -> [w735]
    shift-right: [w734] -> _
    shift-left: w1 -> [w732]
    shift-right: [w733] -> _
    shift-left: w1 -> [w731]
    stop <- w744 stop-if-true
    # "Load Pid  Handling Loop"
    n558 = call "Dequeue Message.vi"("error in (no error)"=w736, "Message Queue"=w737) -> ("error out"=w743:errorcluster, "Message Data"=w741:variant, "Message"=w742:string, "dup Message Queue"=w740:refnum<queue>)  [unwired: 6 in]
    n559 = case "Message Cases" shown="\"Load Pid Main\"" w742 {
      selector: w742 -> [_ _ _ _ _ w935]
      tunnel: w740 -> [w748 w773 _ w920 w933 _]
      tunnel: w743 -> [w751 w771 w916 w924 w927 _]
      tunnel: [w752 w774 w910 w922 w929 w936] -> w738
      tunnel: w746 -> [w750 w760 w915 w923 w932 w937]
      tunnel: [w750 w760 w915 w923 w932 w937] -> w745
      tunnel: [_ _ _ _ TRUE _] -> w744
      tunnel: w741 -> [_ _ w914 _ _ _]
      tunnel: w735 -> [_ _ _ _ w926 _]
      tunnel: [w747 w756 w909 w917 w925 w934] -> w734
      tunnel: [w747 w755 w909 w917 w925 w934] -> w733
      tunnel: w732 -> [w747 w754 _ _ _ _]
      tunnel: w731 -> [_ w753 _ _ _ _]
      frame "init" {
        # "Initialize - All initialization work should take place in this message, since other loops can potentially enqueue messages that execute immediately after this one."
        n560 = call-poly "Enqueue Message.vi"("error in (no error)"=w751, "Message"="Load Pid Main", "Message Queue"=w748) -> ("error out"=w752:errorcluster)  [unwired: 7 in, 1 out]
      }
      frame "Load Pid Main" {
        n561 = Unbundle By Name(w760) -> ("Main Screen.Load En"=w766:refnum<vi>)
        n562 = Unbundle By Name(w760) -> ("PID.apply load"=w761:refnum<vi>)
        n563 = property class="Bool (strict)"(reference=w766) -> (reference out=w764:refnum<vi>, error out=w765:errorcluster, "Value"=w759:bool)  [unwired: 1 in]
        n564 = property class="Bool (strict)"(reference=w761) -> (reference out=w763:refnum<vi>, error out=w762:errorcluster, "Value"=w758:bool)  [unwired: 1 in]
        n565 = Close Reference(reference=w764, error in (no error)=w765) -> ()  [unwired: 1 out]
        n566 = Close Reference(reference=w763, error in (no error)=w762) -> ()  [unwired: 1 out]
        n567 = Or(x=w759, y=w758) -> (x .or. y?=w757:bool)
        n568 = case shown="True" w757 {
          tunnel: w771 -> [w778 w893]
          tunnel: [w778 w892] -> w767
          tunnel: w760 -> [_ w894]
          tunnel: [w777 w896] -> w756
          tunnel: [w776 w895] -> w755
          tunnel: w754 -> [w777 w891]
          tunnel: w753 -> [w776 w890]
          frame False {
            n569 = local write "Checkbox"(TRUE ("Checkbox")) -> ()
          }
          frame True {
            n570 = Unbundle By Name(w894) -> ("New PID LOGIC.PID SDelay"=w887:refnum<vi>)
            n571 = Unbundle By Name(w894) -> ("PID.Enter ByPass Load"=w873:refnum<vi>)
            n572 = Unbundle By Name(w894) -> ("Main Screen.Set Load (N)"=w880:refnum<vi>)
            n573 = Unbundle By Name(w894) -> ("PID.Bypass Load"=w868:refnum<vi>)
            n574 = Unbundle By Name(w894) -> ("Heave AND Surge.HEAVE POSE"=w864:refnum<vi>)
            n575 = Unbundle By Name(w894) -> ("New PID LOGIC.Kp"=w860:refnum<vi>)
            n576 = Unbundle By Name(w894) -> ("New PID LOGIC.Ki"=w854:refnum<vi>)
            n577 = Unbundle By Name(w894) -> ("New PID LOGIC.Kd"=w852:refnum<vi>)
            n578 = Unbundle By Name(w894) -> ("New PID LOGIC.Deadband"=w846:refnum<vi>)
            n579 = Unbundle By Name(w894) -> ("New PID LOGIC.Deadband"=w844:refnum<vi>)
            n580 = Unbundle By Name(w894) -> ("New PID LOGIC.Init Step"=w838:refnum<vi>)
            n581 = Unbundle By Name(w894) -> ("New PID LOGIC.Max Step Linit"=w834:refnum<vi>)
            n582 = Unbundle By Name(w894) -> ("New PID LOGIC.i_limit"=w828:refnum<vi>)
            n583 = Unbundle By Name(w894) -> ("New PID LOGIC.Min_pos_limit"=w826:refnum<vi>)
            n584 = Unbundle By Name(w894) -> ("New PID LOGIC.Max_pos_limit"=w820:refnum<vi>)
            n585 = Unbundle By Name(w894) -> ("New PID LOGIC.Fine Tune Zone"=w818:refnum<vi>)
            n586 = Unbundle By Name(w894) -> ("PID.Vertical load (N)"=w784:refnum<vi>)
            n587 = property class="DigNum (strict)"(reference=w887) -> (reference out=w889:refnum<vi>, error out=w888:errorcluster, "Value"=w886:dbl)  [unwired: 1 in]
            n588 = property class="DigNum (strict)"(reference=w873) -> (reference out=w871:refnum<vi>, error out=w872:errorcluster, "Value"=w866:dbl)  [unwired: 1 in]
            n589 = property class="DigNum (strict)"(reference=w880) -> (reference out=w882:refnum<vi>, error out=w881:errorcluster, "Value"=w865:dbl)  [unwired: 1 in]
            n590 = property class="DigNum (strict)"(reference=w864) -> (reference out=w862:refnum<vi>, error out=w863:errorcluster, "Value"=w861:sgl)  [unwired: 1 in]
            n591 = property class="DigNum (strict)"(reference=w784) -> (reference out=w785:refnum<vi>, error out=w786:errorcluster, "Value"=w783:dbl)  [unwired: 1 in]
            n592 = property class="Bool (strict)"(reference=w868) -> (reference out=w870:refnum<vi>, error out=w869:errorcluster, "Value"=w867:bool)  [unwired: 1 in]
            n593 = property class="DigNum (strict)"(reference=w860) -> (reference out=w858:refnum<vi>, error out=w859:errorcluster, "Value"=w857:dbl)  [unwired: 1 in]
            n594 = property class="DigNum (strict)"(reference=w854) -> (reference out=w856:refnum<vi>, error out=w855:errorcluster, "Value"=w853:dbl)  [unwired: 1 in]
            n595 = property class="DigNum (strict)"(reference=w852) -> (reference out=w850:refnum<vi>, error out=w851:errorcluster, "Value"=w849:dbl)  [unwired: 1 in]
            n596 = property class="DigNum (strict)"(reference=w846) -> (reference out=w848:refnum<vi>, error out=w847:errorcluster, "Value"=w845:dbl)  [unwired: 1 in]
            n597 = property class="DigNum (strict)"(reference=w844) -> (reference out=w842:refnum<vi>, error out=w843:errorcluster, "Value"=w841:dbl)  [unwired: 1 in]
            n598 = property class="DigNum (strict)"(reference=w838) -> (reference out=w840:refnum<vi>, error out=w839:errorcluster, "Value"=w837:dbl)  [unwired: 1 in]
            n599 = property class="DigNum (strict)"(reference=w834) -> (reference out=w832:refnum<vi>, error out=w833:errorcluster, "Value"=w831:dbl)  [unwired: 1 in]
            n600 = property class="DigNum (strict)"(reference=w828) -> (reference out=w830:refnum<vi>, error out=w829:errorcluster, "Value"=w827:dbl)  [unwired: 1 in]
            n601 = property class="DigNum (strict)"(reference=w826) -> (reference out=w824:refnum<vi>, error out=w825:errorcluster, "Value"=w823:dbl)  [unwired: 1 in]
            n602 = property class="DigNum (strict)"(reference=w820) -> (reference out=w822:refnum<vi>, error out=w821:errorcluster, "Value"=w819:dbl)  [unwired: 1 in]
            n603 = property class="DigNum (strict)" props=["Value"](reference=w818) -> (reference out=w816:refnum<vi>, error out=w817:errorcluster)  [unwired: 1 in, 1 out]
            n604 = case shown="False" "Checkbox" {
              selector: "Checkbox" -> [_ w900]
              tunnel: [0.0 1.0] -> w835
              frame False {
              }
              frame True {
                n605 = Not(x=w900) -> (.not. x?=w899:bool)
                n606 = local write "Checkbox"(w899) -> ()
              }
            }
            n607 = Close Reference(reference=w889, error in (no error)=w888) -> ()  [unwired: 1 out]
            n608 = Close Reference(reference=w871, error in (no error)=w872) -> ()  [unwired: 1 out]
            n609 = Close Reference(reference=w882, error in (no error)=w881) -> ()  [unwired: 1 out]
            n610 = Close Reference(reference=w785, error in (no error)=w786) -> ()  [unwired: 1 out]
            n611 = Close Reference(reference=w870, error in (no error)=w869) -> ()  [unwired: 1 out]
            n612 = Close Reference(reference=w862, error in (no error)=w863) -> ()  [unwired: 1 out]
            n613 = Close Reference(reference=w858, error in (no error)=w859) -> ()  [unwired: 1 out]
            n614 = Close Reference(reference=w830, error in (no error)=w829) -> ()  [unwired: 1 out]
            n615 = Close Reference(reference=w856, error in (no error)=w855) -> ()  [unwired: 1 out]
            n616 = Close Reference(reference=w824, error in (no error)=w825) -> ()  [unwired: 1 out]
            n617 = Close Reference(reference=w822, error in (no error)=w821) -> ()  [unwired: 1 out]
            n618 = Close Reference(reference=w816, error in (no error)=w817) -> ()  [unwired: 1 out]
            n619 = call <vilib>:"High Resolution Polling Wait.vi"("seconds to wait"=w886) -> ()  [unwired: 10 in, 1 out]
            n620 = Close Reference(reference=w848, error in (no error)=w847) -> ()  [unwired: 1 out]
            n621 = Close Reference(reference=w850, error in (no error)=w851) -> ()  [unwired: 1 out]
            n622 = Close Reference(reference=w842, error in (no error)=w843) -> ()  [unwired: 1 out]
            n623 = Close Reference(reference=w840, error in (no error)=w839) -> ()  [unwired: 1 out]
            n624 = Close Reference(reference=w832, error in (no error)=w833) -> ()  [unwired: 1 out]
            n625 = Select(t=w866, s=w867, f=w865) -> (s? t:f=w792:dbl)
            n626 = formula code="// =====================================================================\n// AUTOMATICALLY SCALING PID CONTROL LOGIC FOR LABVIEW FORMULA NODE\n// Profile Adaptability: Constant, Step, & Ramp (2 N to 500 N)\n// Direction Polarity: Increasing count moves DOWN (Increases Load)\n// =====================================================================\n\n// --- Internal Variable Declarations ---\nfloat error;\nfloat deadband_value;\nfloat fine_tune_zone;\nfloat derivative;\nfloat pid_output;\nfloat step_change;\nfloat abs_error;\nfloat dynamic_limit;\nfloat pid_sign;\nfloat abs_pid;\nfloat active_scale_reference;\n\n// 1. Calculate Error State\nerror = set_load - current_load;\nabs_error = (error < 0) ? -error : error;\n\n// 2. Establish Scale Reference (Safeguards against zero-crossings or low-load ramp profiles)\nactive_scale_reference = (set_load < 2.0) ? 2.0 : set_load;\n\n// 3. Compute Dynamic Deadband Threshold with Noise Floor Guard\ndeadband_value = active_scale_reference * (deadband_pct / pct_scale);\nif (deadband_value < 0) {\n    deadband_value = -deadband_value; \n}\nif (deadband_value < min_deadband_floor) {\n    deadband_value = min_deadband_floor; // Prevents low-load sensor noise chattering at 2 N\n}\n\n// 4. Compute Dynamic Fine-Tune Zone with Floor Guard\nfine_tune_zone = active_scale_reference * (fine_tune_pct / pct_scale);\nif (fine_tune_zone < 0) {\n    fine_tune_zone = -fine_tune_zone;\n}\nif (fine_tune_zone < min_finetune_floor) {\n    fine_tune_zone = min_finetune_floor; // Slows down approach smoothly on 2 N targets\n}\n\n// 5. Main Control State Machine\n// ---------------------------------------------------------------------\n// Condition A: Initial Move (Establish baseline and force initial step)\n// ---------------------------------------------------------------------\nif (init_move == 1) {\n    step_change = init_step; \n    integral_out = 0.0;               // Reset integral memory on start\n    prev_error_out = error;           // Initialize derivative baseline\n    \n    if (error > 0) {\n        next_command = current_position + step_change;\n    } else {\n        next_command = current_position - step_change;\n    }\n    pulse_delta = next_command - current_position;\n}\n// ---------------------------------------------------------------------\n// Condition B: Within Target Deadband (Freeze State / Zero Energy)\n// ---------------------------------------------------------------------\nelse if (abs_error <= deadband_value) {\n    step_change = 0.0;\n    next_command = current_position; // Lock to current physical position\n    integral_out = integral_in;       // Freeze integral to prevent drift\n    prev_error_out = error;           // Keep derivative baseline fresh\n    pulse_delta = 0.0;\n} \n// ---------------------------------------------------------------------\n// Condition C: Active PID Control Zone\n// ---------------------------------------------------------------------\nelse {\n    // A. Track Integral with strict Anti-Windup Limits\n    integral_out = integral_in + error;\n    if (integral_out > i_limit) {\n        integral_out = i_limit;\n    } else if (integral_out < -i_limit) {\n        integral_out = -i_limit;\n    }\n\n    // B. Calculate Derivative (Tracks rate of change of error - crucial for RAMP tracking)\n    derivative = error - prev_error_in;\n    prev_error_out = error; \n\n    // C. Execute Raw PID Equation\n    pid_output = (error * kp) + (integral_out * ki) + (derivative * kd);\n    \n    // D. Extract Mathematical Sign and Magnitude\n    pid_sign = (pid_output >= 0) ? 1.0 : -1.0;\n    abs_pid = (pid_output < 0) ? -pid_output : pid_output;\n\n    // E. Continuous Linear Ramp-Down Ceiling (Smooth adaptation for moving ramp profiles)\n    if (abs_error < active_scale_reference) {\n        dynamic_limit = max_step_limit * (abs_error / active_scale_reference);\n        if (dynamic_limit < 1.0) {\n            dynamic_limit = 1.0; // Minimum microstep velocity floor\n        }\n    } else {\n        dynamic_limit = max_step_limit; // Maximum speed deployment for STEP jumps\n    }\n\n    // F. Apply Smooth Step Control & Fine Tuning Zone\n    if (abs_error <= fine_tune_zone) {\n        step_change = 1.0; // Forced 1-Count Precision micro-stepping close to target\n    } else {\n        if (abs_pid < dynamic_limit) {\n            step_change = abs_pid; // Decay step size perfectly near steady state\n        } else {\n            step_change = dynamic_limit; // Cap velocity ceiling to prevent overshooting\n        }\n    }\n    \n    // G. Apply Step Vector directly relative to physical position\n    next_command = current_position + (step_change * pid_sign);\n    pulse_delta = next_command - current_position;\n}\n\n// 6. Hard Structural Boundaries & Safety Guards\n// ---------------------------------------------------------------------\nif (next_command > max_pos_limit) {\n    next_command = max_pos_limit;\n    pulse_delta = next_command - current_position;\n} else if (next_command < min_pos_limit) {\n    next_command = min_pos_limit;\n    pulse_delta = next_command - current_position;\n}"("current_load"=w783, "set_load"=w792, "current_position"=w861, "integral_in"=w891, "prev_error_in"=w890, "kp"=w857, "ki"=w853, "kd"=w849, "deadband_pct"=w845, "pct_scale"=w841, "init_step"=w837, "init_move"=w835, "max_step_limit"=w831, "i_limit"=w827, "min_pos_limit"=w823, "max_pos_limit"=w819, "fine_tune_pct"=5.0 ("input variable"), "min_deadband_floor"=0.05 ("input variable"), "min_finetune_floor"=0.15 ("input variable")) -> ("next_command"=w808:dbl, "integral_out"=w896:dbl, "prev_error_out"=w895:dbl, "pulse_delta"=w812:dbl)
            n627 = Bundle("Value"=w792, "Value"=w783, 0.0) -> (w788:cluster{"Value":dbl, "Value":dbl, dbl})  [unwired: 1 in]
            n628 = Unbundle By Name(w894) -> ("PID.gFF Rot"=w789:refnum<vi>)
            n629 = property class="WFChart (strict)"(reference=w789, "Value"=w788) -> (reference out=w791:refnum<vi>, error out=w790:errorcluster)  [unwired: 1 in]
            n630 = Close Reference(reference=w791, error in (no error)=w790) -> ()  [unwired: 1 out]
            n631 = Unbundle By Name(w894) -> ("Main Screen.Load En"=w885:refnum<vi>)
            n632 = Unbundle By Name(w894) -> ("PID.apply load"=w877:refnum<vi>)
            n633 = Unbundle By Name(w894) -> ("Config Parameters.Heave PID Speed"=w798:refnum<vi>)
            n634 = property class="Bool (strict)"(reference=w885) -> (reference out=w883:refnum<vi>, error out=w884:errorcluster, "Value"=w779:bool)  [unwired: 1 in]
            n635 = property class="Bool (strict)"(reference=w877) -> (reference out=w879:refnum<vi>, error out=w878:errorcluster, "Value"=w875:bool)  [unwired: 1 in]
            n636 = Close Reference(reference=w883, error in (no error)=w884) -> ()  [unwired: 1 out]
            n637 = property class="DigNum (strict)"(reference=w798) -> (reference out=w800:refnum<vi>, error out=w799:errorcluster, "Value"=w797:dbl)  [unwired: 1 in]
            n638 = Close Reference(reference=w879, error in (no error)=w878) -> ()  [unwired: 1 out]
            n639 = Unbundle By Name(w894) -> ("New PID LOGIC.Pulse delta"=w815:refnum<vi>)
            n640 = Unbundle By Name(w894) -> ("Heave AND Surge.Mode Command"=w805:refnum<vi>)
            n641 = Unbundle By Name(w894) -> ("Heave AND Surge.Distance"=w811:refnum<vi>)
            n642 = Close Reference(reference=w800, error in (no error)=w799) -> ()  [unwired: 1 out]
            n643 = Not(x=w779) -> (.not. x?=w876:bool)
            n644 = Not(x=w875) -> (.not. x?=w874:bool)
            n645 = property class="DigNum (strict)"(reference=w815, "Value"=w812) -> (reference out=w813:refnum<vi>, error out=w814:errorcluster)  [unwired: 1 in]
            n646 = property class="DigNum (strict)"(reference=w811, error in=w893, "Value"=w808) -> (reference out=w809:refnum<vi>, error out=w810:errorcluster)
            n647 = Unbundle By Name(w894) -> ("Heave AND Surge.SPEED"=w803:refnum<vi>)
            n648 = property class="DigNum (strict)"(reference=w805, error in=w893, "Value"=u8 4) -> (reference out=w807:refnum<vi>, error out=w806:errorcluster)
            n649 = And(x=w876, y=w874) -> ()  [unwired: 1 out]
            n650 = property class="DigNum (strict)"(reference=w803, "Value"=w797) -> (reference out=w801:refnum<vi>, error out=w802:errorcluster)  [unwired: 1 in]
            n651 = Close Reference(reference=w813, error in (no error)=w814) -> ()  [unwired: 1 out]
            n652 = Close Reference(reference=w809, error in (no error)=w810) -> (error out=w794:errorcluster)
            n653 = Close Reference(reference=w807, error in (no error)=w806) -> (error out=w796:errorcluster)
            n654 = Merge Errors(w794, w796) -> (w795:errorcluster)
            n655 = Close Reference(reference=w801, error in (no error)=w802) -> ()  [unwired: 1 out]
            n656 = call "HEAVE WRITE FGV.vi"("Enum - Menu"=Heave_Write_enum."WRITE", "error in (no error)"=w795, "main ref"=w894) -> ("error out"=w892:errorcluster)  [unwired: 8 in]
          }
        }
        n657 = Unbundle By Name(w760) -> ("Main Home Screen.EXIT"=w772:refnum<vi>)
        n658 = property class="Bool (strict)"(reference=w772) -> (reference out=w769:refnum<vi>, error out=w770:errorcluster, "Value"=w768:bool)  [unwired: 1 in]
        n659 = case shown="False" w768 {
          tunnel: [w903 w907] -> w774
          tunnel: w773 -> [w902 w906]
          tunnel: w767 -> [w901 w905]
          frame True {
            n660 = call-poly "Enqueue Message.vi"("error in (no error)"=w901, "Message"="Confirm Quit", "Message Queue"=w902) -> ("error out"=w903:errorcluster)  [unwired: 7 in, 1 out]
          }
          frame False {
            n661 = call-poly "Enqueue Message.vi"("error in (no error)"=w905, "Message"="Load Pid Main", "Message Queue"=w906) -> ("error out"=w907:errorcluster)  [unwired: 7 in, 1 out]
          }
        }
        n662 = Close Reference(reference=w769, error in (no error)=w770) -> ()  [unwired: 1 out]
      }
      frame "Error" {
        w909 = 0.0 ("integral_out")
        # "#CodeRecommended - If you ever change the name of this \"Error\" message, you'll need to update the name in the Check Loop Error.vi as well."
        # "#CodeRecommended - Consider creating a system for logging errors in some way. These errors are for notification purposes only. Handling of specific errors should be performed in the message frames that generated the error."
        # "Error - Display an error dialog. This message is sent by the \"Error Handler\" VIs at the end of other loops in this application."
        n663 = Variant To Data(error in=w916, type=errorcluster {"status"=FALSE, "code"=0, "source"=""} ("error constant"), Variant=w914) -> (data=w912:errorcluster, error out=w911:errorcluster)
        n664 = call <vilib>:"Simple Error Handler.vi"("error in (no error)"=w912) -> ()  [unwired: 4 in, 5 out]
        n665 = Merge Errors(w911) -> (w910:errorcluster)
      }
      frame "Confirm Quit" {
        w917 = 0.0 ("integral_out")
        # "#CodeNeeded - If you want to provide an \"Are you sure\" dialog (or some other notification) before the application exits, place that code here. This message is typically sent from a Panel Close? event."
        # "Confirm Quit - Message that can confirm whether or not the user wants to exit the application."
        n666 = call-poly "Enqueue Message.vi"("Priority Message? (F)"=TRUE, "error in (no error)"=w924, "Message"="Exit", "Message Queue"=w920) -> ("error out"=w921:errorcluster)  [unwired: 6 in, 1 out]
        n667 = Merge Errors(w921) -> (w922:errorcluster)
      }
      frame "Exit" {
        w925 = 0.0 ("integral_out")
        # "Stop the VI"
        # "Release the message queue reference"
        # "#CodeNeeded - Add any required cleanup code here. Note that if 'Exit' was called as a result of an error, an error dialog will be displayed. Add any custom error handling for an 'Exit' condition here as well."
        # "Exit - Exit the application."
        n668 = call "Fire User Event - Stop.vi"("User Event - Stop"=w926) -> ("error out"=w928:errorcluster)  [unwired: 10 in]
        n669 = Release Queue(queue=w933, error in (no error)=w927) -> (error out=w930:errorcluster)  [unwired: 1 in, 2 out]
        n670 = Merge Errors(w928, w930) -> (w929:errorcluster)
      }
      frame Default {
        w934 = 0.0 ("integral_out")
        # "'Default' case only runs if there is a message that isn't defined in any of the other cases.  Output a programming error."
        n671 = xnode "Error Ring"("parameter 0"=w935) -> ("error out"=w936:errorcluster)
      }
    }
    n672 = call "LAB-IQ Error Handler - Message Handling Loop.vi"("error in (no error)"=w738, "Message Queue"=w740) -> ("dup error in"=w739:errorcluster)  [unwired: 8 in, 1 out]
  }
  n673 = Obtain Queue(max queue size (-1, unlimited)=w15, name (unnamed)=w8, element data type=w8, error in (no error)=w14) -> (queue out=w16:refnum<queue>, error out=w9:errorcluster)  [unwired: 1 in, 1 out]
  n674 = call "HEAVE WRITE FGV.vi"("Enum - Menu"=Heave_Write_enum."INIT", "error in (no error)"=w9, "main ref"=w7) -> ("error out"=w13:errorcluster)  [unwired: 8 in]
  n675 = call "Stall Data Flow.vim"("value in"=w13, "milliseconds to wait"=u32 1000) -> ("value out"=w11:errorcluster)  [unwired: 1 out]
  n676 = UDP Open(8:w11, 9:-1 ("timeout ms (25000)"), 10:"192.168.1.10" ("service name"), 11:u16 8889 ("port")) -> (port=w5:refnum<k16>, 0:w6:errorcluster)  [unwired: 1 in, 1 out]
  n677 = disable-structure shown="Disabled" {
    disable-tunnel: [w949 _] -> w32
    disable-tunnel: w7 -> [w948 _]
    disable-tunnel: w26 -> [w947 _]
    disable-tunnel: w18 -> [w946 _]
    disable-tunnel: w14 -> [w945 _]
    frame Disabled {
      n678 = while {
        shift-right: [w960] -> _
        shift-left: w948 -> [w961]
        tunnel: [w954] -> w949
        tunnel: w946 -> [w952]
        tunnel: w945 -> [w951]
        tunnel: w947 -> [w950]
        stop <- w959 stop-if-true
        # "Heave Motor  Handling Loop"
        n679 = call "Dequeue Message.vi"("error in (no error)"=w951, "Message Queue"=w952) -> ("error out"=w958:errorcluster, "Message Data"=w956:variant, "Message"=w957:string, "dup Message Queue"=w955:refnum<queue>)  [unwired: 6 in]
        n680 = case "Message Cases" shown="\"init\"" w957 {
          selector: w957 -> [_ _ _ _ _ w1041]
          tunnel: w955 -> [w971 w998 _ w1029 w1040 _]
          tunnel: w958 -> [w964 w996 w1019 w1032 w1034 _]
          tunnel: [w965 w999 w1013 w1020 w1036 w1042] -> w953
          tunnel: w961 -> [w962 w988 w1018 w1023 w1039 w1043]
          tunnel: [w962 w988 w1018 w1023 w1039 w1043] -> w960
          tunnel: [_ _ _ _ TRUE _] -> w959
          tunnel: w956 -> [_ _ w1017 _ _ _]
          tunnel: w950 -> [_ _ _ _ w1033 _]
          frame "init" {
            # "Initialize - All initialization work should take place in this message, since other loops can potentially enqueue messages that execute immediately after this one."
            n681 = call "HEAVE WRITE FGV.vi"("Enum - Menu"=Heave_Write_enum."INIT", "error in (no error)"=w964, "main ref"=w962) -> ("error out"=w970:errorcluster)  [unwired: 8 in]
            n682 = call "Stall Data Flow.vim"("value in"=w970, "milliseconds to wait"=u32 1000) -> ("value out"=w968:errorcluster)  [unwired: 1 out]
            n683 = disable-structure shown="Enabled" {
              disable-tunnel: w968 -> [w984 w985]
              disable-tunnel: [w983 w985] -> w963
              disable-tunnel: w962 -> [w982 _]
              frame Disabled {
                n684 = call "Heave Init.vi"("error in (no error)"=w984, "main ref"=w982) -> ("error out"=w983:errorcluster)  [unwired: 9 in]
              }
              frame Enabled {
              }
            }
            n685 = disable-structure shown="Enabled" {
              disable-tunnel: [w975 w978] -> w966
              disable-tunnel: w963 -> [w974 w977]
              disable-tunnel: w962 -> [w973 _]
              frame Disabled {
                n686 = call "HEAVE READ FGV.vi"("Enum - Menu"=Heave_Right_enum."INIT", "error in (no error)"=w974, "main ref"=w973) -> ("error out"=w975:errorcluster)  [unwired: 7 in, 1 out]
              }
              frame Enabled {
                n687 = UDP Open(8:w977, 9:-1 ("timeout ms (25000)"), 10:"192.168.1.10" ("service name"), 11:u16 8889 ("port")) -> (0:w978:errorcluster)  [unwired: 1 in, 2 out]
              }
            }
            n688 = call-poly "Enqueue Message.vi"("error in (no error)"=w966, "Message"="Heave Main", "Message Queue"=w971) -> ("error out"=w965:errorcluster)  [unwired: 7 in, 1 out]
          }
          frame "Heave Main" {
            n689 = Unbundle By Name(w988) -> ("Heave AND Surge.Read Heave Temp"=w991:refnum<vi>)
            n690 = property class="Bool (strict)"(reference=w991) -> (reference out=w989:refnum<vi>, error out=w990:errorcluster, "Value"=w987:bool)  [unwired: 1 in]
            n691 = Close Reference(reference=w989, error in (no error)=w990) -> ()  [unwired: 1 out]
            n692 = case shown="True" w987 {
              tunnel: w996 -> [w1000 w1004]
              tunnel: [w1000 w1003] -> w992
              tunnel: w988 -> [_ w1002]
              frame False {
              }
              frame True {
                n693 = call "HEAVE READ FGV.vi"("Enum - Menu"=Heave_Right_enum."READ", "error in (no error)"=w1004, "main ref"=w1002) -> ("error out"=w1003:errorcluster)  [unwired: 7 in, 1 out]
              }
            }
            n694 = Unbundle By Name(w988) -> ("Main Home Screen.EXIT"=w997:refnum<vi>)
            n695 = property class="Bool (strict)"(reference=w997) -> (reference out=w994:refnum<vi>, error out=w995:errorcluster, "Value"=w993:bool)  [unwired: 1 in]
            n696 = call <vilib>:"Clear Errors.vi"("error in (no error)"=w992) -> ("error out"=w986:errorcluster)  [unwired: 5 in, 1 out]
            n697 = Close Reference(reference=w994, error in (no error)=w995) -> ()  [unwired: 1 out]
            n698 = case shown="False" w993 {
              tunnel: [w1007 w1011] -> w999
              tunnel: w998 -> [w1006 w1010]
              tunnel: w986 -> [w1005 w1009]
              frame True {
                n699 = call-poly "Enqueue Message.vi"("error in (no error)"=w1005, "Message"="Confirm Quit", "Message Queue"=w1006) -> ("error out"=w1007:errorcluster)  [unwired: 7 in, 1 out]
              }
              frame False {
                n700 = call-poly "Enqueue Message.vi"("error in (no error)"=w1009, "Message"="Heave Main", "Message Queue"=w1010) -> ("error out"=w1011:errorcluster)  [unwired: 7 in, 1 out]
              }
            }
          }
          frame "Error" {
            # "#CodeRecommended - If you ever change the name of this \"Error\" message, you'll need to update the name in the Check Loop Error.vi as well."
            # "#CodeRecommended - Consider creating a system for logging errors in some way. These errors are for notification purposes only. Handling of specific errors should be performed in the message frames that generated the error."
            # "Error - Display an error dialog. This message is sent by the \"Error Handler\" VIs at the end of other loops in this application."
            n701 = Variant To Data(error in=w1019, type=errorcluster {"status"=FALSE, "code"=0, "source"=""} ("error constant"), Variant=w1017) -> (data=w1015:errorcluster, error out=w1014:errorcluster)
            n702 = call <vilib>:"Simple Error Handler.vi"("error in (no error)"=w1015) -> ()  [unwired: 4 in, 5 out]
            n703 = Merge Errors(w1014) -> (w1013:errorcluster)
          }
          frame "Confirm Quit" {
            # "#CodeNeeded - If you want to provide an \"Are you sure\" dialog (or some other notification) before the application exits, place that code here. This message is typically sent from a Panel Close? event."
            # "Confirm Quit - Message that can confirm whether or not the user wants to exit the application."
            n704 = call-poly "Enqueue Message.vi"("Priority Message? (F)"=TRUE, "error in (no error)"=w1032, "Message"="Exit", "Message Queue"=w1029) -> ("error out"=w1030:errorcluster)  [unwired: 6 in, 1 out]
            n705 = Merge Errors(w1030) -> (w1031:errorcluster)
            n706 = call "HEAVE READ FGV.vi"("Enum - Menu"=Heave_Right_enum."CLOSE", "error in (no error)"=w1031, "main ref"=w1023) -> ("error out"=w1026:errorcluster)  [unwired: 7 in, 1 out]
            n707 = call <vilib>:"Clear Errors.vi"("error in (no error)"=w1026) -> ("error out"=w1021:errorcluster)  [unwired: 5 in, 1 out]
            n708 = call "HEAVE WRITE FGV.vi"("Enum - Menu"=Heave_Write_enum."CLOSE", "error in (no error)"=w1021, "main ref"=w1023) -> ("error out"=w1024:errorcluster)  [unwired: 8 in]
            n709 = call <vilib>:"Clear Errors.vi"("error in (no error)"=w1024) -> ("error out"=w1020:errorcluster)  [unwired: 5 in, 1 out]
          }
          frame "Exit" {
            # "Stop the VI"
            # "Release the message queue reference"
            # "#CodeNeeded - Add any required cleanup code here. Note that if 'Exit' was called as a result of an error, an error dialog will be displayed. Add any custom error handling for an 'Exit' condition here as well."
            # "Exit - Exit the application."
            n710 = call "Fire User Event - Stop.vi"("User Event - Stop"=w1033) -> ("error out"=w1035:errorcluster)  [unwired: 10 in]
            n711 = Release Queue(queue=w1040, error in (no error)=w1034) -> (error out=w1037:errorcluster)  [unwired: 1 in, 2 out]
            n712 = Merge Errors(w1035, w1037) -> (w1036:errorcluster)
          }
          frame Default {
            # "'Default' case only runs if there is a message that isn't defined in any of the other cases.  Output a programming error."
            n713 = xnode "Error Ring"("parameter 0"=w1041) -> ("error out"=w1042:errorcluster)
          }
        }
        n714 = call "LAB-IQ Error Handler - Message Handling Loop.vi"("error in (no error)"=w953, "Message Queue"=w955) -> ("dup error in"=w954:errorcluster)  [unwired: 8 in, 1 out]
      }
    }
    frame Enabled {
    }
  }
  n715 = while {
    tunnel: w64 -> [w1065]
    shift-right: [w1072] -> _
    shift-left: w7 -> [w1073]
    tunnel: w26 -> [w1070]
    tunnel: w57 -> [w1069]
    tunnel: [w1063] -> w65
    tunnel: w36 -> [w1061]
    tunnel: w35 -> [w1060]
    tunnel: w18 -> [w1059]
    tunnel: w33 -> [w1058]
    tunnel: w30 -> [w1057]
    tunnel: w29 -> [w1056]
    tunnel: w28 -> [w1055]
    tunnel: w27 -> [w1054]
    tunnel: w25 -> [w1053]
    tunnel: w24 -> [w1052]
    tunnel: w23 -> [w1051]
    stop <- w1071 stop-if-true
    # "Message Handling Loop"
    n716 = call "Dequeue Message.vi"("error in (no error)"=w1069, "Message Queue"=w1065) -> ("error out"=w1068:errorcluster, "Message Data"=w1066:variant, "Message"=w1067:string, "dup Message Queue"=w1064:refnum<queue>)  [unwired: 6 in]
    n717 = case "Message Cases" shown="\"init\"" w1067 {
      selector: w1067 -> [_ _ _ _ _ _ _ _ _ _ _ _ _ _ _ _ _ _ _ _ _ _ _ _ _ _ _ _ _ _ _ _ _ _ _ _ _ _ _ _ w2001]
      tunnel: w1064 -> [_ w1103 _ _ _ _ _ _ _ _ _ _ _ _ _ _ _ _ _ _ _ _ _ _ _ _ _ _ _ _ _ _ _ _ _ _ _ _ w1989 w2000 _]
      tunnel: w1068 -> [w1075 w1105 w1119 w1148 w1169 w1186 w1203 w1220 w1241 w1253 w1303 w1308 w1315 w1320 w1385 w1411 w1437 w1468 w1480 w1528 w1548 w1637 w1714 w1753 w1765 w1786 w1815 w1834 w1845 w1856 w1867 w1877 w1889 w1911 w1951 w1966 w1974 w1981 w1992 w1993 _]
      tunnel: [w1076 w1102 w1118 w1149 w1164 w1181 w1198 w1215 w1236 w1245 w1281 w1306 w1313 w1324 w1381 w1407 w1433 w1469 w1481 w1492 w1539 w1628 w1713 w1752 w1764 w1785 w1802 w1836 w1847 w1858 w1869 w1879 w1888 w1910 w1949 w1964 w1972 w1975 w1984 w1996 w2002] -> w1062
      tunnel: w1073 -> [w1074 w1077 w1120 w1147 w1155 w1172 w1189 w1206 w1224 w1243 w1258 w1305 w1311 w1319 w1383 w1409 w1435 w1459 w1471 w1483 w1532 w1620 w1708 w1751 w1763 w1779 w1797 w1832 w1843 w1854 w1865 w1876 w1887 w1909 w1930 w1955 w1967 w1980 w1982 w1999 w2003]
      tunnel: [w1074 w1077 w1120 w1147 w1155 w1172 w1189 w1206 w1224 w1243 w1258 w1305 w1311 w1319 w1383 w1409 w1435 w1459 w1471 w1483 w1532 w1620 w1708 w1751 w1763 w1779 w1797 w1832 w1843 w1854 w1865 w1876 w1887 w1909 w1930 w1955 w1967 w1980 w1982 w1999 w2003] -> w1072
      tunnel: [_ _ _ _ _ _ _ _ _ _ _ _ _ _ _ _ _ _ _ _ _ _ _ _ _ _ _ _ _ _ _ _ _ _ _ _ _ _ _ TRUE _] -> w1071
      tunnel: w1066 -> [_ _ _ _ _ _ _ _ _ _ _ _ _ _ _ _ _ _ _ _ _ _ _ _ _ _ _ _ _ _ _ _ _ _ _ _ _ w1979 _ _ _]
      tunnel: w1070 -> [_ _ _ _ _ _ _ _ _ _ _ _ _ _ _ _ _ _ _ _ _ _ _ _ _ _ _ _ _ _ _ _ _ _ _ _ _ _ _ w1995 _]
      tunnel: w1061 -> [_ _ w1117 _ _ _ _ _ _ _ _ _ _ _ _ _ _ _ _ _ _ _ _ _ _ _ _ _ _ _ _ _ _ _ _ _ _ _ _ _ _]
      tunnel: w1060 -> [_ _ w1116 _ _ _ _ _ _ _ _ _ _ _ _ _ _ _ _ _ _ _ _ _ _ _ _ _ _ _ _ _ _ _ _ _ _ _ _ _ _]
      tunnel: w1059 -> [_ _ w1115 _ _ _ _ _ _ _ _ _ _ _ _ _ _ _ _ _ _ _ _ _ _ _ _ _ _ _ _ _ _ _ _ _ _ _ _ _ _]
      tunnel: w1058 -> [_ _ w1114 _ _ _ _ _ _ _ _ _ _ _ _ _ _ _ _ _ _ _ _ _ _ _ _ _ _ _ _ _ _ _ _ _ _ _ _ _ _]
      tunnel: w1057 -> [_ _ w1113 _ _ _ _ _ _ _ _ _ _ _ _ _ _ _ _ _ _ _ _ _ _ _ _ _ _ _ _ _ _ _ _ _ _ _ _ _ _]
      tunnel: w1056 -> [_ _ w1112 _ _ _ _ _ _ _ _ _ _ _ _ _ _ _ _ _ _ _ _ _ _ _ _ _ _ _ _ _ _ _ _ _ _ _ _ _ _]
      tunnel: w1055 -> [_ _ w1111 _ _ _ _ _ _ _ _ _ _ _ _ _ _ _ _ _ _ _ _ _ _ _ _ _ _ _ _ _ _ _ _ _ _ _ _ _ _]
      tunnel: w1054 -> [_ _ w1110 _ _ _ _ _ _ _ _ _ _ _ _ _ _ _ _ _ _ _ _ _ _ _ _ _ _ _ _ _ _ _ _ _ _ _ _ _ _]
      tunnel: w1053 -> [_ _ w1109 _ _ _ _ _ _ _ _ _ _ _ _ _ _ _ _ _ _ _ _ _ _ _ _ _ _ _ _ _ _ _ _ _ _ _ _ _ _]
      tunnel: w1052 -> [_ _ w1108 _ _ _ _ _ _ _ _ _ _ _ _ _ _ _ _ _ _ _ _ _ _ _ _ _ _ _ _ _ _ _ _ _ _ _ _ _ _]
      tunnel: w1051 -> [_ _ w1107 _ _ _ _ _ _ _ _ _ _ _ _ _ _ _ _ _ _ _ _ _ _ _ _ _ _ _ _ _ _ _ _ _ _ _ _ _ _]
      frame "Time Out" {
        n718 = call "Pulse_mm conversion loop.vi"("error in (no error)"=w1075, "main ref"=w1074) -> ("error out"=w1076:errorcluster)  [unwired: 9 in]
        n719 = call "Load Commiunication Error.vi"("error in (no error)"=w1075, "main ref"=w1074) -> ()  [unwired: 9 in, 1 out]
      }
      frame "init" {
        # "Initialize - All initialization work should take place in this message, since other loops can potentially enqueue messages that execute immediately after this one."
        n720 = call-poly "Enqueue Message.vi"("error in (no error)"=w1105, "Message"="Init Other Loop", "Message Queue"=w1103) -> ("error out"=w1106:errorcluster)  [unwired: 7 in, 1 out]
        n721 = Unbundle By Name(w1077) -> ("Loading.Communication is established"=w1078:refnum<vi>)
        n722 = Unbundle By Name(w1077) -> ("Loading Com Port.Load Cell Temp"=w1097:refnum<vi>)
        n723 = Unbundle By Name(w1077) -> ("Loading.SSP 0.3"=w1091:refnum<vi>)
        n724 = Unbundle By Name(w1077) -> ("Loading.SSP 0.5"=w1088:refnum<vi>)
        n725 = Unbundle By Name(w1077) -> ("Loading.SSP 0.75"=w1083:refnum<vi>)
        n726 = call "Read Config Unitest.vi"("error in (no error)"=w1106, "main ref"=w1077) -> ("error out"=w1101:errorcluster)  [unwired: 9 in]
        n727 = call "Encrypt file path creation.vi"("error in (no error)"=w1101) -> ("error out"=w1100:errorcluster, "File Path"=w1099:path)  [unwired: 9 in]
        n728 = property class="Bool (strict)"(reference=w1097, "Value"=FALSE) -> (reference out=w1095:refnum<vi>, error out=w1096:errorcluster)  [unwired: 1 in]
        n729 = property class="Bool (strict)"(reference=w1088, "Visible"=FALSE) -> (reference out=w1086:refnum<vi>, error out=w1087:errorcluster)  [unwired: 1 in]
        n730 = property class="Bool (strict)"(reference=w1091, "Visible"=FALSE) -> (reference out=w1093:refnum<vi>, error out=w1092:errorcluster)  [unwired: 1 in]
        n731 = property class="Bool (strict)"(reference=w1083, "Visible"=FALSE) -> (reference out=w1085:refnum<vi>, error out=w1084:errorcluster)  [unwired: 1 in]
        n732 = property class="Bool (strict)"(reference=w1078, "Visible"=FALSE ("Value")) -> (reference out=w1080:refnum<vi>, error out=w1079:errorcluster)  [unwired: 1 in]
        n733 = call "DATA ENCRYPT STRING FILE WRITE.vi"("file path (dialog if empty)"=w1099, "error in (no error)"=w1100, "User Action"="System Booted", "main ref"=w1077) -> ("error out"=w1102:errorcluster)  [unwired: 5 in, 1 out]
        n734 = Close Reference(reference=w1086, error in (no error)=w1087) -> ()  [unwired: 1 out]
        n735 = Close Reference(reference=w1093, error in (no error)=w1092) -> ()  [unwired: 1 out]
        n736 = Close Reference(reference=w1085, error in (no error)=w1084) -> ()  [unwired: 1 out]
        n737 = Close Reference(reference=w1095, error in (no error)=w1096) -> ()  [unwired: 1 out]
        n738 = Close Reference(reference=w1080, error in (no error)=w1079) -> ()  [unwired: 1 out]
      }
      frame "Init Other Loop" {
        n739 = disable-structure shown="Disabled" {
          disable-tunnel: w1119 -> [w1144 w1145]
          disable-tunnel: [w1133 w1145] -> w1118
          disable-tunnel: w1117 -> [w1131 _]
          disable-tunnel: w1116 -> [w1130 _]
          disable-tunnel: w1115 -> [w1129 _]
          disable-tunnel: w1114 -> [w1128 _]
          disable-tunnel: w1113 -> [w1127 _]
          disable-tunnel: w1112 -> [w1126 _]
          disable-tunnel: w1111 -> [w1125 _]
          disable-tunnel: w1110 -> [w1124 _]
          disable-tunnel: w1109 -> [w1123 _]
          disable-tunnel: w1108 -> [w1122 _]
          disable-tunnel: w1107 -> [w1121 _]
          frame Disabled {
            w1132 = "Init" ("Message")
            n740 = call-poly "Enqueue Message.vi"("error in (no error)"=w1144, "Message"=w1132, "Message Queue"=w1131) -> ("error out"=w1143:errorcluster)  [unwired: 7 in, 1 out]
            n741 = call-poly "Enqueue Message.vi"("error in (no error)"=w1143, "Message"=w1132, "Message Queue"=w1130) -> ("error out"=w1142:errorcluster)  [unwired: 7 in, 1 out]
            n742 = call-poly "Enqueue Message.vi"("error in (no error)"=w1142, "Message"=w1132, "Message Queue"=w1129) -> ("error out"=w1141:errorcluster)  [unwired: 7 in, 1 out]
            n743 = call-poly "Enqueue Message.vi"("error in (no error)"=w1141, "Message"=w1132, "Message Queue"=w1128) -> ("error out"=w1140:errorcluster)  [unwired: 7 in, 1 out]
            n744 = call-poly "Enqueue Message.vi"("error in (no error)"=w1140, "Message"=w1132, "Message Queue"=w1127) -> ("error out"=w1139:errorcluster)  [unwired: 7 in, 1 out]
            n745 = call-poly "Enqueue Message.vi"("error in (no error)"=w1139, "Message"=w1132, "Message Queue"=w1126) -> ("error out"=w1138:errorcluster)  [unwired: 7 in, 1 out]
            n746 = call-poly "Enqueue Message.vi"("error in (no error)"=w1138, "Message"=w1132, "Message Queue"=w1125) -> ("error out"=w1137:errorcluster)  [unwired: 7 in, 1 out]
            n747 = call-poly "Enqueue Message.vi"("error in (no error)"=w1137, "Message"=w1132, "Message Queue"=w1124) -> ("error out"=w1136:errorcluster)  [unwired: 7 in, 1 out]
            n748 = call-poly "Enqueue Message.vi"("error in (no error)"=w1136, "Message"=w1132, "Message Queue"=w1123) -> ("error out"=w1135:errorcluster)  [unwired: 7 in, 1 out]
            n749 = call-poly "Enqueue Message.vi"("error in (no error)"=w1135, "Message"=w1132, "Message Queue"=w1122) -> ("error out"=w1134:errorcluster)  [unwired: 7 in, 1 out]
            n750 = call-poly "Enqueue Message.vi"("error in (no error)"=w1134, "Message"=w1132, "Message Queue"=w1121) -> ("error out"=w1133:errorcluster)  [unwired: 7 in, 1 out]
          }
          frame Enabled {
          }
        }
      }
      frame "Service Save" {
        n751 = call "Write Config Unitest.vi"("error in (no error)"=w1148, "main ref"=w1147) -> ("error out"=w1153:errorcluster)  [unwired: 9 in]
        n752 = call "Stall Data Flow.vim"("value in"=w1153, "milliseconds to wait"=u32 2000) -> ("value out"=w1152:errorcluster)  [unwired: 1 out]
        n753 = call "Read Config Unitest.vi"("error in (no error)"=w1152, "main ref"=w1147) -> ("error out"=w1150:errorcluster)  [unwired: 9 in]
        n754 = call "DATA ENCRYPT STRING FILE WRITE.vi"("error in (no error)"=w1150, "User Action"="Service Parameter Saved", "main ref"=w1147) -> ("error out"=w1149:errorcluster)  [unwired: 6 in, 1 out]
      }
      frame "HOME" {
        n755 = call "DATA ENCRYPT STRING FILE WRITE.vi"("error in (no error)"=w1169, "User Action"="User Pressed Home", "main ref"=w1155) -> ("error out"=w1165:errorcluster)  [unwired: 6 in, 1 out]
        n756 = Unbundle By Name(w1155) -> ("Main Home Screen.MainPage"=w1160:refnum<vi>)
        n757 = Unbundle By Name(w1155) -> ("Main Home Screen.Home"=w1168:refnum<vi>)
        n758 = Unbundle By Name(w1155) -> ("Main Home Screen.GUI"=w1158:refnum<vi>)
        n759 = property class="Bool (strict)"(reference=w1168, error in=w1165, "Value"=FALSE) -> (reference out=w1166:refnum<vi>, error out=w1167:errorcluster)
        n760 = property class="TabCtl (strict)"(reference=w1160, "Value"=T5."HOME") -> (reference out=w1162:refnum<vi>, error out=w1161:errorcluster)  [unwired: 1 in]
        n761 = property class="TabCtl (strict)"(reference=w1158, "Value"=T4."Setup") -> (reference out=w1156:refnum<vi>, error out=w1157:errorcluster)  [unwired: 1 in]
        n762 = Close Reference(reference=w1166, error in (no error)=w1167) -> (error out=w1164:errorcluster)
        n763 = Close Reference(reference=w1162, error in (no error)=w1161) -> ()  [unwired: 1 out]
        n764 = Close Reference(reference=w1156, error in (no error)=w1157) -> ()  [unwired: 1 out]
      }
      frame "Platform Setting" {
        n765 = call "DATA ENCRYPT STRING FILE WRITE.vi"("error in (no error)"=w1186, "User Action"="User Pressed Platform Setting", "main ref"=w1172) -> ("error out"=w1182:errorcluster)  [unwired: 6 in, 1 out]
        n766 = Unbundle By Name(w1172) -> ("Main Home Screen.Platform Settings"=w1185:refnum<vi>)
        n767 = Unbundle By Name(w1172) -> ("Main Home Screen.MainPage"=w1177:refnum<vi>)
        n768 = Unbundle By Name(w1172) -> ("Main Home Screen.GUI"=w1175:refnum<vi>)
        n769 = property class="TabCtl (strict)"(reference=w1177, "Value"=T5."PlatformSetting") -> (reference out=w1179:refnum<vi>, error out=w1178:errorcluster)  [unwired: 1 in]
        n770 = property class="TabCtl (strict)"(reference=w1175, "Value"=T4."Setup") -> (reference out=w1173:refnum<vi>, error out=w1174:errorcluster)  [unwired: 1 in]
        n771 = property class="Bool (strict)"(reference=w1185, error in=w1182, "Value"=FALSE) -> (reference out=w1183:refnum<vi>, error out=w1184:errorcluster)
        n772 = Close Reference(reference=w1179, error in (no error)=w1178) -> ()  [unwired: 1 out]
        n773 = Close Reference(reference=w1173, error in (no error)=w1174) -> ()  [unwired: 1 out]
        n774 = Close Reference(reference=w1183, error in (no error)=w1184) -> (error out=w1181:errorcluster)
      }
      frame "Configure" {
        n775 = call "DATA ENCRYPT STRING FILE WRITE.vi"("error in (no error)"=w1203, "User Action"="User Pressed Configure", "main ref"=w1189) -> ("error out"=w1199:errorcluster)  [unwired: 6 in, 1 out]
        n776 = Unbundle By Name(w1189) -> ("Main Home Screen.Configure"=w1202:refnum<vi>)
        n777 = Unbundle By Name(w1189) -> ("Main Home Screen.MainPage"=w1194:refnum<vi>)
        n778 = Unbundle By Name(w1189) -> ("Main Home Screen.GUI"=w1192:refnum<vi>)
        n779 = property class="Bool (strict)"(reference=w1202, error in=w1199, "Value"=FALSE) -> (reference out=w1200:refnum<vi>, error out=w1201:errorcluster)
        n780 = property class="TabCtl (strict)"(reference=w1194, "Value"=T5."Details") -> (reference out=w1196:refnum<vi>, error out=w1195:errorcluster)  [unwired: 1 in]
        n781 = property class="TabCtl (strict)"(reference=w1192, "Value"=T4."Setup") -> (reference out=w1190:refnum<vi>, error out=w1191:errorcluster)  [unwired: 1 in]
        n782 = Close Reference(reference=w1200, error in (no error)=w1201) -> (error out=w1198:errorcluster)
        n783 = Close Reference(reference=w1196, error in (no error)=w1195) -> ()  [unwired: 1 out]
        n784 = Close Reference(reference=w1190, error in (no error)=w1191) -> ()  [unwired: 1 out]
      }
      frame "Analysis" {
        n785 = call "DATA ENCRYPT STRING FILE WRITE.vi"("error in (no error)"=w1220, "User Action"="User Pressed Analysis", "main ref"=w1206) -> ("error out"=w1216:errorcluster)  [unwired: 6 in, 1 out]
        n786 = Unbundle By Name(w1206) -> ("Main Home Screen.MainPage"=w1211:refnum<vi>)
        n787 = Unbundle By Name(w1206) -> ("Main Home Screen.Analysis"=w1219:refnum<vi>)
        n788 = Unbundle By Name(w1206) -> ("Main Home Screen.GUI"=w1209:refnum<vi>)
        n789 = property class="Bool (strict)"(reference=w1219, error in=w1216, "Value"=FALSE) -> (reference out=w1217:refnum<vi>, error out=w1218:errorcluster)
        n790 = property class="TabCtl (strict)"(reference=w1211, "Value"=T5."Analysis") -> (reference out=w1213:refnum<vi>, error out=w1212:errorcluster)  [unwired: 1 in]
        n791 = property class="TabCtl (strict)"(reference=w1209, "Value"=T4."Setup") -> (reference out=w1207:refnum<vi>, error out=w1208:errorcluster)  [unwired: 1 in]
        n792 = Close Reference(reference=w1217, error in (no error)=w1218) -> (error out=w1215:errorcluster)
        n793 = Close Reference(reference=w1213, error in (no error)=w1212) -> ()  [unwired: 1 out]
        n794 = Close Reference(reference=w1207, error in (no error)=w1208) -> ()  [unwired: 1 out]
      }
      frame "service 2" {
        n795 = call "DATA ENCRYPT STRING FILE WRITE.vi"("error in (no error)"=w1241, "User Action"="User Pressed service", "main ref"=w1224) -> ("error out"=w1237:errorcluster)  [unwired: 6 in, 1 out]
        n796 = Unbundle By Name(w1224) -> ("Main Screen.Main Screen Tab"=w1225:refnum<vi>)
        n797 = Unbundle By Name(w1224) -> ("Main Home Screen.MainPage"=w1232:refnum<vi>)
        n798 = Unbundle By Name(w1224) -> ("Main Home Screen.Analysis"=w1240:refnum<vi>)
        n799 = Unbundle By Name(w1224) -> ("Main Home Screen.GUI"=w1230:refnum<vi>)
        n800 = property class="Bool (strict)"(reference=w1240, error in=w1237, "Value"=FALSE) -> (reference out=w1238:refnum<vi>, error out=w1239:errorcluster)
        n801 = property class="TabCtl (strict)"(reference=w1232, "Value"=T5."HOME") -> (reference out=w1234:refnum<vi>, error out=w1233:errorcluster)  [unwired: 1 in]
        n802 = property class="TabCtl (strict)"(reference=w1230, "Value"=T4."Begin") -> (reference out=w1228:refnum<vi>, error out=w1229:errorcluster)  [unwired: 1 in]
        n803 = property class="TabCtl (strict)"(reference=w1225, "Value"=T8."About") -> (reference out=w1222:refnum<vi>, error out=w1226:errorcluster)  [unwired: 1 in]
        n804 = Close Reference(reference=w1238, error in (no error)=w1239) -> (error out=w1236:errorcluster)
        n805 = Close Reference(reference=w1234, error in (no error)=w1233) -> ()  [unwired: 1 out]
        n806 = Close Reference(reference=w1228, error in (no error)=w1229) -> ()  [unwired: 1 out]
        n807 = Close Reference(reference=w1222, error in (no error)=w1226) -> ()  [unwired: 1 out]
      }
      frame "Auto" {
        n808 = call "DATA ENCRYPT STRING FILE WRITE.vi"("error in (no error)"=w1253, "User Action"="User Pressed Auto File Name", "main ref"=w1243) -> ("error out"=w1250:errorcluster)  [unwired: 6 in, 1 out]
        n809 = Get Date/Time In Seconds() -> (seconds since 1Jan1904=w1251:timestamp)
        n810 = Format Into String(format string="%<%I_%M_%S_%p_%d_%B_%Y>T", error in=w1250, w1251) -> (resulting string=w1244:string, error out=w1246:errorcluster)  [unwired: 1 in]
        n811 = Unbundle By Name(w1243) -> ("Config Screen.FILE"=w1249:refnum<vi>)
        n812 = property class="Str"(reference=w1249, error in=w1246, "Value"=w1244) -> (reference out=w1247:refnum<vi>, error out=w1248:errorcluster)
        n813 = Close Reference(reference=w1247, error in (no error)=w1248) -> (error out=w1245:errorcluster)
      }
      frame "Select Load Head" {
        n814 = Unbundle By Name(w1258) -> ("Loading.Enter the Loading Rate (N/min)"=w1279:refnum<vi>)
        n815 = Unbundle By Name(w1258) -> ("Loading.Communication is established"=w1264:refnum<vi>)
        n816 = call "DATA ENCRYPT STRING FILE WRITE.vi"("error in (no error)"=w1303, "User Action"="User Pressed Select Load Head", "main ref"=w1258) -> ("error out"=w1299:errorcluster)  [unwired: 6 in, 1 out]
        n817 = Unbundle By Name(w1258) -> ("Loading.Enter the Final Load (N)"=w1274:refnum<vi>)
        n818 = Unbundle By Name(w1258) -> ("Loading.DecaForce COM Status"=w1260:refnum<vi>)
        n819 = Unbundle By Name(w1258) -> ("Loading.Loading Mode"=w1302:refnum<vi>)
        n820 = Unbundle By Name(w1258) -> ("Config Screen.Select Load Head"=w1286:refnum<vi>)
        n821 = Unbundle By Name(w1258) -> ("Loading.Warning"=w1269:refnum<vi>)
        n822 = Unbundle By Name(w1258) -> ("Loading.Load Selection"=w1295:refnum<vi>)
        n823 = property class="Bool (strict)"(reference=w1286, "Value"=FALSE) -> (reference out=w1284:refnum<vi>, error out=w1285:errorcluster)  [unwired: 1 in]
        n824 = property class="TabCtl (strict)"(reference=w1295, "Value"=T6."Constant") -> (reference out=w1297:refnum<vi>, error out=w1296:errorcluster)  [unwired: 1 in]
        n825 = property class="Ring (strict)"(reference=w1302, error in=w1299, "Value"=u16 0) -> (reference out=w1300:refnum<vi>, error out=w1301:errorcluster)
        n826 = property class="DigNum (strict)"(reference=w1279, "DisabledEnum"=T15."Disabled and Grayed Out" ("Disabled")) -> (reference out=w1278:refnum<vi>, error out=w1280:errorcluster)  [unwired: 1 in]
        n827 = property class="DigNum (strict)"(reference=w1274, "DisabledEnum"=T15."Disabled and Grayed Out" ("Disabled")) -> (reference out=w1275:refnum<vi>, error out=w1273:errorcluster)  [unwired: 1 in]
        n828 = property class="TabCtl (strict)"(reference=w1269, "Visible"=FALSE) -> (reference out=w1268:refnum<vi>, error out=w1270:errorcluster)  [unwired: 1 in]
        n829 = property class="Bool (strict)"(reference=w1264, "Visible"=FALSE) -> (reference out=w1262:refnum<vi>, error out=w1263:errorcluster)  [unwired: 1 in]
        n830 = property class="Bool (strict)"(reference=w1260, "Visible"=FALSE) -> (reference out=w1255:refnum<vi>, error out=w1261:errorcluster)  [unwired: 1 in]
        n831 = Close Reference(reference=w1284, error in (no error)=w1285) -> (error out=w1282:errorcluster)
        n832 = Close Reference(reference=w1297, error in (no error)=w1296) -> (error out=w1288:errorcluster)
        n833 = Close Reference(reference=w1300, error in (no error)=w1301) -> (error out=w1290:errorcluster)
        n834 = Close Reference(reference=w1278, error in (no error)=w1280) -> (error out=w1272:errorcluster)
        n835 = Close Reference(reference=w1275, error in (no error)=w1273) -> (error out=w1271:errorcluster)
        n836 = Close Reference(reference=w1268, error in (no error)=w1270) -> (error out=w1267:errorcluster)
        n837 = Close Reference(reference=w1262, error in (no error)=w1263) -> (error out=w1257:errorcluster)
        n838 = Close Reference(reference=w1255, error in (no error)=w1261) -> (error out=w1256:errorcluster)
        n839 = Merge Errors(w1290, w1288, w1282, w1272, w1271, w1267, w1257, w1256) -> (w1289:errorcluster)
        n840 = Unbundle By Name(w1258) -> ("Main Home Screen.GUI"=w1291:refnum<vi>)
        n841 = property class="TabCtl (strict)"(reference=w1291, error in=w1289, "Value"=T4."Load Head") -> (reference out=w1293:refnum<vi>, error out=w1292:errorcluster)
        n842 = Close Reference(reference=w1293, error in (no error)=w1292) -> (error out=w1281:errorcluster)
      }
      frame "com 3" {
        n843 = call "DATA ENCRYPT STRING FILE WRITE.vi"("error in (no error)"=w1308, "User Action"="User Pressed Check Load Communication", "main ref"=w1305) -> ("error out"=w1307:errorcluster)  [unwired: 6 in, 1 out]
        n844 = call "SET LOAD PARAMETERS.vi"("error in (no error)"=w1307, "main ref"=w1305) -> ("error out"=w1306:errorcluster)  [unwired: 9 in]
      }
      frame "ZeroAll" {
        n845 = call "DATA ENCRYPT STRING FILE WRITE.vi"("error in (no error)"=w1315, "User Action"="User Pressed Zero All", "main ref"=w1311) -> ("error out"=w1314:errorcluster)  [unwired: 6 in, 1 out]
        n846 = local write "ZeroAll"(FALSE ("ZeroAll")) -> ()
        n847 = call "LOAD CELL FGV MAIN.vi"("Enum"=T16."ZEROALL", "error in (no error)"=w1314, "main ref"=w1311) -> ("error IO"=w1313:errorcluster)  [unwired: 8 in]
      }
      frame "Loading Mode" {
        n848 = Unbundle By Name(w1319) -> ("Loading.Loading Mode"=w1321:refnum<vi>)
        n849 = property class="Ring (strict)"(reference=w1321, error in=w1320) -> (reference out=w1323:refnum<vi>, error out=w1322:errorcluster, "Value"=w1317:u16)
        n850 = Close Reference(reference=w1323, error in (no error)=w1322) -> (error out=w1318:errorcluster)
        n851 = case shown="1" w1317 {
          tunnel: [w1338 w1355 w1367 w1379] -> w1324
          tunnel: w1319 -> [w1325 w1341 w1359 w1371]
          tunnel: w1318 -> [w1339 w1354 w1366 w1378]
          frame 0, Default {
            n852 = Unbundle By Name(w1325) -> ("Loading.Enter the Loading Rate (N/min)"=w1332:refnum<vi>)
            n853 = Unbundle By Name(w1325) -> ("Loading.Load Selection"=w1335:refnum<vi>)
            n854 = Unbundle By Name(w1325) -> ("Loading.Enter the Final Load (N)"=w1327:refnum<vi>)
            n855 = property class="TabCtl (strict)"(reference=w1335, "Value"=T6."Constant") -> (reference out=w1337:refnum<vi>, error out=w1336:errorcluster)  [unwired: 1 in]
            n856 = property class="DigNum (strict)"(reference=w1332, "DisabledEnum"=T15."Disabled and Grayed Out" ("Disabled")) -> (reference out=w1331:refnum<vi>, error out=w1333:errorcluster)  [unwired: 1 in]
            n857 = property class="DigNum (strict)"(reference=w1327, "DisabledEnum"=T15."Disabled and Grayed Out" ("Disabled")) -> (reference out=w1328:refnum<vi>, error out=w1326:errorcluster)  [unwired: 1 in]
            n858 = call "DATA ENCRYPT STRING FILE WRITE.vi"("error in (no error)"=w1339, "User Action"="User selected Constant Mode", "main ref"=w1325) -> ("error out"=w1338:errorcluster)  [unwired: 6 in, 1 out]
            n859 = Close Reference(reference=w1337, error in (no error)=w1336) -> ()  [unwired: 1 out]
            n860 = Close Reference(reference=w1331, error in (no error)=w1333) -> ()  [unwired: 1 out]
            n861 = Close Reference(reference=w1328, error in (no error)=w1326) -> ()  [unwired: 1 out]
          }
          frame 1 {
            n862 = Unbundle By Name(w1341) -> ("Loading.Enter the Loading Rate (N/min)"=w1352:refnum<vi>)
            n863 = Unbundle By Name(w1341) -> ("Loading.Enter the Final Load (N)"=w1347:refnum<vi>)
            n864 = Unbundle By Name(w1341) -> ("Loading.Load Selection"=w1343:refnum<vi>)
            n865 = property class="TabCtl (strict)"(reference=w1343, "Value"=T6."Constant") -> (reference out=w1345:refnum<vi>, error out=w1344:errorcluster)  [unwired: 1 in]
            n866 = property class="DigNum (strict)"(reference=w1352, "DisabledEnum"=T15."Enabled" ("Disabled")) -> (reference out=w1351:refnum<vi>, error out=w1353:errorcluster)  [unwired: 1 in]
            n867 = property class="DigNum (strict)"(reference=w1347, "DisabledEnum"=T15."Enabled" ("Disabled")) -> (reference out=w1348:refnum<vi>, error out=w1346:errorcluster)  [unwired: 1 in]
            n868 = call "DATA ENCRYPT STRING FILE WRITE.vi"("error in (no error)"=w1354, "User Action"="User selected Ramp Mode", "main ref"=w1341) -> ("error out"=w1355:errorcluster)  [unwired: 6 in, 1 out]
            n869 = Close Reference(reference=w1345, error in (no error)=w1344) -> ()  [unwired: 1 out]
            n870 = Close Reference(reference=w1351, error in (no error)=w1353) -> ()  [unwired: 1 out]
            n871 = Close Reference(reference=w1348, error in (no error)=w1346) -> ()  [unwired: 1 out]
          }
          frame 2 {
            n872 = Unbundle By Name(w1359) -> ("Loading.Load Selection"=w1363:refnum<vi>)
            n873 = Unbundle By Name(w1359) -> ("Loading.Warning 2"=w1361:refnum<vi>)
            n874 = property class="TabCtl (strict)"(reference=w1363, "Value"=T6."Step") -> (reference out=w1365:refnum<vi>, error out=w1364:errorcluster)  [unwired: 1 in]
            n875 = property class="Bool (strict)"(reference=w1361, "Visible"=FALSE) -> (reference out=w1357:refnum<vi>, error out=w1360:errorcluster)  [unwired: 1 in]
            n876 = call "DATA ENCRYPT STRING FILE WRITE.vi"("error in (no error)"=w1366, "User Action"="User selected Step Mode", "main ref"=w1359) -> ("error out"=w1367:errorcluster)  [unwired: 6 in, 1 out]
            n877 = Close Reference(reference=w1365, error in (no error)=w1364) -> ()  [unwired: 1 out]
            n878 = Close Reference(reference=w1357, error in (no error)=w1360) -> ()  [unwired: 1 out]
          }
          frame 3 {
            n879 = Unbundle By Name(w1371) -> ("Loading.Load Selection"=w1375:refnum<vi>)
            n880 = Unbundle By Name(w1371) -> ("Loading.Warning 2"=w1373:refnum<vi>)
            n881 = property class="TabCtl (strict)"(reference=w1375, "Value"=T6."Indentation") -> (reference out=w1377:refnum<vi>, error out=w1376:errorcluster)  [unwired: 1 in]
            n882 = property class="Bool (strict)"(reference=w1373, "Visible"=FALSE) -> (reference out=w1369:refnum<vi>, error out=w1372:errorcluster)  [unwired: 1 in]
            n883 = call "DATA ENCRYPT STRING FILE WRITE.vi"("error in (no error)"=w1378, "User Action"="User selected Indentation Mode", "main ref"=w1371) -> ("error out"=w1379:errorcluster)  [unwired: 6 in, 1 out]
            n884 = Close Reference(reference=w1377, error in (no error)=w1376) -> ()  [unwired: 1 out]
            n885 = Close Reference(reference=w1369, error in (no error)=w1372) -> ()  [unwired: 1 out]
          }
        }
      }
      frame "SSP 0.3" {
        n886 = Unbundle By Name(w1383) -> ("Loading.SSP 0.3"=w1386:refnum<vi>)
        n887 = property class="Bool (strict)"(reference=w1386, error in=w1385) -> (reference out=w1388:refnum<vi>, error out=w1387:errorcluster, "Value"=w1384:bool)
        n888 = Close Reference(reference=w1388, error in (no error)=w1387) -> (error out=w1382:errorcluster)
        n889 = case shown="True" w1384 {
          tunnel: w1383 -> [_ w1390]
          tunnel: w1382 -> [w1389 w1398]
          tunnel: [w1389 w1397] -> w1381
          frame False {
          }
          frame True {
            w1400 = FALSE ("Value")
            n890 = Unbundle By Name(w1390) -> ("Loading.Enter the Load  (N)"=w1396:refnum<vi>)
            n891 = Unbundle By Name(w1390) -> ("Loading.SSP 0.75"=w1401:refnum<vi>)
            n892 = Unbundle By Name(w1390) -> ("Loading.SSP 0.5"=w1406:refnum<vi>)
            n893 = property class="Bool (strict)"(reference=w1401, "Value"=w1400) -> (reference out=w1403:refnum<vi>, error out=w1402:errorcluster)  [unwired: 1 in]
            n894 = property class="Bool (strict)"(reference=w1406, "Value"=w1400) -> (reference out=w1404:refnum<vi>, error out=w1405:errorcluster)  [unwired: 1 in]
            n895 = property class="DigNum (strict)"(reference=w1396, "Minimum"=2.0 ("Data Entry Limits:Minimum"), "Maximum"=50.0 ("Data Entry Limits:Maximum"), "Increment"=0.1 ("Data Entry Limits:Increment")) -> (reference out=w1394:refnum<vi>, error out=w1395:errorcluster)  [unwired: 1 in]
            n896 = call "DATA ENCRYPT STRING FILE WRITE.vi"("error in (no error)"=w1398, "User Action"="User selected 0.3 SSP", "main ref"=w1390) -> ("error out"=w1397:errorcluster)  [unwired: 6 in, 1 out]
            n897 = Close Reference(reference=w1403, error in (no error)=w1402) -> ()  [unwired: 1 out]
            n898 = Close Reference(reference=w1404, error in (no error)=w1405) -> ()  [unwired: 1 out]
            n899 = Close Reference(reference=w1394, error in (no error)=w1395) -> ()  [unwired: 1 out]
          }
        }
      }
      frame "SSP 0.5" {
        n900 = Unbundle By Name(w1409) -> ("Loading.SSP 0.5"=w1412:refnum<vi>)
        n901 = property class="Bool (strict)"(reference=w1412, error in=w1411) -> (reference out=w1414:refnum<vi>, error out=w1413:errorcluster, "Value"=w1410:bool)
        n902 = Close Reference(reference=w1414, error in (no error)=w1413) -> (error out=w1408:errorcluster)
        n903 = case shown="True" w1410 {
          tunnel: w1409 -> [_ w1416]
          tunnel: w1408 -> [w1415 w1424]
          tunnel: [w1415 w1423] -> w1407
          frame False {
          }
          frame True {
            w1426 = FALSE ("Value")
            n904 = Unbundle By Name(w1416) -> ("Loading.Enter the Load  (N)"=w1422:refnum<vi>)
            n905 = Unbundle By Name(w1416) -> ("Loading.SSP 0.75"=w1432:refnum<vi>)
            n906 = Unbundle By Name(w1416) -> ("Loading.SSP 0.3"=w1427:refnum<vi>)
            n907 = property class="Bool (strict)"(reference=w1427, "Value"=w1426) -> (reference out=w1429:refnum<vi>, error out=w1428:errorcluster)  [unwired: 1 in]
            n908 = property class="Bool (strict)"(reference=w1432, "Value"=w1426) -> (reference out=w1430:refnum<vi>, error out=w1431:errorcluster)  [unwired: 1 in]
            n909 = property class="DigNum (strict)"(reference=w1422, "Minimum"=2.0 ("Data Entry Limits:Minimum"), "Maximum"=200.0 ("Data Entry Limits:Maximum"), "Increment"=0.1 ("Data Entry Limits:Increment")) -> (reference out=w1420:refnum<vi>, error out=w1421:errorcluster)  [unwired: 1 in]
            n910 = call "DATA ENCRYPT STRING FILE WRITE.vi"("error in (no error)"=w1424, "User Action"="User selected 0.5 SSP", "main ref"=w1416) -> ("error out"=w1423:errorcluster)  [unwired: 6 in, 1 out]
            n911 = Close Reference(reference=w1429, error in (no error)=w1428) -> ()  [unwired: 1 out]
            n912 = Close Reference(reference=w1430, error in (no error)=w1431) -> ()  [unwired: 1 out]
            n913 = Close Reference(reference=w1420, error in (no error)=w1421) -> ()  [unwired: 1 out]
          }
        }
      }
      frame "SSP 0.75" {
        n914 = Unbundle By Name(w1435) -> ("Loading.SSP 0.75"=w1438:refnum<vi>)
        n915 = property class="Bool (strict)"(reference=w1438, error in=w1437) -> (reference out=w1440:refnum<vi>, error out=w1439:errorcluster, "Value"=w1436:bool)
        n916 = Close Reference(reference=w1440, error in (no error)=w1439) -> (error out=w1434:errorcluster)
        n917 = case shown="True" w1436 {
          tunnel: w1435 -> [_ w1442]
          tunnel: w1434 -> [w1441 w1450]
          tunnel: [w1441 w1449] -> w1433
          frame False {
          }
          frame True {
            w1452 = FALSE ("Value")
            n918 = Unbundle By Name(w1442) -> ("Loading.SSP 0.3"=w1453:refnum<vi>)
            n919 = Unbundle By Name(w1442) -> ("Loading.SSP 0.5"=w1458:refnum<vi>)
            n920 = Unbundle By Name(w1442) -> ("Loading.Enter the Load  (N)"=w1448:refnum<vi>)
            n921 = property class="Bool (strict)"(reference=w1453, "Value"=w1452) -> (reference out=w1455:refnum<vi>, error out=w1454:errorcluster)  [unwired: 1 in]
            n922 = property class="Bool (strict)"(reference=w1458, "Value"=w1452) -> (reference out=w1456:refnum<vi>, error out=w1457:errorcluster)  [unwired: 1 in]
            n923 = property class="DigNum (strict)"(reference=w1448, "Minimum"=200.0 ("Data Entry Limits:Minimum"), "Maximum"=500.0 ("Data Entry Limits:Maximum"), "Increment"=0.1 ("Data Entry Limits:Increment")) -> (reference out=w1446:refnum<vi>, error out=w1447:errorcluster)  [unwired: 1 in]
            n924 = call "DATA ENCRYPT STRING FILE WRITE.vi"("error in (no error)"=w1450, "User Action"="User selected 0.75 SSP", "main ref"=w1442) -> ("error out"=w1449:errorcluster)  [unwired: 6 in, 1 out]
            n925 = Close Reference(reference=w1455, error in (no error)=w1454) -> ()  [unwired: 1 out]
            n926 = Close Reference(reference=w1456, error in (no error)=w1457) -> ()  [unwired: 1 out]
            n927 = Close Reference(reference=w1446, error in (no error)=w1447) -> ()  [unwired: 1 out]
          }
        }
      }
      frame "LHBack" {
        # "Back to Configure"
        n928 = Unbundle By Name(w1459) -> ("Main Home Screen.GUI"=w1465:refnum<vi>)
        n929 = Unbundle By Name(w1459) -> ("Main Home Screen.MainPage"=w1461:refnum<vi>)
        n930 = property class="TabCtl (strict)"(reference=w1461, "Value"=T5."HOME") -> (reference out=w1463:refnum<vi>, error out=w1462:errorcluster)  [unwired: 1 in]
        n931 = property class="TabCtl (strict)"(reference=w1465, "Value"=T4."Setup") -> (reference out=w1467:refnum<vi>, error out=w1466:errorcluster)  [unwired: 1 in]
        n932 = Close Reference(reference=w1463, error in (no error)=w1462) -> ()  [unwired: 1 out]
        n933 = Close Reference(reference=w1467, error in (no error)=w1466) -> ()  [unwired: 1 out]
        n934 = call "DATA ENCRYPT STRING FILE WRITE.vi"("error in (no error)"=w1468, "User Action"="User selected Back to Configure", "main ref"=w1459) -> ("error out"=w1469:errorcluster)  [unwired: 6 in, 1 out]
      }
      frame "MMBack" {
        # "Back to Configure"
        n935 = Unbundle By Name(w1471) -> ("Main Home Screen.GUI"=w1477:refnum<vi>)
        n936 = Unbundle By Name(w1471) -> ("Main Home Screen.MainPage"=w1473:refnum<vi>)
        n937 = property class="TabCtl (strict)"(reference=w1473, "Value"=T5."HOME") -> (reference out=w1475:refnum<vi>, error out=w1474:errorcluster)  [unwired: 1 in]
        n938 = property class="TabCtl (strict)"(reference=w1477, "Value"=T4."Load Head") -> (reference out=w1479:refnum<vi>, error out=w1478:errorcluster)  [unwired: 1 in]
        n939 = Close Reference(reference=w1475, error in (no error)=w1474) -> ()  [unwired: 1 out]
        n940 = Close Reference(reference=w1479, error in (no error)=w1478) -> ()  [unwired: 1 out]
        n941 = call "DATA ENCRYPT STRING FILE WRITE.vi"("error in (no error)"=w1480, "User Action"="User selected Back to Load Selection", "main ref"=w1471) -> ("error out"=w1481:errorcluster)  [unwired: 6 in, 1 out]
      }
      frame "LHNext" {
        w1513 = FALSE ("Visible")
        n942 = Unbundle By Name(w1483) -> ("Motion Module.HomeRot"=w1519:refnum<vi>)
        n943 = Unbundle By Name(w1483) -> ("Motion Module.HomeScratch"=w1514:refnum<vi>)
        n944 = Unbundle By Name(w1483) -> ("Motion Module.PlaceModule"=w1512:refnum<vi>)
        n945 = Unbundle By Name(w1483) -> ("Motion Module.Motion Mode:"=w1505:refnum<vi>)
        n946 = Unbundle By Name(w1483) -> ("Motion Module.Motion Direction:  3"=w1504:refnum<vi>)
        n947 = Unbundle By Name(w1483) -> ("Motion Module.Wear Track Diameter (mm)"=w1498:refnum<vi>)
        n948 = Unbundle By Name(w1483) -> ("Motion Module.Set WTD"=w1495:refnum<vi>)
        n949 = Unbundle By Name(w1483) -> ("Motion Module.Rotary Module Selection"=w1489:refnum<vi>)
        n950 = call "DATA ENCRYPT STRING FILE WRITE.vi"("error in (no error)"=w1528, "User Action"="User selected Select Module", "main ref"=w1483) -> ("error out"=w1492:errorcluster)  [unwired: 6 in, 1 out]
        n951 = property class="TabCtl (strict)"(reference=w1489, "Visible"=FALSE) -> (reference out=w1488:refnum<vi>, error out=w1490:errorcluster)  [unwired: 1 in]
        n952 = property class="Bool (strict)"(reference=w1519, error in=w1492, "Visible"=w1513) -> (reference out=w1517:refnum<vi>, error out=w1518:errorcluster)
        n953 = property class="Bool (strict)"(reference=w1514, error in=w1492, "Visible"=w1513) -> (reference out=w1516:refnum<vi>, error out=w1515:errorcluster)
        n954 = property class="Bool (strict)"(reference=w1512, error in=w1492, "Visible"=TRUE) -> (reference out=w1510:refnum<vi>, error out=w1511:errorcluster)
        n955 = property class="Ring (strict)"(reference=w1505, error in=w1492, "Visible"=FALSE) -> (reference out=w1507:refnum<vi>, error out=w1506:errorcluster)
        n956 = property class="Ring (strict)"(reference=w1504, error in=w1492, "Visible"=FALSE) -> (reference out=w1501:refnum<vi>, error out=w1503:errorcluster)
        n957 = property class="DigNum (strict)"(reference=w1498, "Visible"=FALSE) -> (reference out=w1497:refnum<vi>, error out=w1499:errorcluster)  [unwired: 1 in]
        n958 = property class="Bool (strict)"(reference=w1495, "Visible"=FALSE) -> (reference out=w1496:refnum<vi>, error out=w1494:errorcluster)  [unwired: 1 in]
        n959 = Close Reference(reference=w1517, error in (no error)=w1518) -> ()  [unwired: 1 out]
        n960 = Close Reference(reference=w1516, error in (no error)=w1515) -> ()  [unwired: 1 out]
        n961 = Close Reference(reference=w1510, error in (no error)=w1511) -> ()  [unwired: 1 out]
        n962 = Close Reference(reference=w1507, error in (no error)=w1506) -> ()  [unwired: 1 out]
        n963 = Close Reference(reference=w1501, error in (no error)=w1503) -> ()  [unwired: 1 out]
        n964 = Close Reference(reference=w1497, error in (no error)=w1499) -> ()  [unwired: 1 out]
        n965 = Close Reference(reference=w1488, error in (no error)=w1490) -> ()  [unwired: 1 out]
        n966 = Close Reference(reference=w1496, error in (no error)=w1494) -> ()  [unwired: 1 out]
        n967 = Unbundle By Name(w1483) -> ("Motion Module.M3 Image"=w1487:refnum<vi>)
        n968 = Unbundle By Name(w1483) -> ("Main Home Screen.GUI"=w1525:refnum<vi>)
        n969 = Unbundle By Name(w1483) -> ("Main Home Screen.MainPage"=w1521:refnum<vi>)
        n970 = property class="TabCtl (strict)"(reference=w1487, "Value"=enum32{"Page 1", "Page 2"}."Page 2") -> (reference out=w1485:refnum<vi>, error out=w1486:errorcluster)  [unwired: 1 in]
        n971 = property class="TabCtl (strict)"(reference=w1521, "Value"=T5."HOME") -> (reference out=w1523:refnum<vi>, error out=w1522:errorcluster)  [unwired: 1 in]
        n972 = property class="TabCtl (strict)"(reference=w1525, "Value"=T4."Motion Module") -> (reference out=w1527:refnum<vi>, error out=w1526:errorcluster)  [unwired: 1 in]
        n973 = Close Reference(reference=w1485, error in (no error)=w1486) -> ()  [unwired: 1 out]
        n974 = Close Reference(reference=w1523, error in (no error)=w1522) -> ()  [unwired: 1 out]
        n975 = Close Reference(reference=w1527, error in (no error)=w1526) -> ()  [unwired: 1 out]
      }
      frame "Rot Ver" {
        # "Rot Ver"
        n976 = Unbundle By Name(w1532) -> ("Motion Module.Rot Ver"=w1531:refnum<vi>)
        n977 = property class="Bool (strict)"(reference=w1531) -> (reference out=w1534:refnum<vi>, error out=w1533:errorcluster, "Value"=w1530:bool)  [unwired: 1 in]
        n978 = Close Reference(reference=w1534, error in (no error)=w1533) -> ()  [unwired: 1 out]
        n979 = case shown="True" w1530 {
          tunnel: w1548 -> [w1583 w1618]
          tunnel: [w1555 w1618] -> w1539
          tunnel: w1532 -> [w1549 w1585]
          frame True {
            n980 = Unbundle By Name(w1549) -> ("Motion Module.HomeRot"=w1582:refnum<vi>)
            n981 = Unbundle By Name(w1549) -> ("Motion Module.HomeScratch"=w1577:refnum<vi>)
            n982 = Unbundle By Name(w1549) -> ("Motion Module.PlaceModule"=w1575:refnum<vi>)
            n983 = Unbundle By Name(w1549) -> ("Motion Module.Motion Mode:"=w1568:refnum<vi>)
            n984 = Unbundle By Name(w1549) -> ("Motion Module.Motion Direction:  3"=w1567:refnum<vi>)
            n985 = Unbundle By Name(w1549) -> ("Motion Module.Wear Track Diameter (mm)"=w1561:refnum<vi>)
            n986 = Unbundle By Name(w1549) -> ("Motion Module.Set WTD"=w1558:refnum<vi>)
            n987 = Unbundle By Name(w1549) -> ("Motion Module.Rotary Module Selection"=w1552:refnum<vi>)
            n988 = call "DATA ENCRYPT STRING FILE WRITE.vi"("error in (no error)"=w1583, "User Action"="User selected Rot Vertical Module", "main ref"=w1549) -> ("error out"=w1555:errorcluster)  [unwired: 6 in, 1 out]
            n989 = property class="TabCtl (strict)"(reference=w1552, "Visible"=TRUE) -> (reference out=w1551:refnum<vi>, error out=w1553:errorcluster)  [unwired: 1 in]
            n990 = property class="Bool (strict)"(reference=w1582, error in=w1555, "Visible"=TRUE) -> (reference out=w1580:refnum<vi>, error out=w1581:errorcluster)
            n991 = property class="Bool (strict)"(reference=w1577, error in=w1555, "Visible"=FALSE) -> (reference out=w1579:refnum<vi>, error out=w1578:errorcluster)
            n992 = property class="Bool (strict)"(reference=w1575, error in=w1555, "Visible"=FALSE) -> (reference out=w1573:refnum<vi>, error out=w1574:errorcluster)
            n993 = property class="Ring (strict)"(reference=w1568, error in=w1555, "Visible"=TRUE) -> (reference out=w1570:refnum<vi>, error out=w1569:errorcluster)
            n994 = property class="Ring (strict)"(reference=w1567, error in=w1555, "Visible"=TRUE) -> (reference out=w1564:refnum<vi>, error out=w1566:errorcluster)
            n995 = property class="DigNum (strict)"(reference=w1561, "Visible"=TRUE) -> (reference out=w1560:refnum<vi>, error out=w1562:errorcluster)  [unwired: 1 in]
            n996 = property class="Bool (strict)"(reference=w1558, "Visible"=TRUE) -> (reference out=w1559:refnum<vi>, error out=w1557:errorcluster)  [unwired: 1 in]
            n997 = Close Reference(reference=w1580, error in (no error)=w1581) -> ()  [unwired: 1 out]
            n998 = Close Reference(reference=w1579, error in (no error)=w1578) -> ()  [unwired: 1 out]
            n999 = Close Reference(reference=w1573, error in (no error)=w1574) -> ()  [unwired: 1 out]
            n1000 = Close Reference(reference=w1570, error in (no error)=w1569) -> ()  [unwired: 1 out]
            n1001 = Close Reference(reference=w1564, error in (no error)=w1566) -> ()  [unwired: 1 out]
            n1002 = Close Reference(reference=w1560, error in (no error)=w1562) -> ()  [unwired: 1 out]
            n1003 = Close Reference(reference=w1551, error in (no error)=w1553) -> ()  [unwired: 1 out]
            n1004 = Close Reference(reference=w1559, error in (no error)=w1557) -> ()  [unwired: 1 out]
          }
          frame False {
            n1005 = Unbundle By Name(w1585) -> ("Motion Module.HomeRot"=w1617:refnum<vi>)
            n1006 = Unbundle By Name(w1585) -> ("Motion Module.HomeScratch"=w1612:refnum<vi>)
            n1007 = Unbundle By Name(w1585) -> ("Motion Module.PlaceModule"=w1610:refnum<vi>)
            n1008 = Unbundle By Name(w1585) -> ("Motion Module.Motion Mode:"=w1603:refnum<vi>)
            n1009 = Unbundle By Name(w1585) -> ("Motion Module.Motion Direction:  3"=w1602:refnum<vi>)
            n1010 = Unbundle By Name(w1585) -> ("Motion Module.Wear Track Diameter (mm)"=w1596:refnum<vi>)
            n1011 = Unbundle By Name(w1585) -> ("Motion Module.Set WTD"=w1593:refnum<vi>)
            n1012 = Unbundle By Name(w1585) -> ("Motion Module.Rotary Module Selection"=w1588:refnum<vi>)
            n1013 = property class="TabCtl (strict)"(reference=w1588, "Visible"=FALSE) -> (reference out=w1587:refnum<vi>, error out=w1589:errorcluster)  [unwired: 1 in]
            n1014 = property class="Bool (strict)"(reference=w1617, error in=w1618, "Visible"=FALSE) -> (reference out=w1615:refnum<vi>, error out=w1616:errorcluster)
            n1015 = property class="Bool (strict)"(reference=w1612, error in=w1618, "Visible"=FALSE) -> (reference out=w1614:refnum<vi>, error out=w1613:errorcluster)
            n1016 = property class="Bool (strict)"(reference=w1610, error in=w1618, "Visible"=TRUE) -> (reference out=w1608:refnum<vi>, error out=w1609:errorcluster)
            n1017 = property class="Ring (strict)"(reference=w1603, error in=w1618, "Visible"=FALSE) -> (reference out=w1605:refnum<vi>, error out=w1604:errorcluster)
            n1018 = property class="Ring (strict)"(reference=w1602, error in=w1618, "Visible"=FALSE) -> (reference out=w1599:refnum<vi>, error out=w1601:errorcluster)
            n1019 = property class="DigNum (strict)"(reference=w1596, "Visible"=FALSE) -> (reference out=w1595:refnum<vi>, error out=w1597:errorcluster)  [unwired: 1 in]
            n1020 = property class="Bool (strict)"(reference=w1593, "Visible"=FALSE) -> (reference out=w1594:refnum<vi>, error out=w1592:errorcluster)  [unwired: 1 in]
            n1021 = Close Reference(reference=w1615, error in (no error)=w1616) -> ()  [unwired: 1 out]
            n1022 = Close Reference(reference=w1614, error in (no error)=w1613) -> ()  [unwired: 1 out]
            n1023 = Close Reference(reference=w1608, error in (no error)=w1609) -> ()  [unwired: 1 out]
            n1024 = Close Reference(reference=w1605, error in (no error)=w1604) -> ()  [unwired: 1 out]
            n1025 = Close Reference(reference=w1599, error in (no error)=w1601) -> ()  [unwired: 1 out]
            n1026 = Close Reference(reference=w1595, error in (no error)=w1597) -> ()  [unwired: 1 out]
            n1027 = Close Reference(reference=w1587, error in (no error)=w1589) -> ()  [unwired: 1 out]
            n1028 = Close Reference(reference=w1594, error in (no error)=w1592) -> ()  [unwired: 1 out]
          }
        }
        n1029 = Unbundle By Name(w1532) -> ("Motion Module.M3 Image"=w1538:refnum<vi>)
        n1030 = Unbundle By Name(w1532) -> ("Main Home Screen.GUI"=w1545:refnum<vi>)
        n1031 = Unbundle By Name(w1532) -> ("Main Home Screen.MainPage"=w1541:refnum<vi>)
        n1032 = property class="TabCtl (strict)"(reference=w1538, "Value"=enum32{"Page 1", "Page 2"}."Page 1") -> (reference out=w1536:refnum<vi>, error out=w1537:errorcluster)  [unwired: 1 in]
        n1033 = property class="TabCtl (strict)"(reference=w1541, "Value"=T5."HOME") -> (reference out=w1543:refnum<vi>, error out=w1542:errorcluster)  [unwired: 1 in]
        n1034 = property class="TabCtl (strict)"(reference=w1545, "Value"=T4."Motion Module") -> (reference out=w1547:refnum<vi>, error out=w1546:errorcluster)  [unwired: 1 in]
        n1035 = Close Reference(reference=w1536, error in (no error)=w1537) -> ()  [unwired: 1 out]
        n1036 = Close Reference(reference=w1543, error in (no error)=w1542) -> ()  [unwired: 1 out]
        n1037 = Close Reference(reference=w1547, error in (no error)=w1546) -> ()  [unwired: 1 out]
      }
      frame "Scratch" {
        n1038 = Unbundle By Name(w1620) -> ("Motion Module.Scratch"=w1621:refnum<vi>)
        n1039 = property class="Bool (strict)"(reference=w1621) -> (reference out=w1623:refnum<vi>, error out=w1622:errorcluster, "Value"=w1619:bool)  [unwired: 1 in]
        n1040 = Close Reference(reference=w1623, error in (no error)=w1622) -> ()  [unwired: 1 out]
        n1041 = case shown="True" w1619 {
          tunnel: w1637 -> [w1672 w1707]
          tunnel: [w1644 w1707] -> w1628
          tunnel: w1620 -> [w1638 w1674]
          frame True {
            n1042 = Unbundle By Name(w1638) -> ("Motion Module.HomeRot"=w1671:refnum<vi>)
            n1043 = Unbundle By Name(w1638) -> ("Motion Module.HomeScratch"=w1666:refnum<vi>)
            n1044 = Unbundle By Name(w1638) -> ("Motion Module.PlaceModule"=w1664:refnum<vi>)
            n1045 = Unbundle By Name(w1638) -> ("Motion Module.Motion Mode:"=w1657:refnum<vi>)
            n1046 = Unbundle By Name(w1638) -> ("Motion Module.Motion Direction:  3"=w1656:refnum<vi>)
            n1047 = Unbundle By Name(w1638) -> ("Motion Module.Wear Track Diameter (mm)"=w1650:refnum<vi>)
            n1048 = Unbundle By Name(w1638) -> ("Motion Module.Set WTD"=w1647:refnum<vi>)
            n1049 = Unbundle By Name(w1638) -> ("Motion Module.Rotary Module Selection"=w1641:refnum<vi>)
            n1050 = call "DATA ENCRYPT STRING FILE WRITE.vi"("error in (no error)"=w1672, "User Action"="User selected Scratch Module", "main ref"=w1638) -> ("error out"=w1644:errorcluster)  [unwired: 6 in, 1 out]
            n1051 = property class="TabCtl (strict)"(reference=w1641, "Visible"=FALSE) -> (reference out=w1640:refnum<vi>, error out=w1642:errorcluster)  [unwired: 1 in]
            n1052 = property class="Bool (strict)"(reference=w1671, error in=w1644, "Visible"=FALSE) -> (reference out=w1669:refnum<vi>, error out=w1670:errorcluster)
            n1053 = property class="Bool (strict)"(reference=w1666, error in=w1644, "Visible"=TRUE) -> (reference out=w1668:refnum<vi>, error out=w1667:errorcluster)
            n1054 = property class="Bool (strict)"(reference=w1664, error in=w1644, "Visible"=FALSE) -> (reference out=w1662:refnum<vi>, error out=w1663:errorcluster)
            n1055 = property class="Ring (strict)"(reference=w1657, error in=w1644, "Visible"=FALSE) -> (reference out=w1659:refnum<vi>, error out=w1658:errorcluster)
            n1056 = property class="Ring (strict)"(reference=w1656, error in=w1644, "Visible"=FALSE) -> (reference out=w1653:refnum<vi>, error out=w1655:errorcluster)
            n1057 = property class="DigNum (strict)"(reference=w1650, "Visible"=FALSE) -> (reference out=w1649:refnum<vi>, error out=w1651:errorcluster)  [unwired: 1 in]
            n1058 = property class="Bool (strict)"(reference=w1647, "Visible"=FALSE) -> (reference out=w1648:refnum<vi>, error out=w1646:errorcluster)  [unwired: 1 in]
            n1059 = Close Reference(reference=w1669, error in (no error)=w1670) -> ()  [unwired: 1 out]
            n1060 = Close Reference(reference=w1668, error in (no error)=w1667) -> ()  [unwired: 1 out]
            n1061 = Close Reference(reference=w1662, error in (no error)=w1663) -> ()  [unwired: 1 out]
            n1062 = Close Reference(reference=w1659, error in (no error)=w1658) -> ()  [unwired: 1 out]
            n1063 = Close Reference(reference=w1653, error in (no error)=w1655) -> ()  [unwired: 1 out]
            n1064 = Close Reference(reference=w1649, error in (no error)=w1651) -> ()  [unwired: 1 out]
            n1065 = Close Reference(reference=w1640, error in (no error)=w1642) -> ()  [unwired: 1 out]
            n1066 = Close Reference(reference=w1648, error in (no error)=w1646) -> ()  [unwired: 1 out]
          }
          frame False {
            n1067 = Unbundle By Name(w1674) -> ("Motion Module.HomeRot"=w1706:refnum<vi>)
            n1068 = Unbundle By Name(w1674) -> ("Motion Module.HomeScratch"=w1701:refnum<vi>)
            n1069 = Unbundle By Name(w1674) -> ("Motion Module.PlaceModule"=w1699:refnum<vi>)
            n1070 = Unbundle By Name(w1674) -> ("Motion Module.Motion Mode:"=w1692:refnum<vi>)
            n1071 = Unbundle By Name(w1674) -> ("Motion Module.Motion Direction:  3"=w1691:refnum<vi>)
            n1072 = Unbundle By Name(w1674) -> ("Motion Module.Wear Track Diameter (mm)"=w1685:refnum<vi>)
            n1073 = Unbundle By Name(w1674) -> ("Motion Module.Set WTD"=w1682:refnum<vi>)
            n1074 = Unbundle By Name(w1674) -> ("Motion Module.Rotary Module Selection"=w1677:refnum<vi>)
            n1075 = property class="TabCtl (strict)"(reference=w1677, "Visible"=FALSE) -> (reference out=w1676:refnum<vi>, error out=w1678:errorcluster)  [unwired: 1 in]
            n1076 = property class="Bool (strict)"(reference=w1706, error in=w1707, "Visible"=FALSE) -> (reference out=w1704:refnum<vi>, error out=w1705:errorcluster)
            n1077 = property class="Bool (strict)"(reference=w1701, error in=w1707, "Visible"=FALSE) -> (reference out=w1703:refnum<vi>, error out=w1702:errorcluster)
            n1078 = property class="Bool (strict)"(reference=w1699, error in=w1707, "Visible"=TRUE) -> (reference out=w1697:refnum<vi>, error out=w1698:errorcluster)
            n1079 = property class="Ring (strict)"(reference=w1692, error in=w1707, "Visible"=FALSE) -> (reference out=w1694:refnum<vi>, error out=w1693:errorcluster)
            n1080 = property class="Ring (strict)"(reference=w1691, error in=w1707, "Visible"=FALSE) -> (reference out=w1688:refnum<vi>, error out=w1690:errorcluster)
            n1081 = property class="DigNum (strict)"(reference=w1685, "Visible"=FALSE) -> (reference out=w1684:refnum<vi>, error out=w1686:errorcluster)  [unwired: 1 in]
            n1082 = property class="Bool (strict)"(reference=w1682, "Visible"=FALSE) -> (reference out=w1683:refnum<vi>, error out=w1681:errorcluster)  [unwired: 1 in]
            n1083 = Close Reference(reference=w1704, error in (no error)=w1705) -> ()  [unwired: 1 out]
            n1084 = Close Reference(reference=w1703, error in (no error)=w1702) -> ()  [unwired: 1 out]
            n1085 = Close Reference(reference=w1697, error in (no error)=w1698) -> ()  [unwired: 1 out]
            n1086 = Close Reference(reference=w1694, error in (no error)=w1693) -> ()  [unwired: 1 out]
            n1087 = Close Reference(reference=w1688, error in (no error)=w1690) -> ()  [unwired: 1 out]
            n1088 = Close Reference(reference=w1684, error in (no error)=w1686) -> ()  [unwired: 1 out]
            n1089 = Close Reference(reference=w1676, error in (no error)=w1678) -> ()  [unwired: 1 out]
            n1090 = Close Reference(reference=w1683, error in (no error)=w1681) -> ()  [unwired: 1 out]
          }
        }
        n1091 = Unbundle By Name(w1620) -> ("Main Home Screen.GUI"=w1634:refnum<vi>)
        n1092 = Unbundle By Name(w1620) -> ("Main Home Screen.MainPage"=w1630:refnum<vi>)
        n1093 = Unbundle By Name(w1620) -> ("Motion Module.M3 Image"=w1627:refnum<vi>)
        n1094 = property class="TabCtl (strict)"(reference=w1630, "Value"=T5."HOME") -> (reference out=w1632:refnum<vi>, error out=w1631:errorcluster)  [unwired: 1 in]
        n1095 = property class="TabCtl (strict)"(reference=w1627, "Value"=enum32{"Page 1", "Page 2"}."Page 2") -> (reference out=w1625:refnum<vi>, error out=w1626:errorcluster)  [unwired: 1 in]
        n1096 = property class="TabCtl (strict)"(reference=w1634, "Value"=T4."Motion Module") -> (reference out=w1636:refnum<vi>, error out=w1635:errorcluster)  [unwired: 1 in]
        n1097 = Close Reference(reference=w1632, error in (no error)=w1631) -> ()  [unwired: 1 out]
        n1098 = Close Reference(reference=w1625, error in (no error)=w1626) -> ()  [unwired: 1 out]
        n1099 = Close Reference(reference=w1636, error in (no error)=w1635) -> ()  [unwired: 1 out]
      }
      frame "Motion Mode:" {
        n1100 = Unbundle By Name(w1708) -> ("Motion Module.Motion Mode:"=w1710:refnum<vi>)
        n1101 = property class="Ring (strict)"(reference=w1710) -> (reference out=w1712:refnum<vi>, error out=w1711:errorcluster, "Value"=w1709:u16)  [unwired: 1 in]
        n1102 = Close Reference(reference=w1712, error in (no error)=w1711) -> ()  [unwired: 1 out]
        n1103 = case shown="3" w1709 {
          tunnel: w1714 -> [w1723 w1732 w1741 w1750]
          tunnel: [w1722 w1731 w1740 w1749] -> w1713
          tunnel: w1708 -> [w1721 w1730 w1739 w1748]
          tunnel: w1708 -> [w1716 w1725 w1734 w1743]
          frame 0, Default {
            n1104 = Unbundle By Name(w1716) -> ("Motion Module.Rotary Module Selection"=w1717:refnum<vi>)
            n1105 = property class="TabCtl (strict)"(reference=w1717, "Value"=T7."Uniform Rotation") -> (reference out=w1719:refnum<vi>, error out=w1718:errorcluster)  [unwired: 1 in]
            n1106 = Close Reference(reference=w1719, error in (no error)=w1718) -> ()  [unwired: 1 out]
            n1107 = call "DATA ENCRYPT STRING FILE WRITE.vi"("error in (no error)"=w1723, "User Action"="User Selected Uniform Rotation", "main ref"=w1721) -> ("error out"=w1722:errorcluster)  [unwired: 6 in, 1 out]
          }
          frame 1 {
            n1108 = Unbundle By Name(w1725) -> ("Motion Module.Rotary Module Selection"=w1726:refnum<vi>)
            n1109 = property class="TabCtl (strict)"(reference=w1726, "Value"=T7."Angular Oscillation") -> (reference out=w1728:refnum<vi>, error out=w1727:errorcluster)  [unwired: 1 in]
            n1110 = Close Reference(reference=w1728, error in (no error)=w1727) -> ()  [unwired: 1 out]
            n1111 = call "DATA ENCRYPT STRING FILE WRITE.vi"("error in (no error)"=w1732, "User Action"="User Selected Angular Oscillation", "main ref"=w1730) -> ("error out"=w1731:errorcluster)  [unwired: 6 in, 1 out]
          }
          frame 2 {
            n1112 = Unbundle By Name(w1734) -> ("Motion Module.Rotary Module Selection"=w1735:refnum<vi>)
            n1113 = property class="TabCtl (strict)"(reference=w1735, "Value"=T7."Speed Ramp") -> (reference out=w1737:refnum<vi>, error out=w1736:errorcluster)  [unwired: 1 in]
            n1114 = Close Reference(reference=w1737, error in (no error)=w1736) -> ()  [unwired: 1 out]
            n1115 = call "DATA ENCRYPT STRING FILE WRITE.vi"("error in (no error)"=w1741, "User Action"="User Selected Ramp Mode", "main ref"=w1739) -> ("error out"=w1740:errorcluster)  [unwired: 6 in, 1 out]
          }
          frame 3 {
            n1116 = Unbundle By Name(w1743) -> ("Motion Module.Rotary Module Selection"=w1744:refnum<vi>)
            n1117 = property class="TabCtl (strict)"(reference=w1744, "Value"=T7."Speed Step") -> (reference out=w1746:refnum<vi>, error out=w1745:errorcluster)  [unwired: 1 in]
            n1118 = Close Reference(reference=w1746, error in (no error)=w1745) -> ()  [unwired: 1 out]
            n1119 = call "DATA ENCRYPT STRING FILE WRITE.vi"("error in (no error)"=w1750, "User Action"="User Selected Step Mode", "main ref"=w1748) -> ("error out"=w1749:errorcluster)  [unwired: 6 in, 1 out]
          }
        }
      }
      frame "MMNext" {
        n1120 = Unbundle By Name(w1751) -> ("Motion Module.MMNext"=w1758:refnum<vi>)
        n1121 = Unbundle By Name(w1751) -> ("Main Home Screen.GUI"=w1760:refnum<vi>)
        n1122 = property class="TabCtl (strict)"(reference=w1760, "Value"=T4."Environment") -> (reference out=w1762:refnum<vi>, error out=w1761:errorcluster)  [unwired: 1 in]
        n1123 = property class="Bool (strict)"(reference=w1758, "Value"=FALSE) -> (reference out=w1756:refnum<vi>, error out=w1757:errorcluster)  [unwired: 1 in]
        n1124 = Close Reference(reference=w1756, error in (no error)=w1757) -> ()  [unwired: 1 out]
        n1125 = Close Reference(reference=w1762, error in (no error)=w1761) -> ()  [unwired: 1 out]
        n1126 = call "DATA ENCRYPT STRING FILE WRITE.vi"("error in (no error)"=w1753, "User Action"="User Selected SetUp Module", "main ref"=w1751) -> ("error out"=w1752:errorcluster)  [unwired: 6 in, 1 out]
      }
      frame "APBack" {
        n1127 = Unbundle By Name(w1763) -> ("Environmental control.APBack"=w1770:refnum<vi>)
        n1128 = Unbundle By Name(w1763) -> ("Main Home Screen.GUI"=w1772:refnum<vi>)
        n1129 = property class="TabCtl (strict)"(reference=w1772, "Value"=T4."Motion Module") -> (reference out=w1774:refnum<vi>, error out=w1773:errorcluster)  [unwired: 1 in]
        n1130 = property class="Bool (strict)"(reference=w1770, "Value"=FALSE) -> (reference out=w1768:refnum<vi>, error out=w1769:errorcluster)  [unwired: 1 in]
        n1131 = Close Reference(reference=w1768, error in (no error)=w1769) -> ()  [unwired: 1 out]
        n1132 = Close Reference(reference=w1774, error in (no error)=w1773) -> ()  [unwired: 1 out]
        n1133 = call "DATA ENCRYPT STRING FILE WRITE.vi"("error in (no error)"=w1765, "User Action"="User Selected Back to Module", "main ref"=w1763) -> ("error out"=w1764:errorcluster)  [unwired: 6 in, 1 out]
      }
      frame "SNext" {
        w1778 = FALSE ("Value")
        n1134 = Unbundle By Name(w1779) -> ("Main Screen.Start Test"=w1782:refnum<vi>)
        n1135 = Unbundle By Name(w1779) -> ("Main Screen.STOP"=w1781:refnum<vi>)
        n1136 = Unbundle By Name(w1779) -> ("Environmental control.SNext"=w1791:refnum<vi>)
        n1137 = Unbundle By Name(w1779) -> ("Main Home Screen.GUI"=w1793:refnum<vi>)
        n1138 = property class="Bool (strict)"(reference=w1782, "Visible"=TRUE ("Value"), "Value"=FALSE) -> (reference out=w1776:refnum<vi>, error out=w1783:errorcluster)  [unwired: 1 in]
        n1139 = property class="Bool (strict)"(reference=w1781, "Value"=w1778, "Visible"=w1778) -> (reference out=w1775:refnum<vi>, error out=w1780:errorcluster)  [unwired: 1 in]
        n1140 = property class="TabCtl (strict)"(reference=w1793, "Value"=T4."Begin") -> (reference out=w1795:refnum<vi>, error out=w1794:errorcluster)  [unwired: 1 in]
        n1141 = property class="Bool (strict)"(reference=w1791, "Value"=FALSE) -> (reference out=w1789:refnum<vi>, error out=w1790:errorcluster)  [unwired: 1 in]
        n1142 = Close Reference(reference=w1776, error in (no error)=w1783) -> ()  [unwired: 1 out]
        n1143 = Close Reference(reference=w1775, error in (no error)=w1780) -> ()  [unwired: 1 out]
        n1144 = Close Reference(reference=w1789, error in (no error)=w1790) -> ()  [unwired: 1 out]
        n1145 = Close Reference(reference=w1795, error in (no error)=w1794) -> ()  [unwired: 1 out]
        n1146 = call "DATA ENCRYPT STRING FILE WRITE.vi"("error in (no error)"=w1786, "User Action"="User Pressed Setup", "main ref"=w1779) -> ("error out"=w1785:errorcluster)  [unwired: 6 in, 1 out]
      }
      frame "Enable Platform" {
        n1147 = Unbundle By Name(w1797) -> ("Heave AND Surge.Sequence ID"=w1799:refnum<vi>)
        n1148 = Unbundle By Name(w1797) -> ("Heave AND Surge.Mode Command"=w1823:refnum<vi>)
        n1149 = Unbundle By Name(w1797) -> ("Heave AND Surge.Distance"=w1820:refnum<vi>)
        n1150 = Unbundle By Name(w1797) -> ("Heave AND Surge.SPEED"=w1817:refnum<vi>)
        n1151 = Unbundle By Name(w1797) -> ("Platform Settings.Enable Platform"=w1831:refnum<vi>)
        n1152 = property class="DigNum (strict)"(reference=w1799, "Value"=u16 0) -> (reference out=w1798:refnum<vi>, error out=w1800:errorcluster)  [unwired: 1 in]
        n1153 = property class="DigNum (strict)"(reference=w1820, error in=w1815, "Value"=sgl 0.0) -> (reference out=w1821:refnum<vi>, error out=w1819:errorcluster)
        n1154 = property class="DigNum (strict)"(reference=w1817, error in=w1815, "Value"=sgl 0.0) -> (reference out=w1818:refnum<vi>, error out=w1816:errorcluster)
        n1155 = property class="DigNum (strict)"(reference=w1823, error in=w1815, "Value"=u8 1) -> (reference out=w1822:refnum<vi>, error out=w1824:errorcluster)
        n1156 = Close Reference(reference=w1798, error in (no error)=w1800) -> (error out=w1796:errorcluster)
        n1157 = Close Reference(reference=w1821, error in (no error)=w1819) -> (error out=w1812:errorcluster)
        n1158 = Close Reference(reference=w1818, error in (no error)=w1816) -> (error out=w1811:errorcluster)
        n1159 = Close Reference(reference=w1822, error in (no error)=w1824) -> (error out=w1813:errorcluster)
        n1160 = property class="Bool (strict)"(reference=w1831, "Value"=FALSE) -> (reference out=w1829:refnum<vi>, error out=w1830:errorcluster)  [unwired: 1 in]
        n1161 = Close Reference(reference=w1829, error in (no error)=w1830) -> ()  [unwired: 1 out]
        n1162 = Merge Errors(w1815, w1813, w1812, w1811, w1796) -> (w1814:errorcluster)
        n1163 = call "DATA ENCRYPT STRING FILE WRITE.vi"("error in (no error)"=w1814, "User Action"="User Pressed Enable Platform", "main ref"=w1797) -> ("error out"=w1826:errorcluster)  [unwired: 6 in, 1 out]
        n1164 = call "HEAVE WRITE FGV.vi"("Enum - Menu"=Heave_Write_enum."WRITE", "error in (no error)"=w1826, "main ref"=w1797) -> ("error out"=w1803:errorcluster)  [unwired: 8 in]
        n1165 = Unbundle By Name(w1797) -> ("Heave AND Surge.Read Heave Temp"=w1807:refnum<vi>)
        n1166 = property class="Bool (strict)"(reference=w1807, error in=w1803, "Value"=TRUE) -> (reference out=w1805:refnum<vi>, error out=w1806:errorcluster)
        n1167 = Close Reference(reference=w1805, error in (no error)=w1806) -> (error out=w1802:errorcluster)
      }
      frame "Heave Up main" {
        n1168 = Unbundle By Name(w1832) -> ("Platform Settings.Heave Up main"=w1842:refnum<vi>)
        n1169 = call "Heave Up Main.vi"("error in (no error)"=w1834, "main ref"=w1832) -> ("error out"=w1833:errorcluster)  [unwired: 9 in]
        n1170 = property class="Bool (strict)"(reference=w1842, "Value"=FALSE) -> (reference out=w1840:refnum<vi>, error out=w1841:errorcluster)  [unwired: 1 in]
        n1171 = Close Reference(reference=w1840, error in (no error)=w1841) -> ()  [unwired: 1 out]
        n1172 = call "DATA ENCRYPT STRING FILE WRITE.vi"("error in (no error)"=w1833, "User Action"="User Pressed Heave UP", "main ref"=w1832) -> ("error out"=w1837:errorcluster)  [unwired: 6 in, 1 out]
        n1173 = call "HEAVE WRITE FGV.vi"("Enum - Menu"=Heave_Write_enum."WRITE", "error in (no error)"=w1837, "main ref"=w1832) -> ("error out"=w1836:errorcluster)  [unwired: 8 in]
      }
      frame "Heave Down Main" {
        n1174 = call "Heave Down Main.vi"("error in (no error)"=w1845, "main ref"=w1843) -> ("error out"=w1844:errorcluster)  [unwired: 9 in]
        n1175 = Unbundle By Name(w1843) -> ("Platform Settings.Heave Down Main"=w1853:refnum<vi>)
        n1176 = property class="Bool (strict)"(reference=w1853, "Value"=FALSE) -> (reference out=w1851:refnum<vi>, error out=w1852:errorcluster)  [unwired: 1 in]
        n1177 = Close Reference(reference=w1851, error in (no error)=w1852) -> ()  [unwired: 1 out]
        n1178 = call "DATA ENCRYPT STRING FILE WRITE.vi"("error in (no error)"=w1844, "User Action"="User Pressed Heave DOWN", "main ref"=w1843) -> ("error out"=w1848:errorcluster)  [unwired: 6 in, 1 out]
        n1179 = call "HEAVE WRITE FGV.vi"("Enum - Menu"=Heave_Write_enum."WRITE", "error in (no error)"=w1848, "main ref"=w1843) -> ("error out"=w1847:errorcluster)  [unwired: 8 in]
      }
      frame "Surge Backward Main" {
        n1180 = Unbundle By Name(w1854) -> ("Platform Settings.Surge Backward Main"=w1864:refnum<vi>)
        n1181 = call "Surge Backward Main.vi"("error in (no error)"=w1856, "main ref"=w1854) -> ("error out"=w1855:errorcluster)  [unwired: 9 in]
        n1182 = property class="Bool (strict)"(reference=w1864, "Value"=FALSE) -> (reference out=w1862:refnum<vi>, error out=w1863:errorcluster)  [unwired: 1 in]
        n1183 = Close Reference(reference=w1862, error in (no error)=w1863) -> ()  [unwired: 1 out]
        n1184 = call "DATA ENCRYPT STRING FILE WRITE.vi"("error in (no error)"=w1855, "User Action"="User Pressed Surge Backward", "main ref"=w1854) -> ("error out"=w1859:errorcluster)  [unwired: 6 in, 1 out]
        n1185 = call "HEAVE WRITE FGV.vi"("Enum - Menu"=Heave_Write_enum."WRITE", "error in (no error)"=w1859, "main ref"=w1854) -> ("error out"=w1858:errorcluster)  [unwired: 8 in]
      }
      frame "Surge Forward Main" {
        n1186 = Unbundle By Name(w1865) -> ("Platform Settings.Surge Forward Main"=w1875:refnum<vi>)
        n1187 = call "Surge Forward Main.vi"("error in (no error)"=w1867, "main ref"=w1865) -> ("error out"=w1866:errorcluster)  [unwired: 9 in]
        n1188 = property class="Bool (strict)"(reference=w1875, "Value"=FALSE) -> (reference out=w1873:refnum<vi>, error out=w1874:errorcluster)  [unwired: 1 in]
        n1189 = Close Reference(reference=w1873, error in (no error)=w1874) -> ()  [unwired: 1 out]
        n1190 = call "DATA ENCRYPT STRING FILE WRITE.vi"("error in (no error)"=w1866, "User Action"="User Pressed Surge Forward", "main ref"=w1865) -> ("error out"=w1870:errorcluster)  [unwired: 6 in, 1 out]
        n1191 = call "HEAVE WRITE FGV.vi"("Enum - Menu"=Heave_Write_enum."WRITE", "error in (no error)"=w1870, "main ref"=w1865) -> ("error out"=w1869:errorcluster)  [unwired: 8 in]
      }
      frame "Manual Write Heave & Surge" {
        n1192 = Unbundle By Name(w1876) -> ("Heave AND Surge.Manual Write"=w1885:refnum<vi>)
        n1193 = property class="Bool (strict)"(reference=w1885, "Value"=FALSE) -> (reference out=w1883:refnum<vi>, error out=w1884:errorcluster)  [unwired: 1 in]
        n1194 = Close Reference(reference=w1883, error in (no error)=w1884) -> ()  [unwired: 1 out]
        n1195 = call "DATA ENCRYPT STRING FILE WRITE.vi"("error in (no error)"=w1877, "User Action"="User Pressed Manual Write Heave and Surge", "main ref"=w1876) -> ("error out"=w1880:errorcluster)  [unwired: 6 in, 1 out]
        n1196 = call "HEAVE WRITE FGV.vi"("Enum - Menu"=Heave_Write_enum."WRITE", "error in (no error)"=w1880, "main ref"=w1876) -> ("error out"=w1879:errorcluster)  [unwired: 8 in]
      }
      frame "Load En" {
        n1197 = Unbundle By Name(w1887) -> ("Main Screen.Load En"=w1892:refnum<vi>)
        n1198 = property class="Bool (strict)"(reference=w1892) -> (reference out=w1890:refnum<vi>, error out=w1891:errorcluster, "Value"=w1886:bool)  [unwired: 1 in]
        n1199 = Close Reference(reference=w1890, error in (no error)=w1891) -> ()  [unwired: 1 out]
        n1200 = case shown="False" w1886 {
          tunnel: [w1899 w1906] -> w1888
          tunnel: w1889 -> [w1902 w1905]
          tunnel: w1887 -> [w1901 w1904]
          tunnel: w1887 -> [w1896 _]
          tunnel: w1887 -> [w1895 _]
          frame False {
            n1201 = call "DATA ENCRYPT STRING FILE WRITE.vi"("error in (no error)"=w1902, "User Action"="User Pressed UnLoad on Main Screen", "main ref"=w1901) -> ("error out"=w1898:errorcluster)  [unwired: 6 in, 1 out]
            n1202 = call "Stall Data Flow.vim"("value in"=w1898, "milliseconds to wait"=u32 2000) -> ("value out"=w1894:errorcluster)  [unwired: 1 out]
            n1203 = call "PID UNLOAD.vi"("error in (no error)"=w1894, "main ref"=w1895) -> ("error out"=w1897:errorcluster)  [unwired: 9 in]
            n1204 = call "HEAVE WRITE FGV.vi"("Enum - Menu"=Heave_Write_enum."WRITE", "error in (no error)"=w1897, "main ref"=w1896) -> ("error out"=w1899:errorcluster)  [unwired: 8 in]
          }
          frame True {
            n1205 = call "DATA ENCRYPT STRING FILE WRITE.vi"("error in (no error)"=w1905, "User Action"="User Pressed Load on Main Screen", "main ref"=w1904) -> ("error out"=w1906:errorcluster)  [unwired: 6 in, 1 out]
          }
        }
      }
      frame "apply load" {
        n1206 = Unbundle By Name(w1909) -> ("Main Screen.Load En"=w1914:refnum<vi>)
        n1207 = property class="Bool (strict)"(reference=w1914) -> (reference out=w1912:refnum<vi>, error out=w1913:errorcluster, "Value"=w1908:bool)  [unwired: 1 in]
        n1208 = Close Reference(reference=w1912, error in (no error)=w1913) -> ()  [unwired: 1 out]
        n1209 = case shown="False" w1908 {
          tunnel: [w1921 w1928] -> w1910
          tunnel: w1911 -> [w1924 w1927]
          tunnel: w1909 -> [w1923 w1926]
          tunnel: w1909 -> [w1918 _]
          tunnel: w1909 -> [w1917 _]
          frame False {
            n1210 = call "DATA ENCRYPT STRING FILE WRITE.vi"("error in (no error)"=w1924, "User Action"="User Pressed UnLoad on Service Screen", "main ref"=w1923) -> ("error out"=w1920:errorcluster)  [unwired: 6 in, 1 out]
            n1211 = call "Stall Data Flow.vim"("value in"=w1920, "milliseconds to wait"=u32 2000) -> ("value out"=w1916:errorcluster)  [unwired: 1 out]
            n1212 = call "PID UNLOAD.vi"("error in (no error)"=w1916, "main ref"=w1917) -> ("error out"=w1919:errorcluster)  [unwired: 9 in]
            n1213 = call "HEAVE WRITE FGV.vi"("Enum - Menu"=Heave_Write_enum."WRITE", "error in (no error)"=w1919, "main ref"=w1918) -> ("error out"=w1921:errorcluster)  [unwired: 8 in]
          }
          frame True {
            n1214 = call "DATA ENCRYPT STRING FILE WRITE.vi"("error in (no error)"=w1927, "User Action"="User Pressed Load on Service Screen", "main ref"=w1926) -> ("error out"=w1928:errorcluster)  [unwired: 6 in, 1 out]
          }
        }
      }
      frame "BACK" {
        w1934 = FALSE ("Value")
        n1215 = Unbundle By Name(w1930) -> ("Main Screen.BACK"=w1954:refnum<vi>)
        n1216 = property class="Bool (strict)"(reference=w1954, "Value"=FALSE) -> (reference out=w1952:refnum<vi>, error out=w1953:errorcluster)  [unwired: 1 in]
        n1217 = Close Reference(reference=w1952, error in (no error)=w1953) -> ()  [unwired: 1 out]
        n1218 = call "DATA ENCRYPT STRING FILE WRITE.vi"("error in (no error)"=w1951, "User Action"="User Pressed Back on Main Screen", "main ref"=w1930) -> ("error out"=w1949:errorcluster)  [unwired: 6 in, 1 out]
        n1219 = Unbundle By Name(w1930) -> ("Main Home Screen.MainPage"=w1941:refnum<vi>)
        n1220 = Unbundle By Name(w1930) -> ("Main Screen.Start Test"=w1937:refnum<vi>)
        n1221 = Unbundle By Name(w1930) -> ("Main Screen.STOP"=w1936:refnum<vi>)
        n1222 = Unbundle By Name(w1930) -> ("Main Home Screen.GUI"=w1945:refnum<vi>)
        n1223 = property class="TabCtl (strict)"(reference=w1941, "Value"=T5."HOME") -> (reference out=w1943:refnum<vi>, error out=w1942:errorcluster)  [unwired: 1 in]
        n1224 = property class="TabCtl (strict)"(reference=w1945, "Value"=T4."Setup") -> (reference out=w1947:refnum<vi>, error out=w1946:errorcluster)  [unwired: 1 in]
        n1225 = property class="Bool (strict)"(reference=w1937, "Visible"=TRUE ("Value"), "Value"=FALSE) -> (reference out=w1932:refnum<vi>, error out=w1938:errorcluster)  [unwired: 1 in]
        n1226 = property class="Bool (strict)"(reference=w1936, "Value"=w1934, "Visible"=w1934) -> (reference out=w1931:refnum<vi>, error out=w1935:errorcluster)  [unwired: 1 in]
        n1227 = Close Reference(reference=w1947, error in (no error)=w1946) -> ()  [unwired: 1 out]
        n1228 = Close Reference(reference=w1943, error in (no error)=w1942) -> ()  [unwired: 1 out]
        n1229 = Close Reference(reference=w1932, error in (no error)=w1938) -> ()  [unwired: 1 out]
        n1230 = Close Reference(reference=w1931, error in (no error)=w1935) -> ()  [unwired: 1 out]
      }
      frame "Start Test" {
        n1231 = call "DATA ENCRYPT STRING FILE WRITE.vi"("error in (no error)"=w1966, "User Action"="User Pressed Start Test on Main Screen", "main ref"=w1955) -> ("error out"=w1964:errorcluster)  [unwired: 6 in, 1 out]
        n1232 = Unbundle By Name(w1955) -> ("Main Screen.Start Test Temp"=w1963:refnum<vi>)
        n1233 = Unbundle By Name(w1955) -> ("Main Screen.Depthz"=w1956:refnum<vi>)
        n1234 = property class="Bool (strict)"(reference=w1956, "Value"=TRUE) -> (reference out=w1958:refnum<vi>, error out=w1957:errorcluster)  [unwired: 1 in]
        n1235 = property class="Bool (strict)"(reference=w1963, "Value"=TRUE) -> (reference out=w1961:refnum<vi>, error out=w1962:errorcluster)  [unwired: 1 in]
        n1236 = Close Reference(reference=w1958, error in (no error)=w1957) -> ()  [unwired: 1 out]
        n1237 = Close Reference(reference=w1961, error in (no error)=w1962) -> ()  [unwired: 1 out]
      }
      frame "STOP" {
        n1238 = call "DATA ENCRYPT STRING FILE WRITE.vi"("error in (no error)"=w1974, "User Action"="User Pressed Stop Test on Main Screen", "main ref"=w1967) -> ("error out"=w1972:errorcluster)  [unwired: 6 in, 1 out]
        n1239 = Unbundle By Name(w1967) -> ("Main Screen.Start Test Temp"=w1971:refnum<vi>)
        n1240 = property class="Bool (strict)"(reference=w1971, "Value"=FALSE) -> (reference out=w1969:refnum<vi>, error out=w1970:errorcluster)  [unwired: 1 in]
        n1241 = Close Reference(reference=w1969, error in (no error)=w1970) -> ()  [unwired: 1 out]
      }
      frame "Error" {
        # "#CodeRecommended - If you ever change the name of this \"Error\" message, you'll need to update the name in the Check Loop Error.vi as well."
        # "#CodeRecommended - Consider creating a system for logging errors in some way. These errors are for notification purposes only. Handling of specific errors should be performed in the message frames that generated the error."
        # "Error - Display an error dialog. This message is sent by the \"Error Handler\" VIs at the end of other loops in this application."
        n1242 = Variant To Data(error in=w1981, type=errorcluster {"status"=FALSE, "code"=0, "source"=""} ("error constant"), Variant=w1979) -> (data=w1977:errorcluster, error out=w1976:errorcluster)
        n1243 = call <vilib>:"Simple Error Handler.vi"("error in (no error)"=w1977) -> ()  [unwired: 4 in, 5 out]
        n1244 = Merge Errors(w1976) -> (w1975:errorcluster)
      }
      frame "Confirm Quit" {
        # "#CodeNeeded - If you want to provide an \"Are you sure\" dialog (or some other notification) before the application exits, place that code here. This message is typically sent from a Panel Close? event."
        # "Confirm Quit - Message that can confirm whether or not the user wants to exit the application."
        n1245 = call-poly "Enqueue Message.vi"("Priority Message? (F)"=TRUE, "error in (no error)"=w1992, "Message"="Exit", "Message Queue"=w1989) -> ("error out"=w1990:errorcluster)  [unwired: 6 in, 1 out]
        n1246 = Merge Errors(w1990) -> (w1991:errorcluster)
        n1247 = call "LOAD CELL FGV MAIN.vi"("Enum"=T16."UNINITIAL", "error in (no error)"=w1991, "main ref"=w1982) -> ("error IO"=w1986:errorcluster)  [unwired: 8 in]
        n1248 = call "LOAD CELL FGV MAIN.vi"("Enum"=T16."DELETEHANDLE", "error in (no error)"=w1986, "main ref"=w1982) -> ("error IO"=w1984:errorcluster)  [unwired: 8 in]
      }
      frame "Exit" {
        # "Stop the VI"
        # "Release the message queue reference"
        # "#CodeNeeded - Add any required cleanup code here. Note that if 'Exit' was called as a result of an error, an error dialog will be displayed. Add any custom error handling for an 'Exit' condition here as well."
        # "Exit - Exit the application."
        n1249 = call "Fire User Event - Stop.vi"("User Event - Stop"=w1995) -> ("error out"=w1994:errorcluster)  [unwired: 10 in]
        n1250 = Release Queue(queue=w2000, error in (no error)=w1993) -> (error out=w1997:errorcluster)  [unwired: 1 in, 2 out]
        n1251 = Merge Errors(w1994, w1997) -> (w1996:errorcluster)
      }
      frame Default {
        # "'Default' case only runs if there is a message that isn't defined in any of the other cases.  Output a programming error."
        n1252 = xnode "Error Ring"("parameter 0"=w2001) -> ("error out"=w2002:errorcluster)
      }
    }
    n1253 = call "LAB-IQ Error Handler - Message Handling Loop.vi"("error in (no error)"=w1062, "Message Queue"=w1064) -> ("dup error in"=w1063:errorcluster)  [unwired: 8 in, 1 out]
  }
  n1254 = while {
    shift-right: [w2021] -> _
    shift-left: w7 -> [w2022]
    tunnel: [w2015] -> w37
    tunnel: w36 -> [w2013]
    tunnel: w14 -> [w2012]
    tunnel: w26 -> [w2011]
    stop <- w2020 stop-if-true
    # "Load  Handling Loop"
    n1255 = call "Dequeue Message.vi"("error in (no error)"=w2012, "Message Queue"=w2013) -> ("error out"=w2019:errorcluster, "Message Data"=w2017:variant, "Message"=w2018:string, "dup Message Queue"=w2016:refnum<queue>)  [unwired: 6 in]
    n1256 = case "Message Cases" shown="\"Load Main\"" w2018 {
      selector: w2018 -> [_ _ _ _ _ w2067]
      tunnel: w2016 -> [w2023 w2035 _ w2054 w2066 _]
      tunnel: w2019 -> [w2026 w2033 w2051 w2058 w2060 _]
      tunnel: [w2027 w2036 w2045 w2056 w2062 w2068] -> w2014
      tunnel: w2022 -> [w2025 w2028 w2050 w2057 w2065 w2069]
      tunnel: [w2025 w2028 w2050 w2057 w2065 w2069] -> w2021
      tunnel: [_ _ _ _ TRUE _] -> w2020
      tunnel: w2017 -> [_ _ w2049 _ _ _]
      tunnel: w2011 -> [_ _ _ _ w2059 _]
      frame "init" {
        # "Bundle control references and a sample string value."
        # "Initialize - All initialization work should take place in this message, since other loops can potentially enqueue messages that execute immediately after this one."
        n1257 = call-poly "Enqueue Message.vi"("error in (no error)"=w2026, "Message"="Load Main", "Message Queue"=w2023) -> ("error out"=w2027:errorcluster)  [unwired: 7 in, 1 out]
      }
      frame "Load Main" {
        n1258 = call "LOAD CELL READ.vi"("error in (no error)"=w2033, "main ref"=w2028) -> ("error out"=w2029:errorcluster)  [unwired: 9 in]
        n1259 = Unbundle By Name(w2028) -> ("Main Home Screen.EXIT"=w2034:refnum<vi>)
        n1260 = property class="Bool (strict)"(reference=w2034) -> (reference out=w2031:refnum<vi>, error out=w2032:errorcluster, "Value"=w2030:bool)  [unwired: 1 in]
        n1261 = Close Reference(reference=w2031, error in (no error)=w2032) -> ()  [unwired: 1 out]
        n1262 = case shown="False" w2030 {
          tunnel: [w2039 w2043] -> w2036
          tunnel: w2035 -> [w2038 w2042]
          tunnel: w2029 -> [w2037 w2041]
          frame True {
            n1263 = call-poly "Enqueue Message.vi"("error in (no error)"=w2037, "Message"="Confirm Quit", "Message Queue"=w2038) -> ("error out"=w2039:errorcluster)  [unwired: 7 in, 1 out]
          }
          frame False {
            n1264 = call-poly "Enqueue Message.vi"("error in (no error)"=w2041, "Message"="Load Main", "Message Queue"=w2042) -> ("error out"=w2043:errorcluster)  [unwired: 7 in, 1 out]
          }
        }
      }
      frame "Error" {
        # "#CodeRecommended - If you ever change the name of this \"Error\" message, you'll need to update the name in the Check Loop Error.vi as well."
        # "#CodeRecommended - Consider creating a system for logging errors in some way. These errors are for notification purposes only. Handling of specific errors should be performed in the message frames that generated the error."
        # "Error - Display an error dialog. This message is sent by the \"Error Handler\" VIs at the end of other loops in this application."
        n1265 = Variant To Data(error in=w2051, type=errorcluster {"status"=FALSE, "code"=0, "source"=""} ("error constant"), Variant=w2049) -> (data=w2047:errorcluster, error out=w2046:errorcluster)
        n1266 = call <vilib>:"Simple Error Handler.vi"("error in (no error)"=w2047) -> ()  [unwired: 4 in, 5 out]
        n1267 = Merge Errors(w2046) -> (w2045:errorcluster)
      }
      frame "Confirm Quit" {
        # "#CodeNeeded - If you want to provide an \"Are you sure\" dialog (or some other notification) before the application exits, place that code here. This message is typically sent from a Panel Close? event."
        # "Confirm Quit - Message that can confirm whether or not the user wants to exit the application."
        n1268 = call-poly "Enqueue Message.vi"("Priority Message? (F)"=TRUE, "error in (no error)"=w2058, "Message"="Exit", "Message Queue"=w2054) -> ("error out"=w2055:errorcluster)  [unwired: 6 in, 1 out]
        n1269 = Merge Errors(w2055) -> (w2056:errorcluster)
      }
      frame "Exit" {
        # "Stop the VI"
        # "Release the message queue reference"
        # "#CodeNeeded - Add any required cleanup code here. Note that if 'Exit' was called as a result of an error, an error dialog will be displayed. Add any custom error handling for an 'Exit' condition here as well."
        # "Exit - Exit the application."
        n1270 = call "Fire User Event - Stop.vi"("User Event - Stop"=w2059) -> ("error out"=w2061:errorcluster)  [unwired: 10 in]
        n1271 = Release Queue(queue=w2066, error in (no error)=w2060) -> (error out=w2063:errorcluster)  [unwired: 1 in, 2 out]
        n1272 = Merge Errors(w2061, w2063) -> (w2062:errorcluster)
      }
      frame Default {
        # "'Default' case only runs if there is a message that isn't defined in any of the other cases.  Output a programming error."
        n1273 = xnode "Error Ring"("parameter 0"=w2067) -> ("error out"=w2068:errorcluster)
      }
    }
    n1274 = call "LAB-IQ Error Handler - Message Handling Loop.vi"("error in (no error)"=w2014, "Message Queue"=w2016) -> ("dup error in"=w2015:errorcluster)  [unwired: 8 in, 1 out]
  }
  n1275 = while {
    shift-right: [w2087] -> _
    shift-left: w7 -> [w2088]
    tunnel: [w2081] -> w34
    tunnel: w35 -> [w2079]
    tunnel: w14 -> [w2078]
    tunnel: w26 -> [w2077]
    stop <- w2086 stop-if-true
    # "Sway Motor  Handling Loop"
    n1276 = call "Dequeue Message.vi"("error in (no error)"=w2078, "Message Queue"=w2079) -> ("error out"=w2085:errorcluster, "Message Data"=w2083:variant, "Message"=w2084:string, "dup Message Queue"=w2082:refnum<queue>)  [unwired: 6 in]
    n1277 = case "Message Cases" shown="\"Exit\"" w2084 {
      selector: w2084 -> [_ _ _ _ _ w2132]
      tunnel: w2082 -> [w2089 w2100 _ w2119 w2131 _]
      tunnel: w2085 -> [w2092 w2097 w2116 w2123 w2125 _]
      tunnel: [w2093 w2101 w2110 w2121 w2127 w2133] -> w2080
      tunnel: w2088 -> [w2091 w2099 w2115 w2122 w2130 w2134]
      tunnel: [w2091 w2099 w2115 w2122 w2130 w2134] -> w2087
      tunnel: [_ _ _ _ TRUE _] -> w2086
      tunnel: w2083 -> [_ _ w2114 _ _ _]
      tunnel: w2077 -> [_ _ _ _ w2124 _]
      frame "init" {
        # "Bundle control references and a sample string value."
        # "Initialize - All initialization work should take place in this message, since other loops can potentially enqueue messages that execute immediately after this one."
        n1278 = call-poly "Enqueue Message.vi"("error in (no error)"=w2092, "Message"="Sway Main", "Message Queue"=w2089) -> ("error out"=w2093:errorcluster)  [unwired: 7 in, 1 out]
      }
      frame "Sway Main" {
        n1279 = Unbundle By Name(w2099) -> ("Main Home Screen.EXIT"=w2098:refnum<vi>)
        n1280 = property class="Bool (strict)"(reference=w2098) -> (reference out=w2095:refnum<vi>, error out=w2096:errorcluster, "Value"=w2094:bool)  [unwired: 1 in]
        n1281 = Close Reference(reference=w2095, error in (no error)=w2096) -> ()  [unwired: 1 out]
        n1282 = case shown="False" w2094 {
          tunnel: [w2104 w2108] -> w2101
          tunnel: w2100 -> [w2103 w2107]
          tunnel: w2097 -> [w2102 w2106]
          frame True {
            n1283 = call-poly "Enqueue Message.vi"("error in (no error)"=w2102, "Message"="Confirm Quit", "Message Queue"=w2103) -> ("error out"=w2104:errorcluster)  [unwired: 7 in, 1 out]
          }
          frame False {
            n1284 = call-poly "Enqueue Message.vi"("error in (no error)"=w2106, "Message"="Sway Main", "Message Queue"=w2107) -> ("error out"=w2108:errorcluster)  [unwired: 7 in, 1 out]
          }
        }
      }
      frame "Error" {
        # "#CodeRecommended - If you ever change the name of this \"Error\" message, you'll need to update the name in the Check Loop Error.vi as well."
        # "#CodeRecommended - Consider creating a system for logging errors in some way. These errors are for notification purposes only. Handling of specific errors should be performed in the message frames that generated the error."
        # "Error - Display an error dialog. This message is sent by the \"Error Handler\" VIs at the end of other loops in this application."
        n1285 = Variant To Data(error in=w2116, type=errorcluster {"status"=FALSE, "code"=0, "source"=""} ("error constant"), Variant=w2114) -> (data=w2112:errorcluster, error out=w2111:errorcluster)
        n1286 = call <vilib>:"Simple Error Handler.vi"("error in (no error)"=w2112) -> ()  [unwired: 4 in, 5 out]
        n1287 = Merge Errors(w2111) -> (w2110:errorcluster)
      }
      frame "Confirm Quit" {
        # "#CodeNeeded - If you want to provide an \"Are you sure\" dialog (or some other notification) before the application exits, place that code here. This message is typically sent from a Panel Close? event."
        # "Confirm Quit - Message that can confirm whether or not the user wants to exit the application."
        n1288 = call-poly "Enqueue Message.vi"("Priority Message? (F)"=TRUE, "error in (no error)"=w2123, "Message"="Exit", "Message Queue"=w2119) -> ("error out"=w2120:errorcluster)  [unwired: 6 in, 1 out]
        n1289 = Merge Errors(w2120) -> (w2121:errorcluster)
      }
      frame "Exit" {
        # "Stop the VI"
        # "Release the message queue reference"
        # "#CodeNeeded - Add any required cleanup code here. Note that if 'Exit' was called as a result of an error, an error dialog will be displayed. Add any custom error handling for an 'Exit' condition here as well."
        # "Exit - Exit the application."
        n1290 = call "Fire User Event - Stop.vi"("User Event - Stop"=w2124) -> ("error out"=w2126:errorcluster)  [unwired: 10 in]
        n1291 = Release Queue(queue=w2131, error in (no error)=w2125) -> (error out=w2128:errorcluster)  [unwired: 1 in, 2 out]
        n1292 = Merge Errors(w2126, w2128) -> (w2127:errorcluster)
      }
      frame Default {
        # "'Default' case only runs if there is a message that isn't defined in any of the other cases.  Output a programming error."
        n1293 = xnode "Error Ring"("parameter 0"=w2132) -> ("error out"=w2133:errorcluster)
      }
    }
    n1294 = call "LAB-IQ Error Handler - Message Handling Loop.vi"("error in (no error)"=w2080, "Message Queue"=w2082) -> ("dup error in"=w2081:errorcluster)  [unwired: 8 in, 1 out]
  }
  n1295 = while {
    shift-right: [w2152] -> _
    shift-left: w7 -> [w2153]
    tunnel: [w2146] -> w31
    tunnel: w33 -> [w2144]
    tunnel: w14 -> [w2143]
    tunnel: w26 -> [w2142]
    stop <- w2151 stop-if-true
    # "Temperature  Handling Loop"
    n1296 = call "Dequeue Message.vi"("error in (no error)"=w2143, "Message Queue"=w2144) -> ("error out"=w2150:errorcluster, "Message Data"=w2148:variant, "Message"=w2149:string, "dup Message Queue"=w2147:refnum<queue>)  [unwired: 6 in]
    n1297 = case "Message Cases" shown="\"Temperature Main\"" w2149 {
      selector: w2149 -> [_ _ _ _ _ w2197]
      tunnel: w2147 -> [w2154 w2165 _ w2184 w2196 _]
      tunnel: w2150 -> [w2157 w2162 w2181 w2188 w2190 _]
      tunnel: [w2158 w2166 w2175 w2186 w2192 w2198] -> w2145
      tunnel: w2153 -> [w2156 w2164 w2180 w2187 w2195 w2199]
      tunnel: [w2156 w2164 w2180 w2187 w2195 w2199] -> w2152
      tunnel: [_ _ _ _ TRUE _] -> w2151
      tunnel: w2148 -> [_ _ w2179 _ _ _]
      tunnel: w2142 -> [_ _ _ _ w2189 _]
      frame "init" {
        # "Initialize - All initialization work should take place in this message, since other loops can potentially enqueue messages that execute immediately after this one."
        n1298 = call-poly "Enqueue Message.vi"("error in (no error)"=w2157, "Message"="Temperature Main", "Message Queue"=w2154) -> ("error out"=w2158:errorcluster)  [unwired: 7 in, 1 out]
      }
      frame "Temperature Main" {
        n1299 = Unbundle By Name(w2164) -> ("Main Home Screen.EXIT"=w2163:refnum<vi>)
        n1300 = property class="Bool (strict)"(reference=w2163) -> (reference out=w2160:refnum<vi>, error out=w2161:errorcluster, "Value"=w2159:bool)  [unwired: 1 in]
        n1301 = case shown="False" w2159 {
          tunnel: [w2169 w2173] -> w2166
          tunnel: w2165 -> [w2168 w2172]
          tunnel: w2162 -> [w2167 w2171]
          frame True {
            n1302 = call-poly "Enqueue Message.vi"("error in (no error)"=w2167, "Message"="Confirm Quit", "Message Queue"=w2168) -> ("error out"=w2169:errorcluster)  [unwired: 7 in, 1 out]
          }
          frame False {
            n1303 = call-poly "Enqueue Message.vi"("error in (no error)"=w2171, "Message"="Temperature Main", "Message Queue"=w2172) -> ("error out"=w2173:errorcluster)  [unwired: 7 in, 1 out]
          }
        }
        n1304 = Close Reference(reference=w2160, error in (no error)=w2161) -> ()  [unwired: 1 out]
      }
      frame "Error" {
        # "#CodeRecommended - If you ever change the name of this \"Error\" message, you'll need to update the name in the Check Loop Error.vi as well."
        # "#CodeRecommended - Consider creating a system for logging errors in some way. These errors are for notification purposes only. Handling of specific errors should be performed in the message frames that generated the error."
        # "Error - Display an error dialog. This message is sent by the \"Error Handler\" VIs at the end of other loops in this application."
        n1305 = Variant To Data(error in=w2181, type=errorcluster {"status"=FALSE, "code"=0, "source"=""} ("error constant"), Variant=w2179) -> (data=w2177:errorcluster, error out=w2176:errorcluster)
        n1306 = call <vilib>:"Simple Error Handler.vi"("error in (no error)"=w2177) -> ()  [unwired: 4 in, 5 out]
        n1307 = Merge Errors(w2176) -> (w2175:errorcluster)
      }
      frame "Confirm Quit" {
        # "#CodeNeeded - If you want to provide an \"Are you sure\" dialog (or some other notification) before the application exits, place that code here. This message is typically sent from a Panel Close? event."
        # "Confirm Quit - Message that can confirm whether or not the user wants to exit the application."
        n1308 = call-poly "Enqueue Message.vi"("Priority Message? (F)"=TRUE, "error in (no error)"=w2188, "Message"="Exit", "Message Queue"=w2184) -> ("error out"=w2185:errorcluster)  [unwired: 6 in, 1 out]
        n1309 = Merge Errors(w2185) -> (w2186:errorcluster)
      }
      frame "Exit" {
        # "Stop the VI"
        # "Release the message queue reference"
        # "#CodeNeeded - Add any required cleanup code here. Note that if 'Exit' was called as a result of an error, an error dialog will be displayed. Add any custom error handling for an 'Exit' condition here as well."
        # "Exit - Exit the application."
        n1310 = call "Fire User Event - Stop.vi"("User Event - Stop"=w2189) -> ("error out"=w2191:errorcluster)  [unwired: 10 in]
        n1311 = Release Queue(queue=w2196, error in (no error)=w2190) -> (error out=w2193:errorcluster)  [unwired: 1 in, 2 out]
        n1312 = Merge Errors(w2191, w2193) -> (w2192:errorcluster)
      }
      frame Default {
        # "'Default' case only runs if there is a message that isn't defined in any of the other cases.  Output a programming error."
        n1313 = xnode "Error Ring"("parameter 0"=w2197) -> ("error out"=w2198:errorcluster)
      }
    }
    n1314 = call "LAB-IQ Error Handler - Message Handling Loop.vi"("error in (no error)"=w2145, "Message Queue"=w2147) -> ("dup error in"=w2146:errorcluster)  [unwired: 8 in, 1 out]
  }
  n1315 = while {
    shift-right: [w2217] -> _
    shift-left: w7 -> [w2218]
    tunnel: [w2211] -> _
    tunnel: w30 -> [w2209]
    tunnel: w14 -> [w2208]
    tunnel: w26 -> [w2207]
    stop <- w2216 stop-if-true
    # "Ramp Motor  Handling Loop"
    n1316 = call "Dequeue Message.vi"("error in (no error)"=w2208, "Message Queue"=w2209) -> ("error out"=w2215:errorcluster, "Message Data"=w2213:variant, "Message"=w2214:string, "dup Message Queue"=w2212:refnum<queue>)  [unwired: 6 in]
    n1317 = case "Message Cases" shown="\"Ramp Main\"" w2214 {
      selector: w2214 -> [_ _ _ _ _ w2262]
      tunnel: w2212 -> [w2219 w2230 _ w2249 w2261 _]
      tunnel: w2215 -> [w2222 w2227 w2246 w2253 w2255 _]
      tunnel: [w2223 w2231 w2240 w2251 w2257 w2263] -> w2210
      tunnel: w2218 -> [w2221 w2229 w2245 w2252 w2260 w2264]
      tunnel: [w2221 w2229 w2245 w2252 w2260 w2264] -> w2217
      tunnel: [_ _ _ _ TRUE _] -> w2216
      tunnel: w2213 -> [_ _ w2244 _ _ _]
      tunnel: w2207 -> [_ _ _ _ w2254 _]
      frame "init" {
        # "Initialize - All initialization work should take place in this message, since other loops can potentially enqueue messages that execute immediately after this one."
        n1318 = call-poly "Enqueue Message.vi"("error in (no error)"=w2222, "Message"="Ramp Main", "Message Queue"=w2219) -> ("error out"=w2223:errorcluster)  [unwired: 7 in, 1 out]
      }
      frame "Ramp Main" {
        n1319 = Unbundle By Name(w2229) -> ("Main Home Screen.EXIT"=w2228:refnum<vi>)
        n1320 = property class="Bool (strict)"(reference=w2228) -> (reference out=w2225:refnum<vi>, error out=w2226:errorcluster, "Value"=w2224:bool)  [unwired: 1 in]
        n1321 = case shown="False" w2224 {
          tunnel: [w2234 w2238] -> w2231
          tunnel: w2230 -> [w2233 w2237]
          tunnel: w2227 -> [w2232 w2236]
          frame True {
            n1322 = call-poly "Enqueue Message.vi"("error in (no error)"=w2232, "Message"="Confirm Quit", "Message Queue"=w2233) -> ("error out"=w2234:errorcluster)  [unwired: 7 in, 1 out]
          }
          frame False {
            n1323 = call-poly "Enqueue Message.vi"("error in (no error)"=w2236, "Message"="Ramp Main", "Message Queue"=w2237) -> ("error out"=w2238:errorcluster)  [unwired: 7 in, 1 out]
          }
        }
        n1324 = Close Reference(reference=w2225, error in (no error)=w2226) -> ()  [unwired: 1 out]
      }
      frame "Error" {
        # "#CodeRecommended - If you ever change the name of this \"Error\" message, you'll need to update the name in the Check Loop Error.vi as well."
        # "#CodeRecommended - Consider creating a system for logging errors in some way. These errors are for notification purposes only. Handling of specific errors should be performed in the message frames that generated the error."
        # "Error - Display an error dialog. This message is sent by the \"Error Handler\" VIs at the end of other loops in this application."
        n1325 = Variant To Data(error in=w2246, type=errorcluster {"status"=FALSE, "code"=0, "source"=""} ("error constant"), Variant=w2244) -> (data=w2242:errorcluster, error out=w2241:errorcluster)
        n1326 = call <vilib>:"Simple Error Handler.vi"("error in (no error)"=w2242) -> ()  [unwired: 4 in, 5 out]
        n1327 = Merge Errors(w2241) -> (w2240:errorcluster)
      }
      frame "Confirm Quit" {
        # "#CodeNeeded - If you want to provide an \"Are you sure\" dialog (or some other notification) before the application exits, place that code here. This message is typically sent from a Panel Close? event."
        # "Confirm Quit - Message that can confirm whether or not the user wants to exit the application."
        n1328 = call-poly "Enqueue Message.vi"("Priority Message? (F)"=TRUE, "error in (no error)"=w2253, "Message"="Exit", "Message Queue"=w2249) -> ("error out"=w2250:errorcluster)  [unwired: 6 in, 1 out]
        n1329 = Merge Errors(w2250) -> (w2251:errorcluster)
      }
      frame "Exit" {
        # "Stop the VI"
        # "Release the message queue reference"
        # "#CodeNeeded - Add any required cleanup code here. Note that if 'Exit' was called as a result of an error, an error dialog will be displayed. Add any custom error handling for an 'Exit' condition here as well."
        # "Exit - Exit the application."
        n1330 = call "Fire User Event - Stop.vi"("User Event - Stop"=w2254) -> ("error out"=w2256:errorcluster)  [unwired: 10 in]
        n1331 = Release Queue(queue=w2261, error in (no error)=w2255) -> (error out=w2258:errorcluster)  [unwired: 1 in, 2 out]
        n1332 = Merge Errors(w2256, w2258) -> (w2257:errorcluster)
      }
      frame Default {
        # "'Default' case only runs if there is a message that isn't defined in any of the other cases.  Output a programming error."
        n1333 = xnode "Error Ring"("parameter 0"=w2262) -> ("error out"=w2263:errorcluster)
      }
    }
    n1334 = call "LAB-IQ Error Handler - Message Handling Loop.vi"("error in (no error)"=w2210, "Message Queue"=w2212) -> ("dup error in"=w2211:errorcluster)  [unwired: 8 in, 1 out]
  }
  n1335 = while {
    shift-right: [w2282] -> _
    shift-left: w7 -> [w2283]
    tunnel: [w2276] -> _
    tunnel: w29 -> [w2274]
    tunnel: w14 -> [w2273]
    tunnel: w26 -> [w2272]
    stop <- w2281 stop-if-true
    # "ECR  Handling Loop"
    n1336 = call "Dequeue Message.vi"("error in (no error)"=w2273, "Message Queue"=w2274) -> ("error out"=w2280:errorcluster, "Message Data"=w2278:variant, "Message"=w2279:string, "dup Message Queue"=w2277:refnum<queue>)  [unwired: 6 in]
    n1337 = case "Message Cases" shown="\"ECR Main\"" w2279 {
      selector: w2279 -> [_ _ _ _ _ w2327]
      tunnel: w2277 -> [w2284 w2295 _ w2314 w2326 _]
      tunnel: w2280 -> [w2287 w2292 w2311 w2318 w2320 _]
      tunnel: [w2288 w2296 w2305 w2316 w2322 w2328] -> w2275
      tunnel: w2283 -> [w2286 w2294 w2310 w2317 w2325 w2329]
      tunnel: [w2286 w2294 w2310 w2317 w2325 w2329] -> w2282
      tunnel: [_ _ _ _ TRUE _] -> w2281
      tunnel: w2278 -> [_ _ w2309 _ _ _]
      tunnel: w2272 -> [_ _ _ _ w2319 _]
      frame "init" {
        # "Initialize - All initialization work should take place in this message, since other loops can potentially enqueue messages that execute immediately after this one."
        n1338 = call-poly "Enqueue Message.vi"("error in (no error)"=w2287, "Message"="ECR Main", "Message Queue"=w2284) -> ("error out"=w2288:errorcluster)  [unwired: 7 in, 1 out]
      }
      frame "ECR Main" {
        n1339 = Unbundle By Name(w2294) -> ("Main Home Screen.EXIT"=w2293:refnum<vi>)
        n1340 = property class="Bool (strict)"(reference=w2293) -> (reference out=w2290:refnum<vi>, error out=w2291:errorcluster, "Value"=w2289:bool)  [unwired: 1 in]
        n1341 = case shown="False" w2289 {
          tunnel: [w2299 w2303] -> w2296
          tunnel: w2295 -> [w2298 w2302]
          tunnel: w2292 -> [w2297 w2301]
          frame True {
            n1342 = call-poly "Enqueue Message.vi"("error in (no error)"=w2297, "Message"="Confirm Quit", "Message Queue"=w2298) -> ("error out"=w2299:errorcluster)  [unwired: 7 in, 1 out]
          }
          frame False {
            n1343 = call-poly "Enqueue Message.vi"("error in (no error)"=w2301, "Message"="ECR Main", "Message Queue"=w2302) -> ("error out"=w2303:errorcluster)  [unwired: 7 in, 1 out]
          }
        }
        n1344 = Close Reference(reference=w2290, error in (no error)=w2291) -> ()  [unwired: 1 out]
      }
      frame "Error" {
        # "#CodeRecommended - If you ever change the name of this \"Error\" message, you'll need to update the name in the Check Loop Error.vi as well."
        # "#CodeRecommended - Consider creating a system for logging errors in some way. These errors are for notification purposes only. Handling of specific errors should be performed in the message frames that generated the error."
        # "Error - Display an error dialog. This message is sent by the \"Error Handler\" VIs at the end of other loops in this application."
        n1345 = Variant To Data(error in=w2311, type=errorcluster {"status"=FALSE, "code"=0, "source"=""} ("error constant"), Variant=w2309) -> (data=w2307:errorcluster, error out=w2306:errorcluster)
        n1346 = call <vilib>:"Simple Error Handler.vi"("error in (no error)"=w2307) -> ()  [unwired: 4 in, 5 out]
        n1347 = Merge Errors(w2306) -> (w2305:errorcluster)
      }
      frame "Confirm Quit" {
        # "#CodeNeeded - If you want to provide an \"Are you sure\" dialog (or some other notification) before the application exits, place that code here. This message is typically sent from a Panel Close? event."
        # "Confirm Quit - Message that can confirm whether or not the user wants to exit the application."
        n1348 = call-poly "Enqueue Message.vi"("Priority Message? (F)"=TRUE, "error in (no error)"=w2318, "Message"="Exit", "Message Queue"=w2314) -> ("error out"=w2315:errorcluster)  [unwired: 6 in, 1 out]
        n1349 = Merge Errors(w2315) -> (w2316:errorcluster)
      }
      frame "Exit" {
        # "Stop the VI"
        # "Release the message queue reference"
        # "#CodeNeeded - Add any required cleanup code here. Note that if 'Exit' was called as a result of an error, an error dialog will be displayed. Add any custom error handling for an 'Exit' condition here as well."
        # "Exit - Exit the application."
        n1350 = call "Fire User Event - Stop.vi"("User Event - Stop"=w2319) -> ("error out"=w2321:errorcluster)  [unwired: 10 in]
        n1351 = Release Queue(queue=w2326, error in (no error)=w2320) -> (error out=w2323:errorcluster)  [unwired: 1 in, 2 out]
        n1352 = Merge Errors(w2321, w2323) -> (w2322:errorcluster)
      }
      frame Default {
        # "'Default' case only runs if there is a message that isn't defined in any of the other cases.  Output a programming error."
        n1353 = xnode "Error Ring"("parameter 0"=w2327) -> ("error out"=w2328:errorcluster)
      }
    }
    n1354 = call "LAB-IQ Error Handler - Message Handling Loop.vi"("error in (no error)"=w2275, "Message Queue"=w2277) -> ("dup error in"=w2276:errorcluster)  [unwired: 8 in, 1 out]
  }
  n1355 = while {
    shift-right: [w2347] -> _
    shift-left: w7 -> [w2348]
    tunnel: [w2341] -> _
    tunnel: w28 -> [w2339]
    tunnel: w14 -> [w2338]
    tunnel: w26 -> [w2337]
    stop <- w2346 stop-if-true
    # "Humidity  Handling Loop"
    n1356 = call "Dequeue Message.vi"("error in (no error)"=w2338, "Message Queue"=w2339) -> ("error out"=w2345:errorcluster, "Message Data"=w2343:variant, "Message"=w2344:string, "dup Message Queue"=w2342:refnum<queue>)  [unwired: 6 in]
    n1357 = case "Message Cases" shown="\"Humidity Main\"" w2344 {
      selector: w2344 -> [_ _ _ _ _ w2392]
      tunnel: w2342 -> [w2349 w2360 _ w2379 w2391 _]
      tunnel: w2345 -> [w2352 w2357 w2376 w2383 w2385 _]
      tunnel: [w2353 w2361 w2370 w2381 w2387 w2393] -> w2340
      tunnel: w2348 -> [w2351 w2359 w2375 w2382 w2390 w2394]
      tunnel: [w2351 w2359 w2375 w2382 w2390 w2394] -> w2347
      tunnel: [_ _ _ _ TRUE _] -> w2346
      tunnel: w2343 -> [_ _ w2374 _ _ _]
      tunnel: w2337 -> [_ _ _ _ w2384 _]
      frame "init" {
        # "Initialize - All initialization work should take place in this message, since other loops can potentially enqueue messages that execute immediately after this one."
        n1358 = call-poly "Enqueue Message.vi"("error in (no error)"=w2352, "Message"="Humidity Main", "Message Queue"=w2349) -> ("error out"=w2353:errorcluster)  [unwired: 7 in, 1 out]
      }
      frame "Humidity Main" {
        n1359 = Unbundle By Name(w2359) -> ("Main Home Screen.EXIT"=w2358:refnum<vi>)
        n1360 = property class="Bool (strict)"(reference=w2358) -> (reference out=w2355:refnum<vi>, error out=w2356:errorcluster, "Value"=w2354:bool)  [unwired: 1 in]
        n1361 = case shown="False" w2354 {
          tunnel: [w2364 w2368] -> w2361
          tunnel: w2360 -> [w2363 w2367]
          tunnel: w2357 -> [w2362 w2366]
          frame True {
            n1362 = call-poly "Enqueue Message.vi"("error in (no error)"=w2362, "Message"="Confirm Quit", "Message Queue"=w2363) -> ("error out"=w2364:errorcluster)  [unwired: 7 in, 1 out]
          }
          frame False {
            n1363 = call-poly "Enqueue Message.vi"("error in (no error)"=w2366, "Message"="Humidity Main", "Message Queue"=w2367) -> ("error out"=w2368:errorcluster)  [unwired: 7 in, 1 out]
          }
        }
        n1364 = Close Reference(reference=w2355, error in (no error)=w2356) -> ()  [unwired: 1 out]
      }
      frame "Error" {
        # "#CodeRecommended - If you ever change the name of this \"Error\" message, you'll need to update the name in the Check Loop Error.vi as well."
        # "#CodeRecommended - Consider creating a system for logging errors in some way. These errors are for notification purposes only. Handling of specific errors should be performed in the message frames that generated the error."
        # "Error - Display an error dialog. This message is sent by the \"Error Handler\" VIs at the end of other loops in this application."
        n1365 = Variant To Data(error in=w2376, type=errorcluster {"status"=FALSE, "code"=0, "source"=""} ("error constant"), Variant=w2374) -> (data=w2372:errorcluster, error out=w2371:errorcluster)
        n1366 = call <vilib>:"Simple Error Handler.vi"("error in (no error)"=w2372) -> ()  [unwired: 4 in, 5 out]
        n1367 = Merge Errors(w2371) -> (w2370:errorcluster)
      }
      frame "Confirm Quit" {
        # "#CodeNeeded - If you want to provide an \"Are you sure\" dialog (or some other notification) before the application exits, place that code here. This message is typically sent from a Panel Close? event."
        # "Confirm Quit - Message that can confirm whether or not the user wants to exit the application."
        n1368 = call-poly "Enqueue Message.vi"("Priority Message? (F)"=TRUE, "error in (no error)"=w2383, "Message"="Exit", "Message Queue"=w2379) -> ("error out"=w2380:errorcluster)  [unwired: 6 in, 1 out]
        n1369 = Merge Errors(w2380) -> (w2381:errorcluster)
      }
      frame "Exit" {
        # "Stop the VI"
        # "Release the message queue reference"
        # "#CodeNeeded - Add any required cleanup code here. Note that if 'Exit' was called as a result of an error, an error dialog will be displayed. Add any custom error handling for an 'Exit' condition here as well."
        # "Exit - Exit the application."
        n1370 = call "Fire User Event - Stop.vi"("User Event - Stop"=w2384) -> ("error out"=w2386:errorcluster)  [unwired: 10 in]
        n1371 = Release Queue(queue=w2391, error in (no error)=w2385) -> (error out=w2388:errorcluster)  [unwired: 1 in, 2 out]
        n1372 = Merge Errors(w2386, w2388) -> (w2387:errorcluster)
      }
      frame Default {
        # "'Default' case only runs if there is a message that isn't defined in any of the other cases.  Output a programming error."
        n1373 = xnode "Error Ring"("parameter 0"=w2392) -> ("error out"=w2393:errorcluster)
      }
    }
    n1374 = call "LAB-IQ Error Handler - Message Handling Loop.vi"("error in (no error)"=w2340, "Message Queue"=w2342) -> ("dup error in"=w2341:errorcluster)  [unwired: 8 in, 1 out]
  }
  n1375 = while {
    shift-right: [w2412] -> _
    shift-left: w7 -> [w2413]
    tunnel: [w2406] -> _
    tunnel: w27 -> [w2404]
    tunnel: w14 -> [w2403]
    tunnel: w26 -> [w2402]
    stop <- w2411 stop-if-true
    # "Program  Handling Loop"
    n1376 = call "Dequeue Message.vi"("error in (no error)"=w2403, "Message Queue"=w2404) -> ("error out"=w2410:errorcluster, "Message Data"=w2408:variant, "Message"=w2409:string, "dup Message Queue"=w2407:refnum<queue>)  [unwired: 6 in]
    n1377 = case "Message Cases" shown="Default" w2409 {
      selector: w2409 -> [_ _ _ _ _ w2457]
      tunnel: w2407 -> [w2414 w2425 _ w2444 w2456 _]
      tunnel: w2410 -> [w2417 w2422 w2441 w2448 w2450 _]
      tunnel: [w2418 w2426 w2435 w2446 w2452 w2458] -> w2405
      tunnel: w2413 -> [w2416 w2424 w2440 w2447 w2455 w2459]
      tunnel: [w2416 w2424 w2440 w2447 w2455 w2459] -> w2412
      tunnel: [_ _ _ _ TRUE _] -> w2411
      tunnel: w2408 -> [_ _ w2439 _ _ _]
      tunnel: w2402 -> [_ _ _ _ w2449 _]
      frame "init" {
        # "Initialize - All initialization work should take place in this message, since other loops can potentially enqueue messages that execute immediately after this one."
        n1378 = call-poly "Enqueue Message.vi"("error in (no error)"=w2417, "Message"="Program Main", "Message Queue"=w2414) -> ("error out"=w2418:errorcluster)  [unwired: 7 in, 1 out]
      }
      frame "Program Main" {
        n1379 = Unbundle By Name(w2424) -> ("Main Home Screen.EXIT"=w2423:refnum<vi>)
        n1380 = property class="Bool (strict)"(reference=w2423) -> (reference out=w2420:refnum<vi>, error out=w2421:errorcluster, "Value"=w2419:bool)  [unwired: 1 in]
        n1381 = case shown="False" w2419 {
          tunnel: [w2429 w2433] -> w2426
          tunnel: w2425 -> [w2428 w2432]
          tunnel: w2422 -> [w2427 w2431]
          frame True {
            n1382 = call-poly "Enqueue Message.vi"("error in (no error)"=w2427, "Message"="Confirm Quit", "Message Queue"=w2428) -> ("error out"=w2429:errorcluster)  [unwired: 7 in, 1 out]
          }
          frame False {
            n1383 = call-poly "Enqueue Message.vi"("error in (no error)"=w2431, "Message"="Program Main", "Message Queue"=w2432) -> ("error out"=w2433:errorcluster)  [unwired: 7 in, 1 out]
          }
        }
        n1384 = Close Reference(reference=w2420, error in (no error)=w2421) -> ()  [unwired: 1 out]
      }
      frame "Error" {
        # "#CodeRecommended - If you ever change the name of this \"Error\" message, you'll need to update the name in the Check Loop Error.vi as well."
        # "#CodeRecommended - Consider creating a system for logging errors in some way. These errors are for notification purposes only. Handling of specific errors should be performed in the message frames that generated the error."
        # "Error - Display an error dialog. This message is sent by the \"Error Handler\" VIs at the end of other loops in this application."
        n1385 = Variant To Data(error in=w2441, type=errorcluster {"status"=FALSE, "code"=0, "source"=""} ("error constant"), Variant=w2439) -> (data=w2437:errorcluster, error out=w2436:errorcluster)
        n1386 = call <vilib>:"Simple Error Handler.vi"("error in (no error)"=w2437) -> ()  [unwired: 4 in, 5 out]
        n1387 = Merge Errors(w2436) -> (w2435:errorcluster)
      }
      frame "Confirm Quit" {
        # "#CodeNeeded - If you want to provide an \"Are you sure\" dialog (or some other notification) before the application exits, place that code here. This message is typically sent from a Panel Close? event."
        # "Confirm Quit - Message that can confirm whether or not the user wants to exit the application."
        n1388 = call-poly "Enqueue Message.vi"("Priority Message? (F)"=TRUE, "error in (no error)"=w2448, "Message"="Exit", "Message Queue"=w2444) -> ("error out"=w2445:errorcluster)  [unwired: 6 in, 1 out]
        n1389 = Merge Errors(w2445) -> (w2446:errorcluster)
      }
      frame "Exit" {
        # "Stop the VI"
        # "Release the message queue reference"
        # "#CodeNeeded - Add any required cleanup code here. Note that if 'Exit' was called as a result of an error, an error dialog will be displayed. Add any custom error handling for an 'Exit' condition here as well."
        # "Exit - Exit the application."
        n1390 = call "Fire User Event - Stop.vi"("User Event - Stop"=w2449) -> ("error out"=w2451:errorcluster)  [unwired: 10 in]
        n1391 = Release Queue(queue=w2456, error in (no error)=w2450) -> (error out=w2453:errorcluster)  [unwired: 1 in, 2 out]
        n1392 = Merge Errors(w2451, w2453) -> (w2452:errorcluster)
      }
      frame Default {
        # "'Default' case only runs if there is a message that isn't defined in any of the other cases.  Output a programming error."
        n1393 = xnode "Error Ring"("parameter 0"=w2457) -> ("error out"=w2458:errorcluster)
      }
    }
    n1394 = call "LAB-IQ Error Handler - Message Handling Loop.vi"("error in (no error)"=w2405, "Message Queue"=w2407) -> ("dup error in"=w2406:errorcluster)  [unwired: 8 in, 1 out]
  }
  n1395 = while {
    shift-right: [w2477] -> _
    shift-left: w7 -> [w2478]
    tunnel: [w2471] -> _
    tunnel: w25 -> [w2469]
    tunnel: w14 -> [w2468]
    tunnel: w26 -> [w2467]
    stop <- w2476 stop-if-true
    # "Monitor  Handling Loop"
    n1396 = call "Dequeue Message.vi"("error in (no error)"=w2468, "Message Queue"=w2469) -> ("error out"=w2475:errorcluster, "Message Data"=w2473:variant, "Message"=w2474:string, "dup Message Queue"=w2472:refnum<queue>)  [unwired: 6 in]
    n1397 = case "Message Cases" shown="\"Monitor Main\"" w2474 {
      selector: w2474 -> [_ _ _ _ _ w2523]
      tunnel: w2472 -> [w2479 w2491 _ w2510 w2522 _]
      tunnel: w2475 -> [w2482 w2489 w2507 w2514 w2516 _]
      tunnel: [w2483 w2492 w2501 w2512 w2518 w2524] -> w2470
      tunnel: w2478 -> [w2481 w2484 w2506 w2513 w2521 w2525]
      tunnel: [w2481 w2484 w2506 w2513 w2521 w2525] -> w2477
      tunnel: [_ _ _ _ TRUE _] -> w2476
      tunnel: w2473 -> [_ _ w2505 _ _ _]
      tunnel: w2467 -> [_ _ _ _ w2515 _]
      frame "init" {
        # "Initialize - All initialization work should take place in this message, since other loops can potentially enqueue messages that execute immediately after this one."
        n1398 = call-poly "Enqueue Message.vi"("error in (no error)"=w2482, "Message"="Monitor Main", "Message Queue"=w2479) -> ("error out"=w2483:errorcluster)  [unwired: 7 in, 1 out]
      }
      frame "Monitor Main" {
        n1399 = call "Main Monitor Loop.vi"("error in (no error)"=w2489, "main ref"=w2484) -> ("error out"=w2485:errorcluster)  [unwired: 9 in]
        n1400 = Unbundle By Name(w2484) -> ("Main Home Screen.EXIT"=w2490:refnum<vi>)
        n1401 = property class="Bool (strict)"(reference=w2490) -> (reference out=w2487:refnum<vi>, error out=w2488:errorcluster, "Value"=w2486:bool)  [unwired: 1 in]
        n1402 = case shown="False" w2486 {
          tunnel: [w2495 w2499] -> w2492
          tunnel: w2491 -> [w2494 w2498]
          tunnel: w2485 -> [w2493 w2497]
          frame True {
            n1403 = call-poly "Enqueue Message.vi"("error in (no error)"=w2493, "Message"="Confirm Quit", "Message Queue"=w2494) -> ("error out"=w2495:errorcluster)  [unwired: 7 in, 1 out]
          }
          frame False {
            n1404 = call-poly "Enqueue Message.vi"("error in (no error)"=w2497, "Message"="Monitor Main", "Message Queue"=w2498) -> ("error out"=w2499:errorcluster)  [unwired: 7 in, 1 out]
          }
        }
        n1405 = Close Reference(reference=w2487, error in (no error)=w2488) -> ()  [unwired: 1 out]
      }
      frame "Error" {
        # "#CodeRecommended - If you ever change the name of this \"Error\" message, you'll need to update the name in the Check Loop Error.vi as well."
        # "#CodeRecommended - Consider creating a system for logging errors in some way. These errors are for notification purposes only. Handling of specific errors should be performed in the message frames that generated the error."
        # "Error - Display an error dialog. This message is sent by the \"Error Handler\" VIs at the end of other loops in this application."
        n1406 = Variant To Data(error in=w2507, type=errorcluster {"status"=FALSE, "code"=0, "source"=""} ("error constant"), Variant=w2505) -> (data=w2503:errorcluster, error out=w2502:errorcluster)
        n1407 = call <vilib>:"Simple Error Handler.vi"("error in (no error)"=w2503) -> ()  [unwired: 4 in, 5 out]
        n1408 = Merge Errors(w2502) -> (w2501:errorcluster)
      }
      frame "Confirm Quit" {
        # "#CodeNeeded - If you want to provide an \"Are you sure\" dialog (or some other notification) before the application exits, place that code here. This message is typically sent from a Panel Close? event."
        # "Confirm Quit - Message that can confirm whether or not the user wants to exit the application."
        n1409 = call-poly "Enqueue Message.vi"("Priority Message? (F)"=TRUE, "error in (no error)"=w2514, "Message"="Exit", "Message Queue"=w2510) -> ("error out"=w2511:errorcluster)  [unwired: 6 in, 1 out]
        n1410 = Merge Errors(w2511) -> (w2512:errorcluster)
      }
      frame "Exit" {
        # "Stop the VI"
        # "Release the message queue reference"
        # "#CodeNeeded - Add any required cleanup code here. Note that if 'Exit' was called as a result of an error, an error dialog will be displayed. Add any custom error handling for an 'Exit' condition here as well."
        # "Exit - Exit the application."
        n1411 = call "Fire User Event - Stop.vi"("User Event - Stop"=w2515) -> ("error out"=w2517:errorcluster)  [unwired: 10 in]
        n1412 = Release Queue(queue=w2522, error in (no error)=w2516) -> (error out=w2519:errorcluster)  [unwired: 1 in, 2 out]
        n1413 = Merge Errors(w2517, w2519) -> (w2518:errorcluster)
      }
      frame Default {
        # "'Default' case only runs if there is a message that isn't defined in any of the other cases.  Output a programming error."
        n1414 = xnode "Error Ring"("parameter 0"=w2523) -> ("error out"=w2524:errorcluster)
      }
    }
    n1415 = call "LAB-IQ Error Handler - Message Handling Loop.vi"("error in (no error)"=w2470, "Message Queue"=w2472) -> ("dup error in"=w2471:errorcluster)  [unwired: 8 in, 1 out]
  }
  n1416 = while {
    shift-right: [w2543] -> _
    shift-left: w7 -> [w2544]
    tunnel: [w2537] -> _
    tunnel: w23 -> [w2535]
    tunnel: w14 -> [w2534]
    tunnel: w26 -> [w2533]
    stop <- w2542 stop-if-true
    # "Report  Handling Loop"
    n1417 = call "Dequeue Message.vi"("error in (no error)"=w2534, "Message Queue"=w2535) -> ("error out"=w2541:errorcluster, "Message Data"=w2539:variant, "Message"=w2540:string, "dup Message Queue"=w2538:refnum<queue>)  [unwired: 6 in]
    n1418 = case "Message Cases" shown="\"Report Main\"" w2540 {
      selector: w2540 -> [_ _ _ _ _ w2588]
      tunnel: w2538 -> [w2545 w2556 _ w2575 w2587 _]
      tunnel: w2541 -> [w2548 w2553 w2572 w2579 w2581 _]
      tunnel: [w2549 w2557 w2566 w2577 w2583 w2589] -> w2536
      tunnel: w2544 -> [w2547 w2555 w2571 w2578 w2586 w2590]
      tunnel: [w2547 w2555 w2571 w2578 w2586 w2590] -> w2543
      tunnel: [_ _ _ _ TRUE _] -> w2542
      tunnel: w2539 -> [_ _ w2570 _ _ _]
      tunnel: w2533 -> [_ _ _ _ w2580 _]
      frame "init" {
        # "Initialize - All initialization work should take place in this message, since other loops can potentially enqueue messages that execute immediately after this one."
        n1419 = call-poly "Enqueue Message.vi"("error in (no error)"=w2548, "Message"="Report Main", "Message Queue"=w2545) -> ("error out"=w2549:errorcluster)  [unwired: 7 in, 1 out]
      }
      frame "Report Main" {
        n1420 = Unbundle By Name(w2555) -> ("Main Home Screen.EXIT"=w2554:refnum<vi>)
        n1421 = property class="Bool (strict)"(reference=w2554) -> (reference out=w2551:refnum<vi>, error out=w2552:errorcluster, "Value"=w2550:bool)  [unwired: 1 in]
        n1422 = case shown="False" w2550 {
          tunnel: [w2560 w2564] -> w2557
          tunnel: w2556 -> [w2559 w2563]
          tunnel: w2553 -> [w2558 w2562]
          frame True {
            n1423 = call-poly "Enqueue Message.vi"("error in (no error)"=w2558, "Message"="Confirm Quit", "Message Queue"=w2559) -> ("error out"=w2560:errorcluster)  [unwired: 7 in, 1 out]
          }
          frame False {
            n1424 = call-poly "Enqueue Message.vi"("error in (no error)"=w2562, "Message"="Report Main", "Message Queue"=w2563) -> ("error out"=w2564:errorcluster)  [unwired: 7 in, 1 out]
          }
        }
        n1425 = Close Reference(reference=w2551, error in (no error)=w2552) -> ()  [unwired: 1 out]
      }
      frame "Error" {
        # "#CodeRecommended - If you ever change the name of this \"Error\" message, you'll need to update the name in the Check Loop Error.vi as well."
        # "#CodeRecommended - Consider creating a system for logging errors in some way. These errors are for notification purposes only. Handling of specific errors should be performed in the message frames that generated the error."
        # "Error - Display an error dialog. This message is sent by the \"Error Handler\" VIs at the end of other loops in this application."
        n1426 = Variant To Data(error in=w2572, type=errorcluster {"status"=FALSE, "code"=0, "source"=""} ("error constant"), Variant=w2570) -> (data=w2568:errorcluster, error out=w2567:errorcluster)
        n1427 = call <vilib>:"Simple Error Handler.vi"("error in (no error)"=w2568) -> ()  [unwired: 4 in, 5 out]
        n1428 = Merge Errors(w2567) -> (w2566:errorcluster)
      }
      frame "Confirm Quit" {
        # "#CodeNeeded - If you want to provide an \"Are you sure\" dialog (or some other notification) before the application exits, place that code here. This message is typically sent from a Panel Close? event."
        # "Confirm Quit - Message that can confirm whether or not the user wants to exit the application."
        n1429 = call-poly "Enqueue Message.vi"("Priority Message? (F)"=TRUE, "error in (no error)"=w2579, "Message"="Exit", "Message Queue"=w2575) -> ("error out"=w2576:errorcluster)  [unwired: 6 in, 1 out]
        n1430 = Merge Errors(w2576) -> (w2577:errorcluster)
      }
      frame "Exit" {
        # "Stop the VI"
        # "Release the message queue reference"
        # "#CodeNeeded - Add any required cleanup code here. Note that if 'Exit' was called as a result of an error, an error dialog will be displayed. Add any custom error handling for an 'Exit' condition here as well."
        # "Exit - Exit the application."
        n1431 = call "Fire User Event - Stop.vi"("User Event - Stop"=w2580) -> ("error out"=w2582:errorcluster)  [unwired: 10 in]
        n1432 = Release Queue(queue=w2587, error in (no error)=w2581) -> (error out=w2584:errorcluster)  [unwired: 1 in, 2 out]
        n1433 = Merge Errors(w2582, w2584) -> (w2583:errorcluster)
      }
      frame Default {
        # "'Default' case only runs if there is a message that isn't defined in any of the other cases.  Output a programming error."
        n1434 = xnode "Error Ring"("parameter 0"=w2588) -> ("error out"=w2589:errorcluster)
      }
    }
    n1435 = call "LAB-IQ Error Handler - Message Handling Loop.vi"("error in (no error)"=w2536, "Message Queue"=w2538) -> ("dup error in"=w2537:errorcluster)  [unwired: 8 in, 1 out]
  }
  n1436 = Unregister For Events(event registration refnum=w61, error in=w59) -> (error out=w62:errorcluster)
  n1437 = while {
    tunnel: w16 -> [w2606]
    tunnel: w9 -> [w2605]
    tunnel: w7 -> [w2600]
    stop <- w2599 stop-if-true
    # "Dequeue Loop"
    n1438 = Unbundle By Name(w2600) -> ("Main Home Screen.EXIT"=w2601:refnum<vi>)
    n1439 = Dequeue Element(queue=w2606, error in (no error)=w2605) -> (element=w2604:string)  [unwired: 4 out]
    "Heave and Surge Read" <- w2604
    n1440 = property class="Bool (strict)"(reference=w2601) -> (reference out=w2603:refnum<vi>, error out=w2602:errorcluster, "Value"=w2599:bool)  [unwired: 1 in]
    n1441 = call "HEAVE READ.vi"("Heave and Surge Read in"=w2604, "Data Cluster"=w2600) -> ()  [unwired: 9 in, 1 out]
    n1442 = local read "seconds to wait"() -> (w2598:dbl)
    n1443 = Close Reference(reference=w2603, error in (no error)=w2602) -> ()  [unwired: 1 out]
    n1444 = call <vilib>:"High Resolution Polling Wait.vi"("seconds to wait"=w2598) -> ()  [unwired: 10 in, 1 out]
  }
  n1445 = while {
    tunnel: w16 -> [w2622]
    tunnel: w6 -> [w2621]
    tunnel: w7 -> [w2611]
    tunnel: w5 -> [w2608]
    tunnel: [w2607] -> _
    stop <- w2615 stop-if-true
    # "Enqueue Loop"
    n1446 = Unbundle By Name(w2611) -> ("Heave AND Surge.Read Heave Temp"=w2614:refnum<vi>)
    n1447 = Unbundle By Name(w2611) -> ("Main Home Screen.EXIT"=w2618:refnum<vi>)
    n1448 = property class="Bool (strict)"(reference=w2614) -> (reference out=w2612:refnum<vi>, error out=w2613:errorcluster, "Value"=w2610:bool)  [unwired: 1 in]
    n1449 = property class="Bool (strict)"(reference=w2618) -> (reference out=w2616:refnum<vi>, error out=w2617:errorcluster, "Value"=w2615:bool)  [unwired: 1 in]
    n1450 = case shown="True" w2610 {
      tunnel: w2621 -> [w2624 w2631]
      tunnel: [w2624 w2635] -> w2620
      tunnel: ["" ("HEAVE OUT") w2634] -> w2619
      tunnel: w2611 -> [_ _]
      tunnel: w2608 -> [w2623 w2629]
      tunnel: [w2623 w2626] -> w2607
      frame False {
      }
      frame True {
        n1451 = UDP Read(connection ID=w2629, max size (548)=100, timeout ms (25000)=-1, 8:w2631) -> (data out=w2628:string, error out=w2630:errorcluster, 3:w2627:refnum<k16>)  [unwired: 2 out]
        n1452 = case shown="No Error" w2630 {
          tunnel: w2630 -> [_ w2648]
          tunnel: [_ w2647] -> w2635
          tunnel: [w2637 w2646] -> w2634
          tunnel: w2628 -> [w2637 w2646]
          tunnel: w2627 -> [w2636 w2639]
          tunnel: [w2636 w2638] -> w2626
          frame No Error {
          }
          frame Error {
            n1453 = call <vilib>:"Clear Errors.vi"("error in (no error)"=w2648) -> ("error out"=w2641:errorcluster)  [unwired: 5 in, 1 out]
            n1454 = UDP Close(connection ID=w2639, 8:w2641) -> (error out=w2645:errorcluster)  [unwired: 1 out]
            n1455 = call "Stall Data Flow.vim"("value in"=w2645, "milliseconds to wait"=u32 1000) -> ("value out"=w2642:errorcluster)  [unwired: 1 out]
            n1456 = UDP Open(8:w2642, 11:u16 8888 ("port")) -> (port=w2638:refnum<k16>, 0:w2640:errorcluster)  [unwired: 3 in, 1 out]
            n1457 = call <vilib>:"Clear Errors.vi"("error in (no error)"=w2640) -> ("error out"=w2647:errorcluster)  [unwired: 5 in, 1 out]
          }
        }
      }
    }
    n1458 = Close Reference(reference=w2612, error in (no error)=w2613) -> ()  [unwired: 1 out]
    n1459 = Close Reference(reference=w2616, error in (no error)=w2617) -> ()  [unwired: 1 out]
    n1460 = call <vilib>:"High Resolution Polling Wait.vi"("seconds to wait"="seconds to wait") -> ()  [unwired: 10 in, 1 out]
    n1461 = Enqueue Element(queue=w2622, element=w2619, error in (no error)=w2620) -> ()  [unwired: 4 out]
  }
  n1462 = Merge Errors(w62, w65, w37, w34, w32, w31) -> (w63:errorcluster)
  n1463 = call "Destroy User Event - Stop.vi"("error in (no error)"=w63, "User Event - Stop"=w26) -> ("error out"=w60:errorcluster)  [unwired: 9 in]
  n1464 = disable-structure shown="RUN_TIME_ENGINE==True" {
    disable-tunnel: w60 -> [_ _]
    frame condition #0 (active) {
    }
    frame condition #1 {
      # "Call Quit LabVIEW if running as a built application."
      n1465 = Quit LabVIEW() -> ()  [unwired: 1 in]
    }
  }
